vi "Utah Core Audio Test.vi"(11 "Module Config":T9={"Name"="Base Station RF Test", "Parent Q"=refnum, "Is Child?"=FALSE, "Index"=0, "Dirs"={"Root"=path "", "Config"=path "C:/ATE/Config", "Logs"=path "C:/ATE/Logs", "Reports"=path "C:/ATE/Reports", "App Data"=path "C:/ProgramData/MAIN"}, "Simulate"=FALSE, "SimCtrl"=refnum}) -> ()   [LabVIEW 2018]
uses:
  <vilib>/KATE/Queues/Queue Utils.lvlib
  <vilib>/KATE/Module/Module Utils.lvlib
  <vilib>/KATE/Module/Window/Window.Task, Action.ctl
  <vilib>/KATE/Event Log/Event Log.lvlib
  <vilib>/KATE/Scheduler/Scheduler.lvlib
  <vilib>/KATE/Menu/Menu Utils.lvlib
  <vilib>/KATE/Status/Status Utils.lvlib
  Common/Utils/Results/Result.Measurement and Attribute Item Status.ctl
  Common/Utils/Results/Result.Attribute.ctl
  Common/Utils/Results/Result.Limit Type.ctl
  Common/Utils/Results/Result.Numeric.ctl
  <vilib>/KATE/Event Log/Event Notification/Event Notification.lvclass
  <vilib>/KATE/Module/Module.SW Version Info.ctl
  <vilib>/KATE/Event Log/Event Notification/Event Log.Notification Type.ctl
  <vilib>/KATE/Event Log/Event Notification/Event Log.Log Level.ctl
  Common/Utils/Results/Result XML/TestResult.SW Item.ctl
  Common/Utils/TestExec/TestExec.WorkingDir.ctl
  <vilib>/KATE/TCP-IP/Mgr/TCP-IP Mgr.Config.ctl
  <vilib>/KATE/TCP-IP/TCP-IP.lvlib
  Common/Utils/TestExec/TestExec.Test Start Message to Sta.ctl
  <vilib>/KATE/Files/File Utils.lvlib
  Common/Utils/Errors/Error.Error Code List.ctl
  Common/Utils/TestExec/TestExec.Health State Command.ctl
  Common/Utils/Functions/FunctDataMgr/FunctDataMgr.lvclass
  Common/Utils/Results/Result.Results Table Record.ctl
  <vilib>/KATE/Config/Stored Controls/Class.SaveCtrls.lvclass
  <vilib>/KATE/SeqMgr/SeqMgr.Result State Enum.ctl
  <vilib>/KATE/SeqMgr/SeqMgr.lvlib
  <vilib>/KATE/SeqMgr/SeqMgr.Result Info.ctl
  <vilib>/KATE/Config/App Data/Class.AppData.lvclass
  <vilib>/sound2/lvsound2.llb/Sound Data Format.ctl
  <vilib>/sound2/lvsound2.llb/Sound File Write Open.vi
  <vilib>/addons/_NISVFA/_Generation/Signal Generation/SV Discrete Sweep/SV Discrete Sweep.lvclass
  TypeDefs/AudioTest.Result Plot Data.ctl
  <vilib>/sound2/lvsound2.llb/Sound File Write (DBL Single).vi
  <vilib>/KATE/Time/Time Utils.lvlib
  TypeDefs/AudioTest.Config, Limits, Blocked Mic Check.ctl
  TypeDefs/AudioTest.Config, Average Level Config.ctl
  TypeDefs/AudioTest.Config, Sine Sweep Params_V2.ctl
  TypeDefs/AudioTest.Config, Device ID.ctl
  <vilib>/sound2/lvsound2.llb/Sound Output Set Volume (Single).vi
  <vilib>/sound2/lvsound2.llb/Sound Output Write (DBL Single).vi
  <vilib>/sound2/lvsound2.llb/Sampling Mode.ctl
  Common/Utils/Results/Result.Measurement Item.ctl
  <vilib>/sound2/lvsound2.llb/Sound File Write (DBL).vi
  <vilib>/KATE/Queues/Q.Element.ctl
  <vilib>/KATE/Module/Module Config.ctl
  <vilib>/KATE/Module/Module.Working Dirs.ctl
  <vilib>/Utility/miscctls.llb/LVRectTypeDef.ctl
panel:
  in  "Archive Results":bool
  in  "Main Tab":enum32{"Operate", "Maint"}(tab)
  out "TE":bool
  out "Simulate Indication":string="Simulating Instruments"
  in  "Control Tab":enum32{"Test Control", "Config"}(tab)
  in  "Reload Config":bool
  out "Enumerated":bool
  in  "Check UUT Enum Status":bool
  in  "Timeout(s)":dbl=30.0 caption="Time Out(s)" format="%.2f"
  in  "Get Top SN":bool
  in  "Mode":string="Production"
  in  "Run Sweep":bool
  in  "Init UUT Folder":bool
  out "Start Time":timestamp caption="Start\nTime"
  in  "SN":string="ABC123"
  in  "Clear Errors":bool
  in  "Test Reset":bool
  out "Duration(s)":dbl format="%.2g"
  out "Status":string
  in  "Abort":bool
  in  "Result Data Tab":T1(tab)
  in  "UUT Dir":path caption="UUT Folder"
  in  "Open UUT Dir":bool
  in  "Filter":string
  in  "Show Only Failures":bool
  in  "Auto Scroll":bool=TRUE
  out "Results Table":T2[](array[typedef]) caption="Results"
  out "L AvgMag Delta":dbl caption="Delta" format="%.2f"
  out "L AvgMagUnCov":dbl caption="Uncovered" format="%.2f"
  out "L AvgMagCov":dbl caption="Covered" format="%.2f"
  out "R AvgMag Delta":dbl caption="Delta" format="%.2f"
  out "R AvgMagUnCov":dbl caption="Uncovered" format="%.2f"
  out "R AvgMagCov":dbl caption="Covered" format="%.2f"
  out "Right Mic THD":cluster{"F":dbl[], "M":dbl[]}[](graph) caption="Right THD"
  out "Left Mic THD":cluster{"X":dbl[], "Y":dbl[]}[](graph) caption="Left THD"
  out "Right Freq Response":cluster{"frequency":dbl[], "magnitude":dbl[]}[](graph)
  out "Left Freq Response":cluster{"frequency":dbl[], "magnitude":dbl[]}[](graph)
  out "RtThdColor":u32(colorbox)=13816530
  out "RtFRColor":u32(colorbox)=13816530
  out "LFRColor":u32(colorbox)=13816530
  out "LThdColor":u32(colorbox)=13816530
  in  "Raw Time Plots":enum32{"Time", "Covered Mic Mag"}(tab)
  out "Graph Sine Sweep":waveform(dbl)(graph) caption="Stepped Sine Sweep"
  out "Graph Sine Sweep Cal":waveform(dbl)(graph) caption="Stepped Sine Sweep - Calibrated"
  out "Graph Left Covered":waveform(dbl)(graph)
  out "Graph Left Uncovered":waveform(dbl)(graph)
  out "Graph Right Covered":waveform(dbl)(graph)
  out "Graph Right Uncovered":waveform(dbl)(graph)
  out "Right Mic Covered FR":cluster{"F":dbl[], "M":dbl[]}(graph)
  out "Left Mic Covered FR":cluster{"F":dbl[], "M":dbl[]}(graph)
  out "Measurements":path
  out "Result State File":path
  out "Right Mic Covered Raw":path
  out "Right Mic Raw":path
  out "Left Mic Covered Raw":path
  out "Left Mic Raw":path
  out "Sine Sweep Cal":path
  out "Sine Sweep":path
  in  "Undock FW Util":bool
  out "Test Running":bool
  out "Error":errorcluster
  in  "Mic Test Setup":T3
  in  "Clear Graphs":bool
  in  "Clear Raw Data":bool
  in  "Config Tab":enum32{"Microphone Test Setup", "Misc"}(tab)
  in  "Play Tone":bool
  in  "Tone Freq":dbl=1000.0
  in  "Save Wav Files":bool
  in  "Play Volume":dbl(slide)=50.0 scale=0.0..100.0
  in  "SpeakerCalFile":path=path "C:/MTE/Utah Core Audio Test/Config/Microphone Test Speaker Calibration.ini" caption="Speaker Calibration File"
  in  "Limits":T4={"CoveredMicAttn_dB"=30.0, "AvgLevelLL_dBFS"=-30.0, "AvgLevelUL_dBFS"=-10.0, "FreqRespLim"=path "C:/MTE/Utah Core Audio Test/Config/Microphone Test Freq Response Limits.ini", "THDLim"=path "C:/MTE/Utah Core Audio Test/Config/Microphone Test THD Limits.ini"} caption="Test Limits"
  in  "AvgLevelParams":T5={"Freq Start"=500.0, "Freq End"=1200.0} caption="Average Level Calculation"
  in  "Default Data Folder":path=path "C:/MTE/Utah Core Audio Test/Data"
  in  "Sound Devices":T6={"AudioOutName"="Line", "AudioInName"="HMD"}
  in  "Sine Sweep Params":T7={"Duration"=2.54, "Amplitude"=1.0, "FreqStart"=100.0, "FreqEnd"=20000.0, "SampleRate"=44100.0, "StepCnt"=120, "FreqSpacing"=enum."Logarithmic", "Settling"={"Time"=0.0, "Cycles"=1.0}, "Measurement"={"Time"=0.001, "Cycles"=10.0}, "SyncPulseEn"=TRUE} {"Measurement"."Cycles" min=5.0 max=1000.0 step=1.0; "Measurement"."Time" min=0.0 max=5.0 step=0.0001 format="%.3f s"; "Settling"."Cycles" min=0.0 max=100.0 step=0.5; "Settling"."Time" min=0.0 max=5.0 step=0.0001 format="%.3f s"; "StepCnt" min=1; "Amplitude" min=0.0 max=1.0 step=0.1}
  in  "Input Device":i32(ring) items=["Microphone (2- Valve VR Radio & HMD Mic)"]
  in  "Output Device":i32(ring) items=["Speakers (Realtek High Definition Audio)", "Utah (NVIDIA High Definition Audio)", "DELL U3011 (NVIDIA High Definition Audio)", "Realtek Digital Output (Realtek High Definition Audio)", "Realtek Digital Output(Optical) (Realtek High Definition Audio)"]
  in  "Set Audio Output Device Name":bool
  in  "Set Audio Input Device Name":bool
  in  "Stay Open after CLI":bool
  in  "UUT Data Dir":path=path "C:/MTE/Data/X1"
  in  "Sim CLI at Launch":bool
  in  "Run CLI Simulation":bool
  out "R Delta Color":u32(colorbox)=13816530
  out "L Delta Color":u32(colorbox)=13816530
  out "R Level Color":u32(colorbox)=13816530
  out "L Level Color":u32(colorbox)=13816530
  in  "AddTraceInfo":bool caption="Add Trace Info to Errors"
  out "MicTest Dur(s)":dbl=1.0 format="%.2p"
  out "Args":string[](array[string])
  in  "Select Command Line Args":u16(ring) items=["None", "Sweep Left Covered", "Sweep Right Covered", "Sweep Left Uncovered", "Sweep Right Uncovered"]
  in  "Logging Level":T8
  out "App Run Dur(s)":dbl=1.0 format="%.2p"
  out "PlayDur(s)":dbl=1.0 format="%.2p"
  out "Total Samples":i32
  out "Rev":string="v1.0.0"
  out "Error Status":string
  out "Title":string
  in  "Leave Maint":bool
  in  "New Window Bounds":T11={"Left"=212, "Top"=78, "Right"=1444, "Bottom"=899}
  out "Old Window Bounds":T11={"Left"=2142, "Top"=133, "Right"=3354, "Bottom"=889}
  in  "Set Window Bounds":bool
  # "Step                          Name                                                      Value                                    Units      LimType       LL           UL            Result          Code                     Description"
  # "Avg Level:"
  # "dBFS"
  # "dBFS"
  # "dB"
  # "Avg Level:"
  # "dBFS"
  # "dBFS"
  # "dB"
  # "The selected devices are based on the configured Sound Device name lookup."
  # "Volume Check"
  # "Hz"
  # "Relative to Uncovered Mic"
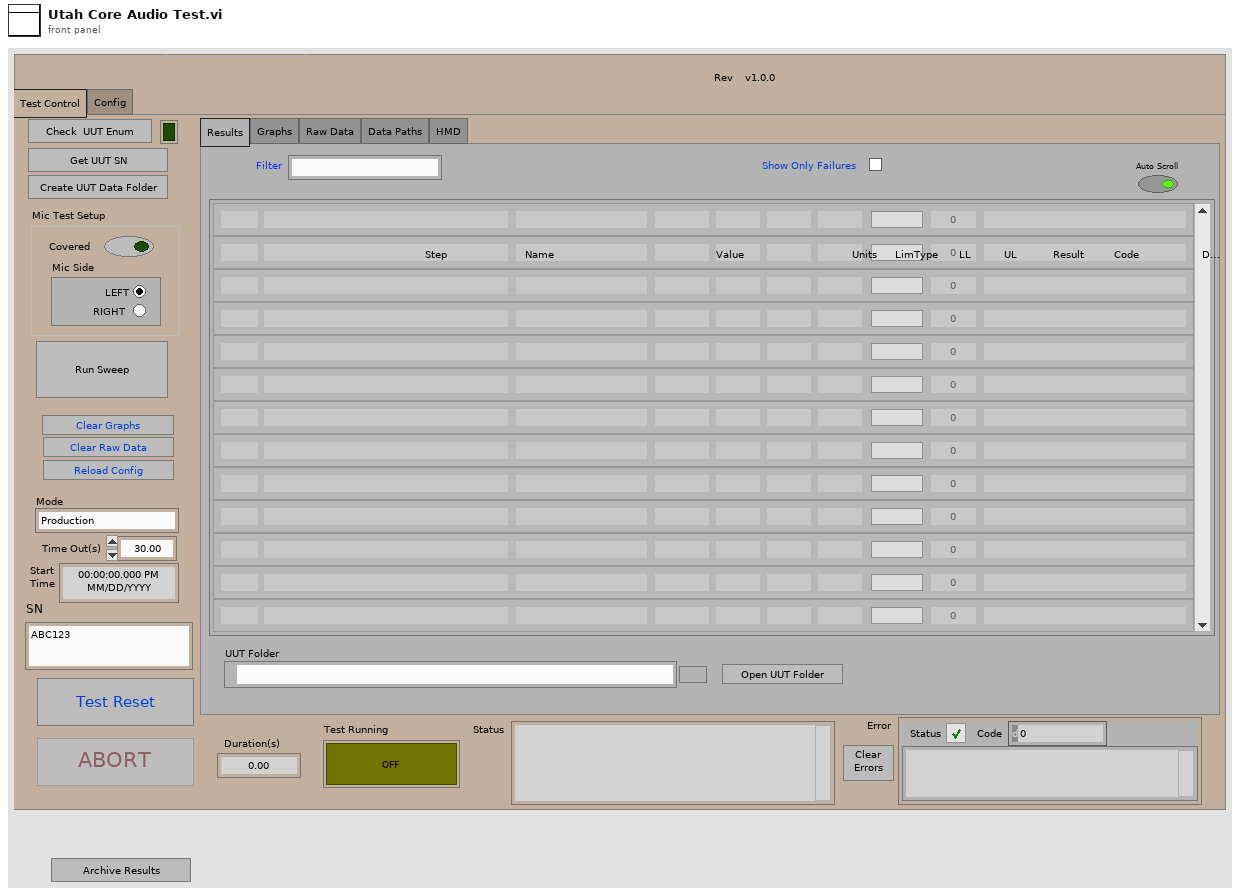
[diagram p1: front panel]
types:
  T1 = enum32{"Results", "Graphs", "Raw Data", "Data Paths", "HMD"}
  T2 = typedef "Result.Results Table Record.ctl" = cluster{"Cnt":i32, "Step":string, "Category":string, "Name":string, "Value":string, "Units":string, "LimType":string, "LL":string, "UL":string, "Status":string, "Status Color":u32, "Code":i32, "Desc":string}
  T3 = cluster{"Mic Side":enum32{"LEFT", "RIGHT"}, "Covered":bool}
  T4 = typedef "AudioTest.Config, Limits, Blocked Mic Check.ctl" = cluster{"CoveredMicAttn_dB":dbl, "AvgLevelLL_dBFS":dbl, "AvgLevelUL_dBFS":dbl, "FreqRespLim":path, "THDLim":path}
  T5 = typedef "AudioTest.Config, Average Level Config.ctl" = cluster{"Freq Start":dbl, "Freq End":dbl}
  T6 = typedef "AudioTest.Config, Device ID.ctl" = cluster{"AudioOutName":string, "AudioInName":string}
  T7 = typedef "AudioTest.Config, Sine Sweep Params_V2.ctl" = cluster{"Duration":dbl, "Amplitude":dbl, "FreqStart":dbl, "FreqEnd":dbl, "SampleRate":dbl, "StepCnt":i32, "FreqSpacing":enum16{"Linear", "Logarithmic"}, "Settling":cluster{"Time":dbl, "Cycles":dbl}, "Measurement":cluster{"Time":dbl, "Cycles":dbl}, "SyncPulseEn":bool}
  T8 = typedef "KATE_Lib.lvlib/Event Log.lvlib/Event Log.Log Level.ctl" = enum16{"Normal", "Verbose", "Debug0", "Debug1", "Debug2"}
  T9 = typedef "KATE_Lib.lvlib/Module Utils.lvlib/Module Config.ctl" = cluster{"Name":string, "Parent Q":refnum<queue>, "Is Child?":bool, "Index":i32, "Dirs":T10, "Simulate":bool, "SimCtrl":refnum<vi>}
  T10 = typedef "KATE_Lib.lvlib/Module Utils.lvlib/Module.Working Dirs.ctl" = cluster{"Root":path, "Config":path, "Logs":path, "Reports":path, "App Data":path}
  T11 = typedef "LVRectTypeDef.ctl" = cluster{"Left":i16, "Top":i16, "Right":i16, "Bottom":i16}
  T12 = typedef "KATE_Lib.lvlib/Module Utils.lvlib/Module.SW Version Info.ctl" = cluster{"AppName":string, "Company":string, "Version":string, "Description":string, "PN":string}
  T13 = typedef "KATE_Lib.lvlib/Module Utils.lvlib/Module Sys Info.ctl" = cluster{"Main Q":refnum<queue>, "Exe":bool, "SW Rev":T12, "Self Ref":refnum<vi>, "Main Tab":refnum<vi>, "Pane":refnum<vi>, "Stop":cluster{"Ref":refnum<event-registration>, "Event":refnum<user-event>}, "Cfg":T9, "Services":cluster{"Name":string, "vi ref":refnum<vi>}[], "Menu Ref":refnum<k9>, "CtrlStates":refnum<class "Class.SaveCtrls.lvclass">, "Docs":cluster{"Tags":string[], "Paths":path[]}, "Log":refnum<class "Event Notification.lvclass">, "Test Controls":refnum<vi>[], "Child Modules":cluster{"Name":string, "vi ref":refnum<vi>}[], "SW Items":string[][], "AppData":refnum<class "Class.AppData.lvclass">, "Subscriptions":refnum<class "Subscription.lvclass">}
  T14 = enum32{"Invalid", "Standard", "Closed", "Hidden", "Minimized", "Maximized"}
  T15 = typedef "KATE_Lib.lvlib/TCP-IP.lvlib/TCP-IP Mgr.Config.ctl" = cluster{"IP":string, "Port":u16, "Listener":bool, "Enable":bool}
  T16 = typedef "TestResult.SW Item.ctl" = cluster{"Name":string, "PN":string, "Version":string, "Note":string}
  T17 = typedef "Result.Measurement Item.ctl" = cluster{"Cnt":i32, "Step":string, "Category":string, "Name":string, "Value":string, "Units":string, "LimType":string, "LL":string, "UL":string, "Status":T18, "Code":i32, "Desc":string, "Time":timestamp}
  T18 = typedef "Result.Measurement and Attribute Item Status.ctl" = i32
  T19 = enum8{"Enabled", "Disabled", "Disabled and Grayed Out"}
  T20 = typedef "KATE_Lib.lvlib/Module Utils.lvlib/Window.Task, Action.ctl" = enum16{"Resize()", "Show Panel(Bool)", "Show Scroll Bars(Bool)", "Dock to SubPanel(SubPanel Ref)", "Undock from SubPanel()", "Return to SubPanel()", "Go To Maint Tab()", "Show Maint Tab(Bool)", "Open Block Diagram()"}
  T21 = typedef "Sound Data Format.ctl" = cluster{"sample rate (S/s)":dbl, "number of channels":i32, "bits per sample":i32}
  T22 = typedef "AudioTest.Result Plot Data.ctl" = cluster{"Order":i32, "Name":string, "X":dbl[], "Y":dbl[], "X Units":string, "Y Units":string, "LimitType":enum16{"None", "LL", "UL"}, "FailCode":i32, "FailDesc":string, "Ref Data Name":string, "Result Name":string, "0dB Level":dbl, "Normalized":bool}
  T23 = enum16{"open", "replace", "create", "open or create", "replace or create", "replace or create with confirmation"}
  T24 = cluster{"Active":bool, "Test":string, "Args":string[]}
  T25 = cluster{"Devices":T6, "SweepParams":T7, "DataFolder":path, "AvgLevelParams":T5, "BlockedMicLim":T4, "SpeakerCalFile":path, "Volume":dbl}
  T26 = typedef "TestExec.WorkingDir.ctl" = cluster{"Name":string, "Path":path}
  T27 = typedef "TestExec.Test Start Message to Sta.ctl" = cluster{"Test Name":string, "Start Time":timestamp, "UUT SN":string}
  T28 = typedef "KATE_Lib.lvlib/Event Log.lvlib/Event Log.Notification Type.ctl" = enum16{"Normal", "Warning", "Error", "Success"}
  T29 = typedef "Result.Attribute.ctl" = cluster{"Cnt":i32, "Step":string, "Category":string, "Name":string, "Value":string, "Status":T18, "Code":i32, "Desc":string, "Time":timestamp}
  T30 = typedef "Result.Numeric.ctl" = cluster{"Cnt":i32, "Step":string, "Category":string, "Name":string, "Value":dbl, "Units":string, "LimType":T31, "LL":dbl, "UL":dbl, "Status":T18, "Code":i32, "Desc":string, "Time":timestamp}
  T31 = typedef "Result.Limit Type.ctl" = enum16{"None", "EQ", "NE", "GT", "LT", "GE", "LE", "GTLT", "GELE", "GELT", "GTLE", "LTGT", "LEGE", "LEGT", "LTGE", "Contains", "NotContains"}
  T32 = typedef "TestExec.Health State Command.ctl" = enum16{"Update", "Clear All", "Clear Warnings", "Clear Errors", "Set Warning", "Set Error"}
  T33 = typedef "KATE_Lib.lvlib/SeqMgr.lvlib/SeqMgr.Result Info.ctl" = cluster{"State":T34, "Code":i32, "Description":string}
  T34 = typedef "KATE_Lib.lvlib/SeqMgr.lvlib/SeqMgr.Result State Enum.ctl" = enum16{"None", "Passing", "Failing", "PASS", "FAIL", "ABORT", "ERROR"}
  T35 = cluster{"Archive":path, "ArchiveSum":path, "Temp Data":path, "UUTDir":path}
  T36 = cluster{"Lnch":bool, "FunctData":refnum<class "FunctDataMgr.lvclass">, "Timeout(s)":dbl, "Dirs":cluster{"Archive":path, "ArchiveSum":path, "Temp Data":path, "UUTDir":path}, "SN_Time":string, "Remote Test":bool, "ResultState":T33, "StaVer":i32, "CL Args":cluster{"Active":bool, "Test":string, "Args":string[]}, "FR Lim":cluster{"LL":T22, "UL":T22}, "THD Lim":cluster{"LL":T22, "UL":T22}, "Rslt":cluster{"Meas":T17[]}, "SavWav":bool}
  T37 = typedef "Error.Error Code List.ctl" = i32
  T38 = cluster{"Sweep":waveform(dbl), "SweepCal":waveform(dbl), "Mic":waveform(dbl), "SmplCnt":i32, "SigConfig":refnum<class "SV Discrete Sweep.lvclass">, "AvgMag":dbl, "Mag":cluster{"F":dbl[], "M":dbl[]}, "THD":cluster{"F":dbl[], "M":dbl[]}, "TestName":string, "Start":dbl}
  T39 = typedef "Sound File Refnum.ctl" = refnum<file>
  T40 = typedef "Sampling Mode.ctl" = i32
  T41 = typedef "Sound Output Task ID.ctl" = u32
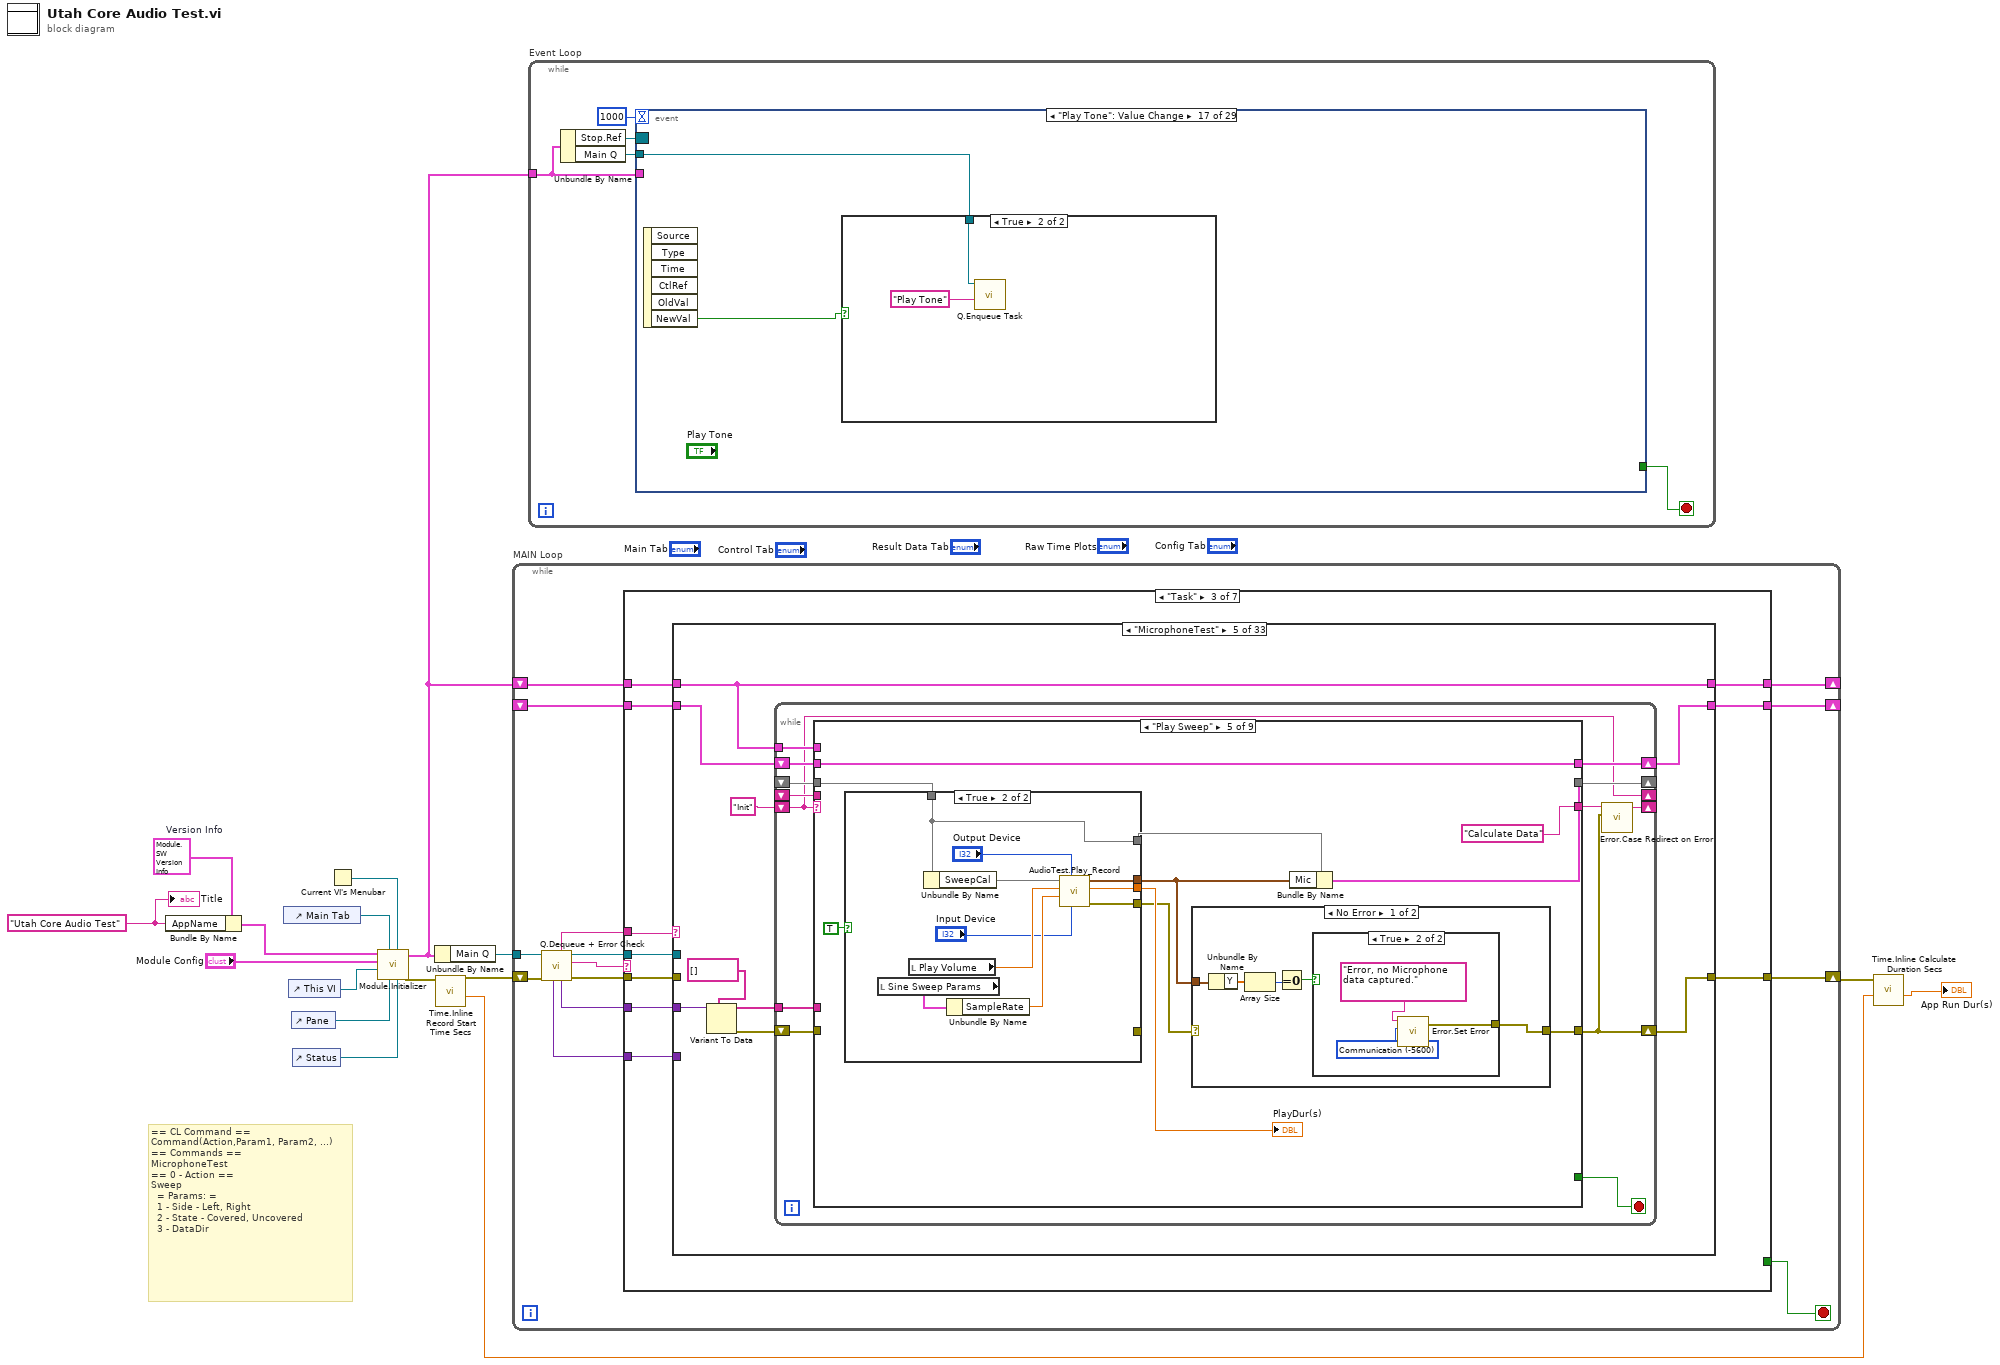
[diagram p0: block diagram]
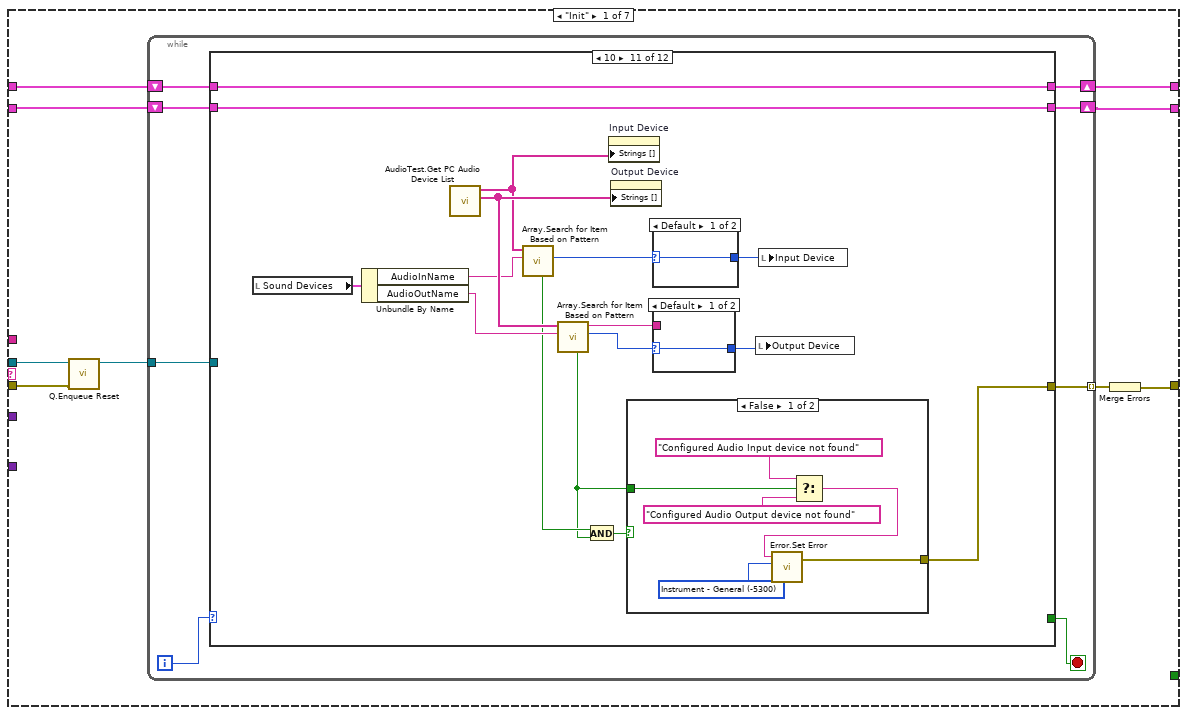
[diagram p2: hidden frame]
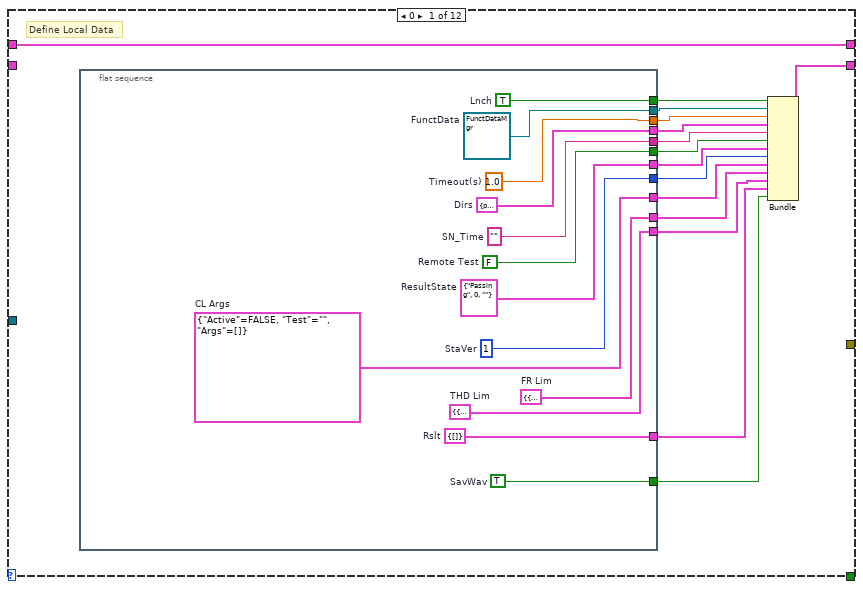
[diagram p3: hidden frame]
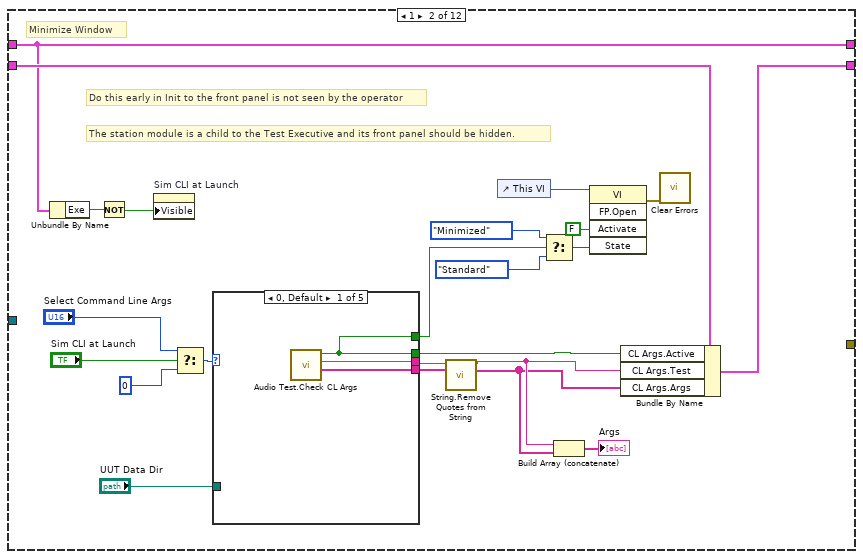
[diagram p4: hidden frame]
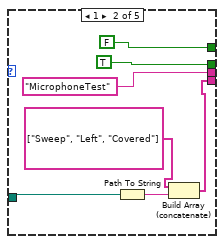
[diagram p5: hidden frame]
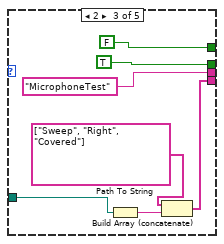
[diagram p6: hidden frame]
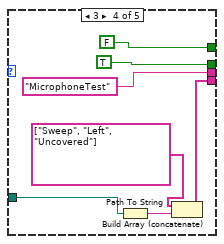
[diagram p7: hidden frame]
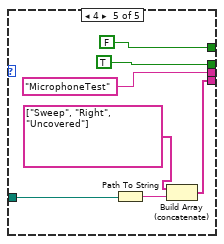
[diagram p8: hidden frame]
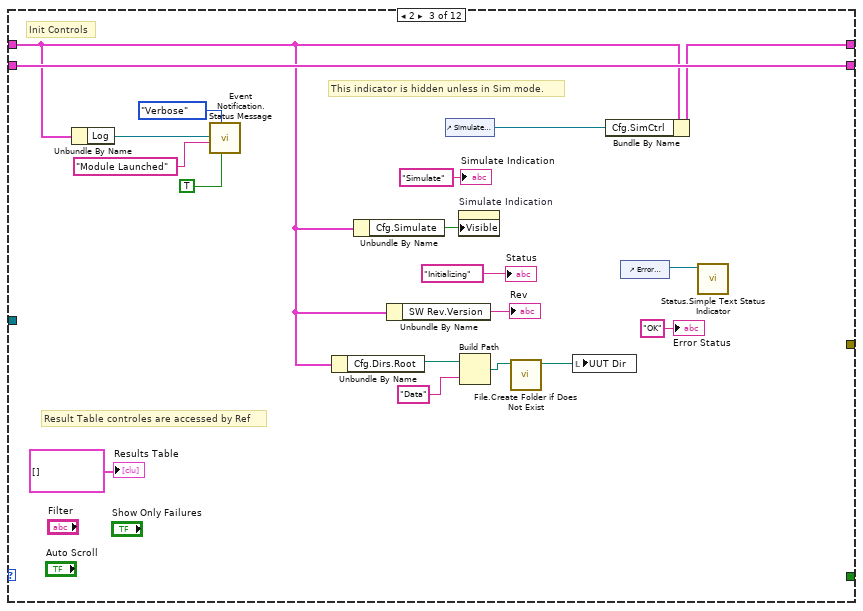
[diagram p9: hidden frame]
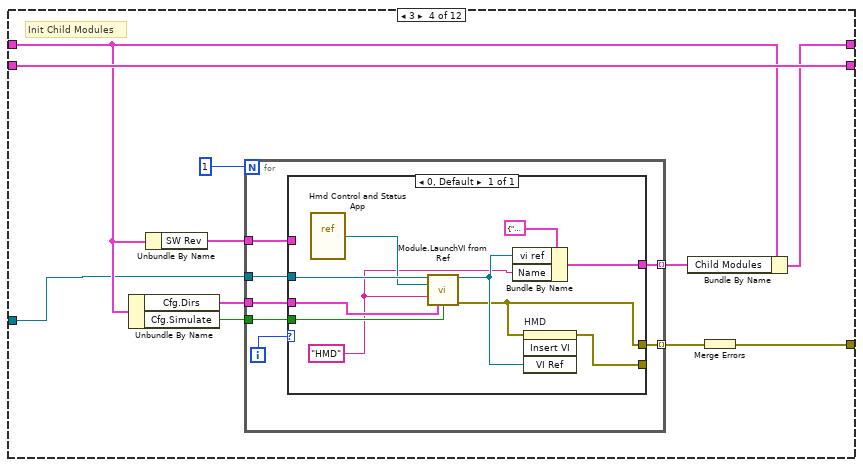
[diagram p10: hidden frame]
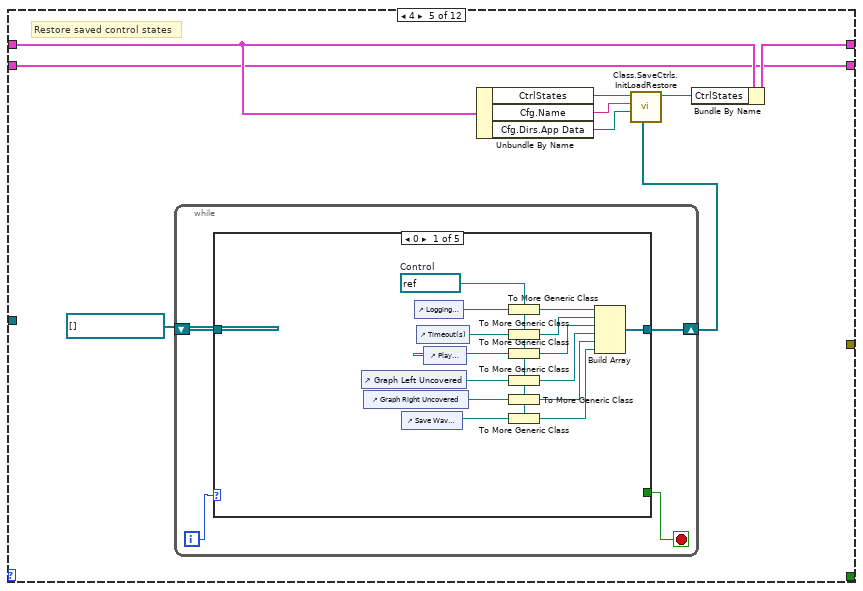
[diagram p11: hidden frame]
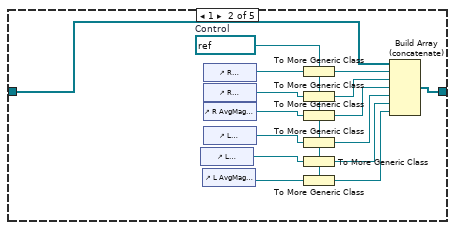
[diagram p12: hidden frame]
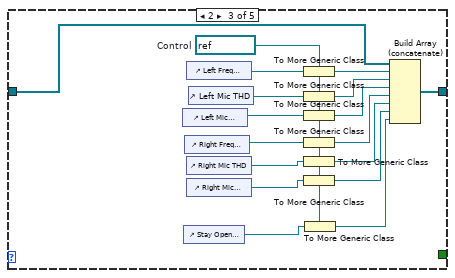
[diagram p13: hidden frame]
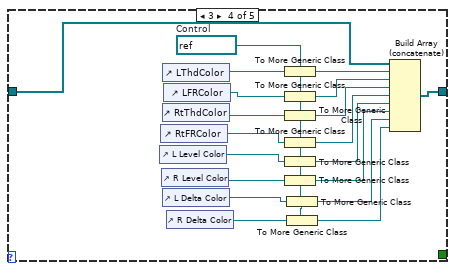
[diagram p14: hidden frame]
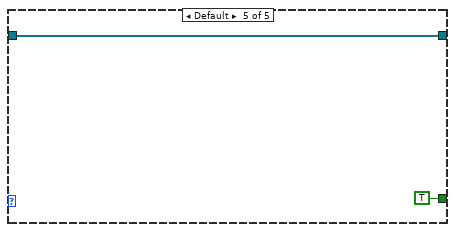
[diagram p15: hidden frame]
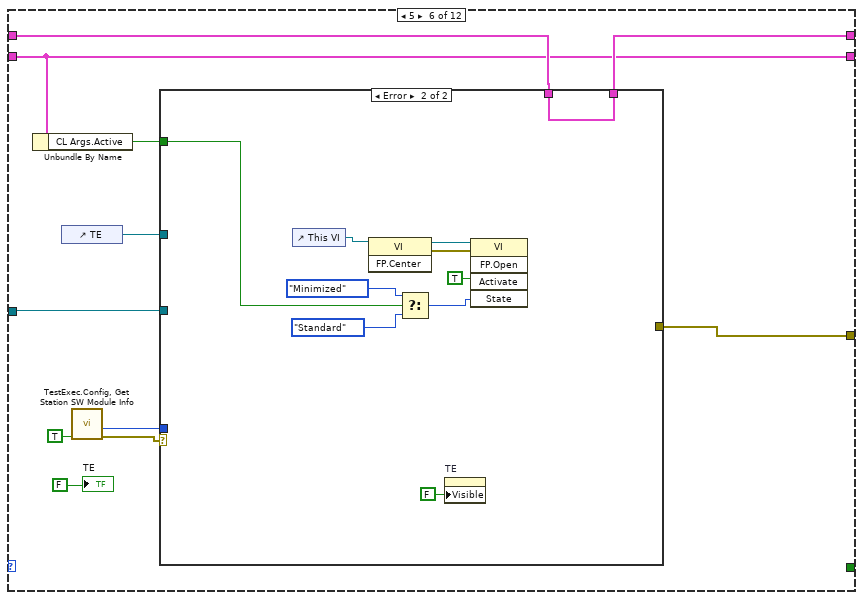
[diagram p16: hidden frame]
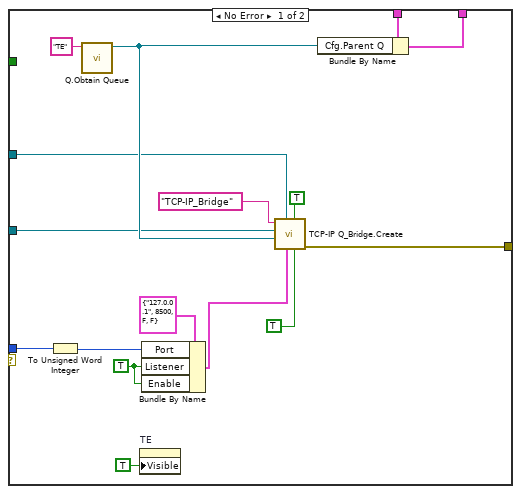
[diagram p17: hidden frame]
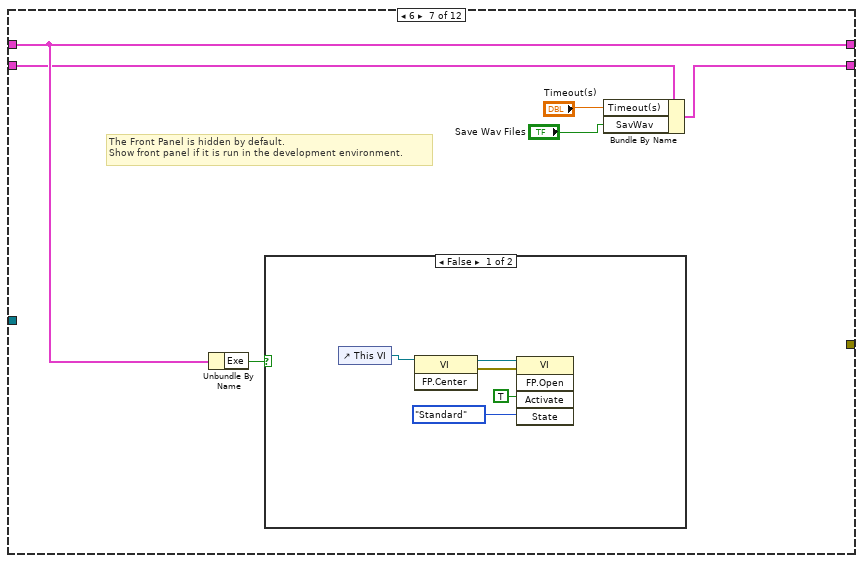
[diagram p18: hidden frame]
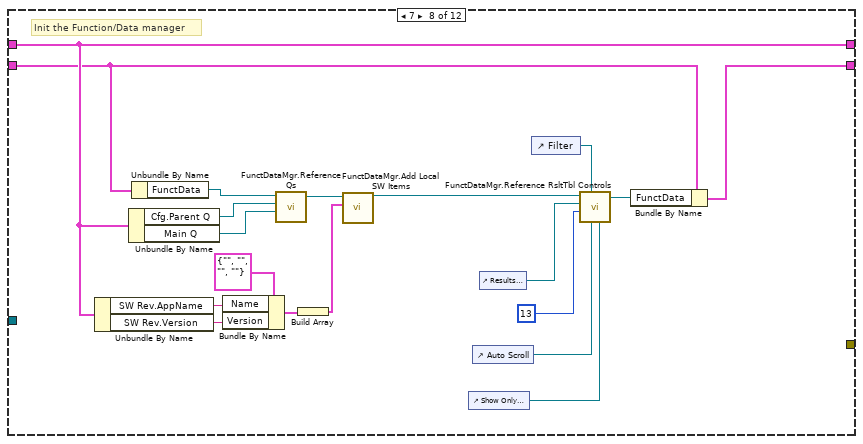
[diagram p20: hidden frame]
diagram:
  w11 = T12 {"AppName"="ModuleX", "Company"="CompanyX", "Version"="1.0", "Description"="This app is being developed.", "PN"=""}  # Version Info
  w8 = "Utah Core Audio Test"
  # "== CL Command ==\nCommand(Action,Param1, Param2, ...)\n== Commands ==\nMicrophoneTest\n== 0 - Action ==\nSweep\n  = Params: =\n  1 - Side - Left, Right\n  2 - State - Covered, Uncovered\n  3 - DataDir"
  n1 = Bundle By Name(cluster=w11, "AppName"=w8) -> (w10:T12)
  n2 = control-ref of="Main Tab"() -> (w16:refnum<vi>)
  n3 = control-ref of="This VI"() -> (w15:refnum<vi>)
  n4 = control-ref of="Pane"() -> (w14:refnum<vi>)
  n5 = control-ref of="Status"() -> (w9:refnum<vi>)
  n6 = Current VI's Menubar() -> (w13:refnum<k9>)
  n7 = call <vilib>:"Module.Initializer.vi"("StatusTxtBx"=w9, "Menu Ref"=w13, "Pane"=w14, "Main Tab"=w16, "Self Ref"=w15, "Module Config"="Module Config", "SW Rev"=w10) -> ("error out"=w3:errorcluster, "Sys"=w6:T13)  [unwired: 3 in]
  n8 = Unbundle By Name(w6) -> ("Main Q"=w7:refnum<queue>)
  n9 = call <vilib>:"Time.Inline Record Start Time Secs.vi"("Error In Upper"=w3) -> ("Start(s)"=w1:dbl, "Error Out Upper"=w2:errorcluster)  [unwired: 8 in, 1 out]
  n10 = while "MAIN Loop" {
    shift-right: [w26] -> w5
    shift-left: w2 -> [w24]
    shift-right: [w27] -> _
    shift-left: _ -> [w30]
    shift-right: [w28] -> _
    shift-left: w6 -> [w29]
    tunnel: w7 -> [w23]
    stop <- w19 stop-if-true
    n11 = call <vilib>:"Q.Dequeue + Error Check.vi"("Error In"=w24, "Q In"=w23) -> ("error out"=w25:errorcluster, "Cmd"=w18:string, "Q Out"=w22:refnum<queue>, "Data1"=w21:variant, "Sub"=w17:string, "Data2"=w20:variant)  [unwired: 4 in]
    n12 = case shown="\"Task\"" w18 {
      selector: w18 -> [_ _ _ _ _ w1970 _]
      tunnel: w30 -> [w35 w390 w452 w1717 w1918 w1976 w2025]
      tunnel: w29 -> [w37 w391 w453 w1718 w1919 w1975 w2021]
      tunnel: [w36 w389 w451 w1716 w1917 w1975 w2022] -> w28
      tunnel: [w34 w388 w450 w1715 w1916 w1974 w2025] -> w27
      tunnel: [w31 _ w444 w1713 _ w1973 w2027] -> w26
      tunnel: w25 -> [w38 _ w446 w1714 _ w1969 _]
      tunnel: w22 -> [w39 w387 w447 w1711 w1922 w1972 _]
      tunnel: w21 -> [_ _ w448 w1710 w1921 w1968 _]
      tunnel: w20 -> [_ _ w445 w1709 w1920 _ _]
      tunnel: w17 -> [_ _ w449 w1712 w1923 w1971 _]
      tunnel: [_ _ _ _ _ _ TRUE] -> w19
      frame "Init" {
        n13 = call <vilib>:"Q.Enqueue Reset.vi"("Error In"=w38, "Q In"=w39) -> ("Q Out"=w33:refnum<queue>)  [unwired: 8 in, 1 out]
        n14 = while {
          shift-right: [w46] -> w36
          shift-left: w37 -> [w47]
          shift-right: [w44] -> w34
          shift-left: w35 -> [w45]
          tunnel: w33 -> [w42]
          tunnel: [w41] -> w32 mode=indexing
          i -> [w40]
          stop <- w43 stop-if-true
          n15 = case shown="10" w40 {
            tunnel: w47 -> [w62 w78 w131 w151 w181 w261 w298 w310 w346 w357 w373 w386]
            tunnel: [w62 w78 w140 w152 w180 w260 w298 w310 w346 w357 w373 w386] -> w46
            tunnel: w45 -> [_ w79 w148 w159 w179 w258 w297 w307 w345 w356 w372 w385]
            tunnel: [w61 w95 w148 w159 w179 w258 w296 w308 w344 w356 w372 w385] -> w44
            tunnel: [_ _ _ _ _ _ _ _ _ _ _ TRUE] -> w43
            tunnel: w42 -> [_ _ _ w150 _ w262 _ _ _ w353 _ _]
            tunnel: [_ _ _ w153 _ w259 _ _ w334 _ w358 _] -> w41
            frame 0 {
              # "Define Local Data"
              n16 = flat-sequence {
                tunnel: [w75] -> w60
                tunnel: [w74] -> w59
                tunnel: [w73] -> w58
                tunnel: [w72] -> w57
                tunnel: [w71] -> w56
                tunnel: [w70] -> w55
                tunnel: [w69] -> w54
                tunnel: [w68] -> w53
                tunnel: [w67] -> w52
                tunnel: [w66] -> w51
                tunnel: [w65] -> w50
                tunnel: [w64] -> w49
                tunnel: [w63] -> w48
                frame #0 {
                  w63 = TRUE  # SavWav
                  w64 = cluster{"Meas":T17[]} {"Meas"=[]}  # Rslt
                  w65 = cluster{"LL":T22, "UL":T22} {"LL"={"Order"=0, "Name"="", "X"=[], "Y"=[], "X Units"="", "Y Units"="", "LimitType"=enum."None", "FailCode"=0, "FailDesc"="", "Ref Data Name"="", "Result Name"="", "0dB Level"=0.0, "Normalized"=FALSE}, "UL"={"Order"=0, "Name"="", "X"=[], "Y"=[], "X Units"="", "Y Units"="", "LimitType"=enum."None", "FailCode"=0, "FailDesc"="", "Ref Data Name"="", "Result Name"="", "0dB Level"=0.0, "Normalized"=FALSE}}  # THD Lim
                  w66 = cluster{"LL":T22, "UL":T22} {"LL"={"Order"=0, "Name"="", "X"=[], "Y"=[], "X Units"="", "Y Units"="", "LimitType"=enum."None", "FailCode"=0, "FailDesc"="", "Ref Data Name"="", "Result Name"="", "0dB Level"=0.0, "Normalized"=FALSE}, "UL"={"Order"=0, "Name"="", "X"=[], "Y"=[], "X Units"="", "Y Units"="", "LimitType"=enum."None", "FailCode"=0, "FailDesc"="", "Ref Data Name"="", "Result Name"="", "0dB Level"=0.0, "Normalized"=FALSE}}  # FR Lim
                  w67 = T24 {"Active"=FALSE, "Test"="", "Args"=[]}  # CL Args
                  w68 = 1  # StaVer
                  w69 = T33 {"State"=enum."Passing", "Code"=0, "Description"=""}  # ResultState
                  w70 = FALSE  # Remote Test
                  w71 = ""  # SN_Time
                  w74 = refnum<class "FunctDataMgr.lvclass"> refnum  # FunctData
                  w72 = T35 {"Archive"=path "", "ArchiveSum"=path "", "Temp Data"=path "", "UUTDir"=path ""}  # Dirs
                  w73 = 1.0  # Timeout(s)
                  w75 = TRUE  # Lnch
                }
              }
              n17 = Bundle("Lnch"=w60, "FunctData"=w59, "Timeout(s)"=w58, "Dirs"=w57, "SN_Time"=w56, "Remote Test"=w55, "ResultState"=w54, "StaVer"=w53, "CL Args"=w52, "FR Lim"=w51, "THD Lim"=w50, "Rslt"=w49, "SavWav"=w48) -> (w61:T36)  [unwired: 1 in]
            }
            frame 1 {
              # "The station module is a child to the Test Executive and its front panel should be hidden."
              # "Do this early in Init to the front panel is not seen by the operator"
              # "Minimize Window"
              n18 = Unbundle By Name(w78) -> ("Exe"=w77:bool)
              n19 = Not(x=w77) -> (.not. x?=w76:bool)
              n20 = property on="Sim CLI at Launch" class="Bool (strict)"("Visible"=w76) -> ()  [unwired: 2 in, 2 out]
              n21 = Select(t="Select Command Line Args", s="Sim CLI at Launch", f=u16 0) -> (s? t:f=w88:u16)
              n22 = case shown="0, Default" w88 {
                tunnel: [w101 "MicrophoneTest" ("Action") "MicrophoneTest" ("Action") "MicrophoneTest" ("Action") "MicrophoneTest" ("Action")] -> w85
                tunnel: [w100 w103 w109 w117 w123] -> w84
                tunnel: [w99 TRUE ("CmdLine") TRUE ("CmdLine") TRUE ("CmdLine") TRUE ("CmdLine")] -> w80
                tunnel: [w99 FALSE ("CmdLine") FALSE ("CmdLine") FALSE ("CmdLine") FALSE ("CmdLine")] -> w91
                tunnel: "UUT Data Dir" -> [_ w102 w111 w116 w124]
                frame 0, Default {
                  n23 = call "Audio Test.Check CL Args.vi"() -> ("Args"=w100:string[], "Action"=w101:string, "CmdLine"=w99:bool)  [unwired: 9 in]
                }
                frame 1 {
                  n24 = Path To String(path=w102) -> (string=w105:string)
                  n25 = Build Array (concatenate)(string[] ["Sweep", "Left", "Covered"], w105) -> (w103:string[])
                }
                frame 2 {
                  n26 = Path To String(path=w111) -> (string=w112:string)
                  n27 = Build Array (concatenate)(string[] ["Sweep", "Right", "Covered"], w112) -> (w109:string[])
                }
                frame 3 {
                  n28 = Path To String(path=w116) -> (string=w119:string)
                  n29 = Build Array (concatenate)(string[] ["Sweep", "Left", "Uncovered"], w119) -> (w117:string[])
                }
                frame 4 {
                  n30 = Path To String(path=w124) -> (string=w126:string)
                  n31 = Build Array (concatenate)(string[] ["Sweep", "Right", "Uncovered"], w126) -> (w123:string[])
                }
              }
              n32 = call "String.Remove Quotes from String.vi"("1D String In"=w84, "String In"=w85) -> ("1D String without Quotes"=w82:string[], "String without Quotes"=w83:string)  [unwired: 7 in, 1 out]
              n33 = control-ref of="This VI"() -> (w97:refnum<vi>)
              n34 = Select(t=T14."Minimized" ("State"), s=w91, f=T14."Standard" ("State")) -> (s? t:f=w92:T14)
              n35 = Build Array (concatenate)(w83, w82) -> (→"Args":string[])
              n36 = invoke class="VI" method="FP.Open"(reference=w97, "Activate"=FALSE ("Activate?"), "State"=w92) -> (error out=w96:errorcluster)  [unwired: 2 in, 4 out]
              n37 = Bundle By Name(cluster=w79, "CL Args.Active"=w80, "CL Args.Test"=w83, "CL Args.Args"=w82) -> (w95:T36)
              n38 = call <vilib>:"Clear Errors.vi"("error in (no error)"=w96) -> ()  [unwired: 5 in, 2 out]
            }
            frame 2 {
              # "Init Controls"
              # "This indicator is hidden unless in Sim mode."
              # "Result Table controles are accessed by Ref"
              n39 = Unbundle By Name(w131) -> ("Log"=w146:refnum<class "Event Notification.lvclass">)
              n40 = call <vilib>:"Event Notification.Status Message.vi"("Log"=TRUE, "Level"=Event_Log.Log_Level."Verbose", "Message"="Module Launched", "Event Notification in"=w146) -> ()  [unwired: 8 in]
              n41 = Unbundle By Name(w131) -> ("Cfg.Dirs.Root"=w135:path)
              n42 = Unbundle By Name(w131) -> ("Cfg.Simulate"=w130:bool)
              n43 = Unbundle By Name(w131) -> ("SW Rev.Version"=→"Rev":string)
              n44 = control-ref of="Simulate Indication"() -> (w141:refnum<vi>)
              n45 = property on="Simulate Indication" class="Str"("Visible"=w130) -> ()  [unwired: 2 in, 2 out]
              n46 = Build Path(base path=w135, name or relative path="Data") -> (appended path=w133:path)
              n47 = call <vilib>:"File.Create Folder if Does Not Exist.vi"("Path"=w133) -> ("Dup Path"=w132:path)  [unwired: 8 in, 2 out]
              n48 = local write "UUT Dir"(w132) -> ()
              n49 = Bundle By Name(cluster=w131, "Cfg.SimCtrl"=w141) -> (w140:T13)
              n50 = control-ref of="Error Status"() -> (w139:refnum<vi>)
              n51 = call <vilib>:"Status.Simple Text Status Indicator.vi"("Status TextBox"=w139) -> ()  [unwired: 10 in, 1 out]
              "Results Table" <- T2[] [] ("Results Table")
              "Simulate Indication" <- "Simulate" ("Simulate Indication")
              "Status" <- "Initializing" ("Status")
              "Error Status" <- "OK" ("Error Status")
            }
            frame 3 {
              # "Init Child Modules"
              n52 = Unbundle By Name(w151) -> ("Cfg.Dirs"=w156:T10, "Cfg.Simulate"=w157:bool)
              n53 = Unbundle By Name(w151) -> ("SW Rev"=w155:T12)
              n54 = for {
                N: 1 -> [_]
                tunnel: w155 -> [w166]
                tunnel: [w161] -> w149 mode=indexing
                tunnel: w150 -> [w164]
                tunnel: w156 -> [w163]
                tunnel: w157 -> [w162]
                tunnel: [w160] -> w158 mode=indexing
                i -> [w165]
                n55 = case shown="0, Default" w165 {
                  tunnel: w166 -> [_]
                  tunnel: w164 -> [w176]
                  tunnel: w163 -> [w172]
                  tunnel: w162 -> [w171]
                  tunnel: [w174] -> w161
                  tunnel: [w168] -> w160
                  tunnel: [w167] -> _
                  frame 0, Default {
                    w169 = "HMD"
                    n56 = vi-ref "Hmd Control and Status App.vi"() -> (w175:refnum<vi>)
                    n57 = call <vilib>:"Module.LaunchVI from Ref.vi"("Parent Q"=w176, "VI Ref In"=w175, "Q Name"=w169, "Working Dirs"=w172, "Simulate"=w171) -> ("VI Ref Out"=w173:refnum<vi>, "error out"=w168:errorcluster)  [unwired: 8 in, 1 out]
                    n58 = Bundle By Name(cluster=cluster{"Name":string, "vi ref":refnum<vi>} {"Name"="", "vi ref"=refnum} ("Service"), "vi ref"=w173, "Name"=w169) -> (w174:cluster{"Name":string, "vi ref":refnum<vi>})
                    n59 = invoke on="HMD" class="SubPnl" method="Insert VI"(error in=w168, "VI Ref"=w173) -> (error out=w167:errorcluster)  [unwired: 2 in, 3 out]
                  }
                }
              }
              n60 = Bundle By Name(cluster=w151, "Child Modules"=w149) -> (w152:T13)
              n61 = Merge Errors(w158) -> (w153:errorcluster)
            }
            frame 4 {
              # "Restore saved control states"
              n62 = while {
                shift-right: [w189] -> w177
                shift-left: refnum<vi>[] [] -> [w186]
                i -> [w188]
                stop <- w187 stop-if-true
                n63 = case shown="0" w188 {
                  tunnel: [w192 w211 w229 w248 w255] -> w189
                  tunnel: [_ _ _ _ TRUE] -> w187
                  tunnel: w186 -> [_ w204 w219 w236 w255]
                  frame 0 {
                    w193 = refnum<vi> refnum  # Control
                    n64 = control-ref of="Graph Left Uncovered"() -> (w202:refnum<vi>)
                    n65 = control-ref of="Graph Right Uncovered"() -> (w191:refnum<vi>)
                    n66 = control-ref of="Save Wav Files"() -> (w190:refnum<vi>)
                    n67 = control-ref of="Logging Level"() -> (w194:refnum<vi>)
                    n68 = control-ref of="Timeout(s)"() -> (w198:refnum<vi>)
                    n69 = control-ref of="Play Volume"() -> (w203:refnum<vi>)
                    n70 = To More Generic Class(target class=w193, reference=w194) -> (generic class reference=w196:refnum<vi>)
                    n71 = To More Generic Class(target class=w193, reference=w198) -> (generic class reference=w195:refnum<vi>)
                    n72 = To More Generic Class(target class=w193, reference=w203) -> (generic class reference=w197:refnum<vi>)
                    n73 = To More Generic Class(target class=w193, reference=w202) -> (generic class reference=w199:refnum<vi>)
                    n74 = To More Generic Class(target class=w193, reference=w191) -> (generic class reference=w200:refnum<vi>)
                    n75 = To More Generic Class(target class=w193, reference=w190) -> (generic class reference=w201:refnum<vi>)
                    n76 = Build Array(w196, w195, w197, w199, w200, w201) -> (w192:refnum<vi>[])
                  }
                  frame 1 {
                    w212 = refnum<vi> refnum  # Control
                    n77 = control-ref of="L AvgMagCov"() -> (w206:refnum<vi>)
                    n78 = control-ref of="L AvgMag Delta"() -> (w205:refnum<vi>)
                    n79 = control-ref of="R AvgMagUnCov"() -> (w210:refnum<vi>)
                    n80 = control-ref of="R AvgMagCov"() -> (w209:refnum<vi>)
                    n81 = control-ref of="R AvgMag Delta"() -> (w208:refnum<vi>)
                    n82 = control-ref of="L AvgMagUnCov"() -> (w207:refnum<vi>)
                    n83 = To More Generic Class(target class=w212, reference=w210) -> (generic class reference=w214:refnum<vi>)
                    n84 = To More Generic Class(target class=w212, reference=w209) -> (generic class reference=w213:refnum<vi>)
                    n85 = To More Generic Class(target class=w212, reference=w208) -> (generic class reference=w215:refnum<vi>)
                    n86 = To More Generic Class(target class=w212, reference=w207) -> (generic class reference=w216:refnum<vi>)
                    n87 = To More Generic Class(target class=w212, reference=w206) -> (generic class reference=w217:refnum<vi>)
                    n88 = To More Generic Class(target class=w212, reference=w205) -> (generic class reference=w218:refnum<vi>)
                    n89 = Build Array (concatenate)(w204, w214, w213, w215, w216, w217, w218) -> (w211:refnum<vi>[])
                  }
                  frame 2 {
                    w221 = refnum<vi> refnum  # Control
                    n90 = control-ref of="Left Mic Covered FR"() -> (w226:refnum<vi>)
                    n91 = control-ref of="Stay Open after CLI"() -> (w222:refnum<vi>)
                    n92 = control-ref of="Right Freq Response"() -> (w225:refnum<vi>)
                    n93 = control-ref of="Left Freq Response"() -> (w228:refnum<vi>)
                    n94 = control-ref of="Right Mic THD"() -> (w224:refnum<vi>)
                    n95 = control-ref of="Right Mic Covered FR"() -> (w223:refnum<vi>)
                    n96 = control-ref of="Left Mic THD"() -> (w227:refnum<vi>)
                    n97 = To More Generic Class(target class=w221, reference=w228) -> (generic class reference=w231:refnum<vi>)
                    n98 = To More Generic Class(target class=w221, reference=w227) -> (generic class reference=w230:refnum<vi>)
                    n99 = To More Generic Class(target class=w221, reference=w226) -> (generic class reference=w232:refnum<vi>)
                    n100 = To More Generic Class(target class=w221, reference=w225) -> (generic class reference=w233:refnum<vi>)
                    n101 = To More Generic Class(target class=w221, reference=w224) -> (generic class reference=w234:refnum<vi>)
                    n102 = To More Generic Class(target class=w221, reference=w223) -> (generic class reference=w235:refnum<vi>)
                    n103 = To More Generic Class(target class=w221, reference=w222) -> (generic class reference=w220:refnum<vi>)
                    n104 = Build Array (concatenate)(w219, w231, w230, w232, w233, w234, w235, w220) -> (w229:refnum<vi>[])
                  }
                  frame 3 {
                    w245 = refnum<vi> refnum  # Control
                    n105 = control-ref of="L Level Color"() -> (w240:refnum<vi>)
                    n106 = control-ref of="RtFRColor"() -> (w241:refnum<vi>)
                    n107 = control-ref of="R Level Color"() -> (w239:refnum<vi>)
                    n108 = control-ref of="LThdColor"() -> (w244:refnum<vi>)
                    n109 = control-ref of="RtThdColor"() -> (w242:refnum<vi>)
                    n110 = control-ref of="L Delta Color"() -> (w238:refnum<vi>)
                    n111 = control-ref of="LFRColor"() -> (w243:refnum<vi>)
                    n112 = control-ref of="R Delta Color"() -> (w237:refnum<vi>)
                    n113 = To More Generic Class(target class=w245, reference=w244) -> (generic class reference=w250:refnum<vi>)
                    n114 = To More Generic Class(target class=w245, reference=w243) -> (generic class reference=w249:refnum<vi>)
                    n115 = To More Generic Class(target class=w245, reference=w242) -> (generic class reference=w251:refnum<vi>)
                    n116 = To More Generic Class(target class=w245, reference=w241) -> (generic class reference=w252:refnum<vi>)
                    n117 = To More Generic Class(target class=w245, reference=w240) -> (generic class reference=w253:refnum<vi>)
                    n118 = To More Generic Class(target class=w245, reference=w239) -> (generic class reference=w254:refnum<vi>)
                    n119 = To More Generic Class(target class=w245, reference=w238) -> (generic class reference=w247:refnum<vi>)
                    n120 = To More Generic Class(target class=w245, reference=w237) -> (generic class reference=w246:refnum<vi>)
                    n121 = Build Array (concatenate)(w236, w250, w249, w251, w252, w253, w254, w247, w246) -> (w248:refnum<vi>[])
                  }
                  frame Default {
                  }
                }
              }
              n122 = Unbundle By Name(w181) -> ("CtrlStates"=w185:refnum<class "Class.SaveCtrls.lvclass">, "Cfg.Name"=w183:string, "Cfg.Dirs.App Data"=w184:path)
              n123 = call-dynamic "Class.SaveCtrls.InitLoadRestore.vi"("Ctrl Array"=w177, "Module Data Dir"=w184, "Module Name"=w183, "CtrlStates In"=w185) -> ("CtrlStates"=w182:refnum<class "Class.SaveCtrls.lvclass">)  [unwired: 6 in, 1 out]
              n124 = Bundle By Name(cluster=w181, "CtrlStates"=w182) -> (w180:T13)
            }
            frame 5 {
              n125 = Unbundle By Name(w258) -> ("CL Args.Active"=w257:bool)
              n126 = control-ref of="TE"() -> (w267:refnum<vi>)
              n127 = call "TestExec.Config, Get Station SW Module Info.vi"("Error if File Doesn't Exist"=TRUE) -> ("error out"=w266:errorcluster, "Station IP Port"=w265:i32)  [unwired: 7 in, 2 out]
              n128 = case shown="Error" w266 {
                tunnel: w261 -> [w283 w293]
                tunnel: [w282 w293] -> w260
                tunnel: w265 -> [w275 _]
                tunnel: w262 -> [w272 _]
                tunnel: [w271 _] -> w259
                tunnel: w267 -> [w270 _]
                tunnel: w257 -> [_ w284]
                frame No Error {
                  w276 = TRUE ("Listener")
                  n129 = To Unsigned Word Integer(number=w275) -> (unsigned 16bit integer=w274:u16)
                  n130 = call <vilib>:"Q.Obtain Queue.vi"("Q Name"="TE") -> ("Q Out"=w280:refnum<queue>)  [unwired: 8 in, 2 out]
                  n131 = property on="TE" class="Bool (strict)"("Visible"=TRUE) -> ()  [unwired: 2 in, 2 out]
                  n132 = Bundle By Name(cluster=T15 {"IP"="127.0.0.1", "Port"=8500, "Listener"=FALSE, "Enable"=FALSE} ("Config"), "Port"=w274, "Listener"=w276, "Enable"=w276) -> (w277:T15)
                  n133 = call <vilib>:"TCP-IP Q_Bridge.Create.vi"("Auto Exit"=TRUE, "Notification"=TRUE, "Config"=w277, "StatusCtrlRef"=w270, "Q_DataOut"=w280, "Q_DataIn"=w272, "Control Q Name"="TCP-IP_Bridge" ("Control Q")) -> ("Error Out"=w271:errorcluster)  [unwired: 3 in, 1 out]
                  n134 = Bundle By Name(cluster=w283, "Cfg.Parent Q"=w280) -> (w282:T13)
                }
                frame Error {
                  n135 = control-ref of="This VI"() -> (w289:refnum<vi>)
                  n136 = invoke class="VI" method="FP.Center"(reference=w289) -> (reference out=w290:refnum<vi>, error out=w291:errorcluster)  [unwired: 2 in, 1 out]
                  n137 = Select(t=T14."Minimized" ("State"), s=w284, f=T14."Standard" ("State")) -> (s? t:f=w287:T14)
                  n138 = property on="TE" class="Bool (strict)"("Visible"=FALSE) -> ()  [unwired: 2 in, 2 out]
                  n139 = invoke class="VI" method="FP.Open"(reference=w290, error in=w291, "Activate"=TRUE ("Activate?"), "State"=w287) -> ()  [unwired: 1 in, 5 out]
                }
              }
              "TE" <- FALSE ("Sta")
            }
            frame 6 {
              # "The Front Panel is hidden by default.\nShow front panel if it is run in the development environment."
              n140 = Unbundle By Name(w298) -> ("Exe"=w299:bool)
              n141 = case shown="False" w299 {
                frame False {
                  n142 = control-ref of="This VI"() -> (w302:refnum<vi>)
                  n143 = invoke class="VI" method="FP.Center"(reference=w302) -> (reference out=w303:refnum<vi>, error out=w304:errorcluster)  [unwired: 2 in, 1 out]
                  n144 = invoke class="VI" method="FP.Open"(reference=w303, error in=w304, "Activate"=TRUE ("Activate?"), "State"=T14."Standard") -> ()  [unwired: 1 in, 5 out]
                }
                frame True {
                }
              }
              n145 = Bundle By Name(cluster=w297, "Timeout(s)"="Timeout(s)", "SavWav"="Save Wav Files") -> (w296:T36)
            }
            frame 7 {
              # "Init the Function/Data manager"
              n146 = Unbundle By Name(w310) -> ("SW Rev.AppName"=w314:string, "SW Rev.Version"=w315:string)
              n147 = Unbundle By Name(w310) -> ("Cfg.Parent Q"=w317:refnum<queue>, "Main Q"=w318:refnum<queue>)
              n148 = Unbundle By Name(w307) -> ("FunctData"=w306:refnum<class "FunctDataMgr.lvclass">)
              n149 = Bundle By Name(cluster=T16 {"Name"="", "PN"="", "Version"="", "Note"=""} ("SW"), "Name"=w314, "Version"=w315) -> (w313:T16)
              n150 = call "FunctDataMgr.Reference Qs.vi"("Q Local"=w318, "Q Parent"=w317, "FunctDataMgr in"=w306) -> ("FunctDataMgr"=w319:refnum<class "FunctDataMgr.lvclass">)  [unwired: 7 in, 1 out]
              n151 = Build Array(w313) -> (w316:T16[])
              n152 = call "FunctDataMgr.Add Local SW Items.vi"("Local SW Items"=w316, "FunctDataMgr in"=w319) -> ("FunctDataMgr"=w305:refnum<class "FunctDataMgr.lvclass">)  [unwired: 8 in, 1 out]
              n153 = control-ref of="Show Only Failures"() -> (w322:refnum<vi>)
              n154 = control-ref of="Auto Scroll"() -> (w323:refnum<vi>)
              n155 = control-ref of="Results Table"() -> (w321:refnum<vi>)
              n156 = control-ref of="Filter"() -> (w320:refnum<vi>)
              n157 = call "FunctDataMgr.Reference RsltTbl Controls.vi"("ShowOnlyFail"=w322, "AutoScroll"=w323, "Filter"=w320, "Visible Rows"=13, "RsltTbl"=w321, "FunctDataMgr in"=w305) -> ("FunctDataMgr"=w309:refnum<class "FunctDataMgr.lvclass">)  [unwired: 4 in, 1 out]
              n158 = Bundle By Name(cluster=w307, "FunctData"=w309) -> (w308:T36)
            }
            frame 8 {
              w333 = T37 -5200 items=["No Error"=0, "Abort"=-2, "Misc"=-5000, "Fixture Error"=-5100, "File IO - General"=-5200, "FIle IO - Config Error"=-5201, "Instrument - General"=-5300, "Instrument - Serial Com"=-5301, "Instrument - Camera"=-5302, "Instrument - PS"=-5303, "Instrument - Oscilloscope"=-5304, "Instrument - Function Gen"=-5305, "Instrument - Load"=-5306, "Instrument - Meter"=-5307, "Instrument - Power Control"=-5308, "Instrument - Motion"=-5309, "Instrument - RF"=-5310, "System Exe"=-5400, "Image Processing"=-5500, "Communication"=-5600, "Script - Syntax Error"=-6000, "Script - Invalid Name or Param"=-6100, "Script - Timeout"=-6200, "Invalid Data"=-6300, "FW Update Error"=-6500] ("Std Code")
              # "Init Data Directories"
              n159 = Unbundle By Name(w346) -> ("Cfg.Dirs.Root"=w343:path)
              n160 = Build Path(base path=w343, name or relative path="Data") -> (appended path=w331:path)
              n161 = Build Path(base path=w331, name or relative path="ArchiveSummary") -> (appended path=w328:path)
              n162 = Build Path(base path=w331, name or relative path="Archive") -> (appended path=w341:path)
              n163 = Build Path(base path=w331, name or relative path="Temp") -> (appended path=w330:path)
              n164 = call <vilib>:"File.Create Folder if Does Not Exist.vi"("Path"=w341) -> ("error out"=w337:errorcluster, "Dup Path"=w327:path)  [unwired: 8 in, 1 out]
              n165 = call <vilib>:"File.Create Folder if Does Not Exist.vi"("Path"=w328) -> ("error out"=w336:errorcluster, "Dup Path"=w326:path)  [unwired: 8 in, 1 out]
              n166 = call <vilib>:"File.Create Folder if Does Not Exist.vi"("Path"=w330) -> ("error out"=w338:errorcluster, "Dup Path"=w324:path)  [unwired: 8 in, 1 out]
              n167 = Merge Errors(w338, w337, w336) -> (w335:errorcluster)
              n168 = case shown="True" FALSE {
                tunnel: w324 -> [_ w347]
                frame False {
                }
                frame True {
                  n169 = call <vilib>:"File.Delete Files and SubFolders in a Dir.vi"("Dir"=w347) -> ()  [unwired: 9 in, 2 out]
                }
              }
              n170 = Bundle By Name(cluster=w345, "Dirs.Temp Data"=w324, "Dirs.Archive"=w327, "Dirs.ArchiveSum"=w326) -> (w344:T36)
              n171 = call "Error.Set-Change Error Info.vi"("Std Code"=w333, "error in"=w335, "Description"="Error creating local data folders.") -> ("error out"=w334:errorcluster)  [unwired: 8 in]
            }
            frame 9 {
              n172 = local read "Logging Level"() -> (w352:T8)
              n173 = To Variant(anything=w352) -> (Variant=w354:variant)
              n174 = call <vilib>:"Q.Enqueue App.vi"("Data1"=w354, "Task Name"="Set Logging Level", "Q In"=w353) -> ()  [unwired: 7 in, 2 out]
              n175 = local read "R Level Color"() -> (w350:u32)
              n176 = local read "R Delta Color"() -> (w351:u32)
              n177 = local read "L Delta Color"() -> (w349:u32)
              n178 = local read "L Level Color"() -> (w348:u32)
              n179 = property on="L AvgMagUnCov" class="DigNum (strict)"("NumText.BGColor"=w348) -> ()  [unwired: 2 in, 2 out]
              n180 = property on="R AvgMagUnCov" class="DigNum (strict)"("NumText.BGColor"=w350) -> ()  [unwired: 2 in, 2 out]
              n181 = property on="R AvgMag Delta" class="DigNum (strict)"("NumText.BGColor"=w351) -> ()  [unwired: 2 in, 2 out]
              n182 = property on="L AvgMag Delta" class="DigNum (strict)"("NumText.BGColor"=w349) -> ()  [unwired: 2 in, 2 out]
            }
            frame 10 {
              n183 = local read "Sound Devices"() -> (w364:T6)
              n184 = Unbundle By Name(w364) -> ("AudioInName"=w363:string, "AudioOutName"=w362:string)
              n185 = call "AudioTest.Get PC Audio Device List.vi"() -> ("Output Devices"=w367:string[], "Input Devices"=w366:string[])  [unwired: 10 in]
              n186 = call "Array.Search for Item Based on Pattern.vi"("Pattern"=w363, "List"=w366) -> ("Index"=w368:i32, "Found"=w360:bool)  [unwired: 7 in, 1 out]
              n187 = call "Array.Search for Item Based on Pattern.vi"("Pattern"=w362, "List"=w367) -> ("Index"=w371:i32, "Found Item"=w370:string, "Found"=w359:bool)  [unwired: 7 in]
              n188 = And(x=w360, y=w359) -> (x .and. y?=w361:bool)
              n189 = property on="Input Device" class="Ring (strict)"("Strings []"=w366) -> ()  [unwired: 2 in, 2 out]
              n190 = property on="Output Device" class="Ring (strict)"("Strings []"=w367) -> ()  [unwired: 2 in, 2 out]
              n191 = case shown="False" w361 {
                tunnel: w359 -> [w378 _]
                tunnel: [w374 _] -> w358
                frame False {
                  w375 = T37 -5300 items=["No Error"=0, "Abort"=-2, "Misc"=-5000, "Fixture Error"=-5100, "File IO - General"=-5200, "FIle IO - Config Error"=-5201, "Instrument - General"=-5300, "Instrument - Serial Com"=-5301, "Instrument - Camera"=-5302, "Instrument - PS"=-5303, "Instrument - Oscilloscope"=-5304, "Instrument - Function Gen"=-5305, "Instrument - Load"=-5306, "Instrument - Meter"=-5307, "Instrument - Power Control"=-5308, "Instrument - Motion"=-5309, "Instrument - RF"=-5310, "System Exe"=-5400, "Image Processing"=-5500, "Communication"=-5600, "Script - Syntax Error"=-6000, "Script - Invalid Name or Param"=-6100, "Script - Timeout"=-6200, "Invalid Data"=-6300, "FW Update Error"=-6500] ("Std Code")
                  n192 = Select(t="Configured Audio Input device not found", s=w378, f="Configured Audio Output device not found") -> (s? t:f=w376:string)
                  n193 = call "Error.Set Error.vi"("Code"=w375, "Desc"=w376) -> ("error out"=w374:errorcluster)  [unwired: 5 in]
                }
                frame True {
                }
              }
              n194 = case shown="Default" w368 {
                selector: w368 -> [w382 _]
                tunnel: [w382 0 ("lower limit")] -> w365
                frame Default {
                }
                frame -1 {
                }
              }
              n195 = case shown="Default" w371 {
                selector: w371 -> [w380 _]
                tunnel: [w380 0] -> w369
                tunnel: w370 -> [_ _]
                frame Default {
                }
                frame -1 {
                }
              }
              n196 = local write "Output Device"(w369) -> ()
              n197 = local write "Input Device"(w365) -> ()
            }
            frame Default {
              # "Done"
            }
          }
        }
        n198 = Merge Errors(w32) -> (w31:errorcluster)
      }
      frame "Reset" {
        n199 = while {
          shift-right: [w396] -> w389
          shift-left: w391 -> [w397]
          shift-right: [w394] -> w388
          shift-left: w390 -> [w395]
          tunnel: w387 -> [w392]
          i -> [w398]
          stop <- w393 stop-if-true
          n200 = case shown="Default" w398 {
            tunnel: w397 -> [w403 w407 w426]
            tunnel: [w403 w407 w426] -> w396
            tunnel: w395 -> [w400 w404 w418]
            tunnel: [w401 w404 w419] -> w394
            tunnel: [TRUE _ _] -> w393
            tunnel: w392 -> [_ _ w431]
            frame Default {
              # "Done"
              n201 = Bundle By Name(cluster=w400, "Rslt.Meas"=T17[] []) -> (w401:T36)
            }
            frame 0 {
              # "Init Controls"
              n202 = invoke on="SN" class="Str" method="Reinit To Default"() -> ()  [unwired: 3 in, 3 out]
              n203 = property on="Status" class="Str"("Text.BGColor"=u32 13816530) -> ()  [unwired: 2 in, 2 out]
              n204 = Unbundle By Name(w407) -> ("Log"=w415:refnum<class "Event Notification.lvclass">)
              n205 = local write "Status"("Initializing" ("Status")) -> ()
              n206 = local write "Main Tab"(0) -> ()
              n207 = local write "Control Tab"(0) -> ()
              n208 = local write "Result Data Tab"(0) -> ()
              n209 = call <vilib>:"Event Notification.Status Message.vi"("Log"=TRUE, "Level"=Event_Log.Log_Level."Verbose", "Message"="Reset - Initializing", "Event Notification in"=w415) -> ()  [unwired: 8 in]
              n210 = invoke on="Play Tone" class="Bool (strict)" method="Reinit To Default"() -> ()  [unwired: 3 in, 3 out]
              n211 = Unbundle By Name(w407) -> ("Cfg.Dirs.Config"=w406:path)
              n212 = Build Path(base path=w406, name or relative path="Audio Sequences") -> ()  [unwired: 1 out]
            }
            frame 1 {
              w420 = FALSE ("Lnch")
              # "Enqueue Tasks"
              n213 = Unbundle By Name(w418) -> ("Lnch"=w417:bool)
              n214 = Flush Queue(queue=w431) -> (queue out=w433:refnum<queue>)  [unwired: 1 in, 2 out]
              n215 = case shown="True" w417 {
                tunnel: [string[] ["Test End", "Test Reset", "Config - Read"] string[] ["Config - Read"]] -> w430
                frame False {
                }
                frame True {
                }
              }
              n216 = call <vilib>:"Scheduler.Clear-Reset.vi"("Q In"=w433) -> ("Q Out"=w432:refnum<queue>)  [unwired: 9 in, 1 out]
              n217 = call "Error.Clear.vi"("Q In"=w432) -> ("Q Out"=w425:refnum<queue>)  [unwired: 9 in, 1 out]
              n218 = property on="Abort" class="Bool"("DisabledEnum"=T19."Disabled and Grayed Out" ("Disabled")) -> ()  [unwired: 2 in, 2 out]
              n219 = Unbundle By Name(w418) -> ("CL Args.Active"=w423:bool)
              n220 = for {
                shift-right: [w441] -> w427
                shift-left: _ -> [w442]
                tunnel: w430 -> [w439] mode=indexing
                shift-right: [w440] -> w428
                shift-left: w425 -> [w443]
                n221 = call <vilib>:"Q.Enqueue Task.vi"("Error In"=w442, "Task Name"=w439, "Q In"=w443) -> ("error out"=w441:errorcluster, "Q Out"=w440:refnum<queue>)  [unwired: 7 in]
              }
              n222 = Unbundle By Name(w418) -> ("FunctData"=w421:refnum<class "FunctDataMgr.lvclass">)
              n223 = call "FunctDataMgr.Reset Data.vi"("FunctDataMgr in"=w421) -> ("FunctDataMgr out"=w422:refnum<class "FunctDataMgr.lvclass">)  [unwired: 9 in, 1 out]
              n224 = call <vilib>:"Q.Enqueue App.vi"("Error In"=w427, "Task Name"="Initialization Done", "Q In"=w428) -> ("Q Out"=w424:refnum<queue>)  [unwired: 7 in, 1 out]
              n225 = case shown="True" w423 {
                tunnel: w424 -> [_ w438]
                frame False {
                }
                frame True {
                  n226 = call <vilib>:"Q.Enqueue Task.vi"("Task Name"="CL_Arg_Seq", "Q In"=w438) -> ()  [unwired: 8 in, 2 out]
                }
              }
              n227 = Bundle By Name(cluster=w418, "FunctData"=w422, "Lnch"=w420, "Remote Test"=w420) -> (w419:T36)
            }
          }
        }
      }
      frame "Task" {
        n228 = case shown="\"MicrophoneTest\"" w449 {
          selector: w449 -> [_ _ _ _ _ _ _ _ _ w1284 _ _ _ _ _ _ _ _ _ _ _ _ _ _ _ _ _ _ _ _ _ _ w1684]
          tunnel: w453 -> [w468 w483 w488 w501 w621 w1231 w1248 w1264 w1267 w1297 w1328 w1364 w1368 w1372 w1395 w1397 w1399 w1421 w1437 w1456 w1475 w1484 w1497 w1570 w1578 w1581 w1587 w1596 w1597 w1642 w1644 w1669 w1692]
          tunnel: w452 -> [w459 w484 w494 w500 w626 w1233 w1244 w1263 w1266 w1298 w1326 w1343 w1366 w1379 w1391 w1396 w1398 w1422 w1431 w1453 w1472 w1477 w1496 w1564 w1573 w1584 w1586 w1589 w1605 w1641 w1654 w1668 w1687]
          tunnel: [w468 w483 w488 w501 w621 w1231 w1248 w1264 w1267 w1297 w1328 w1364 w1368 w1372 w1395 w1397 w1404 w1421 w1437 w1456 w1475 w1484 w1493 w1570 w1578 w1580 w1587 w1596 w1597 w1642 w1644 w1669 w1691] -> w451
          tunnel: [w458 w482 w494 w495 w625 w1234 w1245 w1263 w1266 w1298 w1327 w1343 w1367 w1378 w1390 w1396 w1398 w1422 w1430 w1455 w1471 w1485 w1492 w1566 w1575 w1584 w1586 w1594 w1598 w1640 w1654 w1668 w1686] -> w450
          tunnel: w448 -> [w471 w478 _ _ w624 _ _ _ _ _ _ _ _ _ w1394 _ w1409 _ w1435 _ w1474 _ w1494 w1568 w1577 w1583 _ w1595 w1606 _ w1645 _ w1689]
          tunnel: w447 -> [w472 _ _ w498 _ w1232 w1243 _ _ w1272 w1301 _ _ _ _ _ w1407 w1424 _ w1464 _ w1488 w1495 _ _ _ _ _ _ _ _ _ _]
          tunnel: w446 -> [_ _ _ w497 _ _ _ _ _ _ _ _ _ _ _ _ _ _ _ _ _ _ _ _ _ _ _ _ _ _ _ _ w1694]
          tunnel: w445 -> [_ w477 _ _ _ _ _ _ _ _ _ _ _ _ _ _ _ _ _ _ _ _ _ _ _ _ _ _ _ _ _ _ w1695]
          tunnel: [_ w479 _ w496 w620 _ _ _ _ w1285 w1315 _ _ w1373 w1393 _ _ _ _ _ _ _ w1491 _ _ _ _ _ w1600 _ _ w1660 w1693] -> w444
          frame "Funct Local Call" {
            n229 = Variant To Data(type=string[] [], Variant=w471) -> (data=w462:string[])  [unwired: 1 in, 1 out]
            n230 = Delete From Array(array=w462, index=0) -> (deleted portion=w456:string, array with subset deleted=w460:string[])  [unwired: 1 in]
            n231 = Unbundle By Name(w468) -> ("Log"=w467:refnum<class "Event Notification.lvclass">)
            n232 = Concatenate Strings("Running: ", w456) -> (w466:string)
            n233 = call <vilib>:"Q.Enqueue Task.vi"("Task Name"="Test Start", "Q In"=w472) -> ("Q Out"=w475:refnum<queue>)  [unwired: 8 in, 1 out]
            n234 = call <vilib>:"Event Notification.Status Message.vi"("Level"=Event_Log.Log_Level."Verbose", "Message"=w466, "Event Notification in"=w467) -> ()  [unwired: 9 in]
            n235 = To Variant(anything=w460) -> (Variant=w455:variant)
            n236 = Get Date/Time In Seconds() -> (seconds since 1Jan1904=→"Start Time":timestamp)
            n237 = local write "Duration(s)"(0.0 ("Duration(s)")) -> ()
            n238 = call <vilib>:"Q.Enqueue Item.vi"("Data1"=w455, "Sub"=w456, "Cmd"="Function", "Q In"=w475) -> ("Q Out"=w474:refnum<queue>)  [unwired: 6 in, 1 out]
            n239 = call <vilib>:"Q.Enqueue Task.vi"("Task Name"="Test End", "Q In"=w474) -> ()  [unwired: 8 in, 2 out]
            n240 = Bundle By Name(cluster=w459, "Remote Test"=FALSE ("Local Test")) -> (w458:T36)
          }
          frame "Funct RTN" {
            n241 = Unbundle By Name(w484) -> ("FunctData"=w481:refnum<class "FunctDataMgr.lvclass">)
            n242 = call "FunctDataMgr.Function Return.vi"("RTN Info"=w477, "RTN Vars"=w478, "FunctDataMgr in"=w481) -> ("Error Out"=w479:errorcluster, "FunctDataMgr out"=w480:refnum<class "FunctDataMgr.lvclass">)  [unwired: 7 in]
            n243 = Bundle By Name(cluster=w484, "FunctData"=w480) -> (w482:T36)
          }
          frame "HMD Module Undock" {
            n244 = Unbundle By Name(w488) -> ("Child Modules"=w486:cluster{"Name":string, "vi ref":refnum<vi>}[])
            n245 = control-ref of="HMD"() -> (w489:refnum<vi>)
            n246 = Index Array(array=w486) -> (element=w487:cluster{"Name":string, "vi ref":refnum<vi>})  [unwired: 1 in]
            n247 = Unbundle By Name(w487) -> ("Name"=w485:string)
            n248 = call <vilib>:"Module.Window, Q Task.vi"("Sub Panel"=w489, "Q Name"=w485, "Action"=Window.Task,_Action."Dock to SubPanel(SubPanel Ref)") -> ("error out"=w491:errorcluster)  [unwired: 7 in, 1 out]
            n249 = call <vilib>:"Clear Errors.vi"("error in (no error)"=w491) -> ("error out"=w490:errorcluster)  [unwired: 5 in, 1 out]
            n250 = call <vilib>:"Module.Window, Q Task.vi"("Q Name"=w485, "error in"=w490, "Action"=Window.Task,_Action."Undock from SubPanel()") -> ()  [unwired: 7 in, 2 out]
          }
          frame "CL_Arg_Seq" {
            n251 = while {
              shift-right: [w510] -> w495
              shift-left: w500 -> [w512]
              shift-right: [w509] -> _
              shift-left: "Init" -> [w511]
              tunnel: w498 -> [w506]
              shift-right: [w505] -> w496
              shift-left: w497 -> [w504]
              shift-right: [w502] -> _
              shift-left: _ -> [w503]
              stop <- w507 stop-if-true
              n252 = case shown="\"Init\"" w511 {
                tunnel: w512 -> [w516 w528 w556 w575 w595 w605]
                tunnel: [w516 w528 w556 w575 w595 w605] -> w510
                tunnel: ["Command" w524 "Sweep Param2 Check" "Data Dir Check" "Done" "Done"] -> w508
                tunnel: [_ _ _ _ _ TRUE] -> w507
                tunnel: w506 -> [_ _ _ _ _ w608]
                tunnel: [w513 w527 w554 w573 w593 w607] -> w505
                tunnel: w504 -> [_ _ _ _ _ w607]
                tunnel: w503 -> [w515 _ w551 w570 w592 w604]
                tunnel: [w515 w521 w551 w570 w592 w604] -> w502
                frame "Init" {
                  # "RTN if error exists."
                  n253 = invoke on="Play Tone" class="Bool (strict)" method="Reinit To Default"() -> ()  [unwired: 3 in, 3 out]
                  n254 = local read "Error"() -> (w513:errorcluster)
                }
                frame "Command" {
                  w523 = ""  # DataDir
                  # "== Args: ==\nTest\nType\nSide\nDataDir"
                  n255 = Unbundle By Name(w528) -> ("CL Args.Test"=w518:string, "CL Args.Args"=w520:string[])
                  n256 = call <vilib>:"Trim Whitespace.vi"("string"=w518) -> ("trimmed string"=w517:string)  [unwired: 1 in]
                  n257 = Index Array(array=w520, index=0) -> (element=w525:string)
                  n258 = case shown="\"MicrophoneTest\"" w517 {
                    selector: w517 -> [w529 _]
                    tunnel: [w530 w536] -> w527
                    tunnel: w525 -> [_ w538]
                    tunnel: [_ w537] -> w524
                    tunnel: w520 -> [_ w535]
                    tunnel: [_ w534] -> w519
                    frame Default {
                      w533 = T37 -6100 items=["No Error"=0, "Abort"=-2, "Misc"=-5000, "Fixture Error"=-5100, "File IO - General"=-5200, "FIle IO - Config Error"=-5201, "Instrument - General"=-5300, "Instrument - Serial Com"=-5301, "Instrument - Camera"=-5302, "Instrument - PS"=-5303, "Instrument - Oscilloscope"=-5304, "Instrument - Function Gen"=-5305, "Instrument - Load"=-5306, "Instrument - Meter"=-5307, "Instrument - Power Control"=-5308, "Instrument - Motion"=-5309, "Instrument - RF"=-5310, "System Exe"=-5400, "Image Processing"=-5500, "Communication"=-5600, "Script - Syntax Error"=-6000, "Script - Invalid Name or Param"=-6100, "Script - Timeout"=-6200, "Invalid Data"=-6300, "FW Update Error"=-6500] ("Std Code")
                      n259 = Format Into String(format string="Invalid Command \"%s\".  Expected \"MicrophoneTest\"", w529) -> (resulting string=w532:string)  [unwired: 2 in, 1 out]
                      n260 = call "Error.Set Error.vi"("Code"=w533, "Desc"=w532) -> ("error out"=w530:errorcluster)  [unwired: 5 in]
                    }
                    frame "MicrophoneTest" {
                      # "OK"
                      n261 = case shown="\"Sweep\"" w538 {
                        selector: w538 -> [w539 _]
                        tunnel: ["Done" "Sweep Param1 Check"] -> w537
                        tunnel: [w541 _] -> w536
                        tunnel: w535 -> [_ w547]
                        tunnel: [_ w545] -> w534
                        frame Default {
                          w544 = T37 -6100 items=["No Error"=0, "Abort"=-2, "Misc"=-5000, "Fixture Error"=-5100, "File IO - General"=-5200, "FIle IO - Config Error"=-5201, "Instrument - General"=-5300, "Instrument - Serial Com"=-5301, "Instrument - Camera"=-5302, "Instrument - PS"=-5303, "Instrument - Oscilloscope"=-5304, "Instrument - Function Gen"=-5305, "Instrument - Load"=-5306, "Instrument - Meter"=-5307, "Instrument - Power Control"=-5308, "Instrument - Motion"=-5309, "Instrument - RF"=-5310, "System Exe"=-5400, "Image Processing"=-5500, "Communication"=-5600, "Script - Syntax Error"=-6000, "Script - Invalid Name or Param"=-6100, "Script - Timeout"=-6200, "Invalid Data"=-6300, "FW Update Error"=-6500] ("Std Code")
                          n262 = Format Into String(format string="Invalid Action \"%s\", Expected \"Sweep\" or \"Analysis\".", w539) -> (resulting string=w543:string)  [unwired: 2 in, 1 out]
                          n263 = call "Error.Set Error.vi"("Code"=w544, "Desc"=w543) -> ("error out"=w541:errorcluster)  [unwired: 5 in]
                        }
                        frame "Sweep" {
                          n264 = Index Array(array=w547, index=3) -> (element=w545:string)
                        }
                      }
                    }
                  }
                  n265 = Bundle("DataDir"=w523) -> (w522:cluster{"DataDir":string})  [unwired: 1 in]
                  n266 = Bundle By Name(cluster=w522, "DataDir"=w519) -> (w521:cluster{"DataDir":string})
                }
                frame "Sweep Param1 Check" {
                  n267 = Unbundle By Name(w556) -> ("CL Args.Args"=w553:string[])
                  n268 = Index Array(array=w553, index=1) -> (element=w550:string)
                  n269 = call <vilib>:"Trim Whitespace.vi"("string"=w550) -> ("trimmed string"=w549:string)  [unwired: 1 in]
                  n270 = case shown="\"Right\"" w549 {
                    selector: w549 -> [w557 _ _]
                    tunnel: [w558 _ _] -> w554
                    frame Default {
                      w561 = T37 -6100 items=["No Error"=0, "Abort"=-2, "Misc"=-5000, "Fixture Error"=-5100, "File IO - General"=-5200, "FIle IO - Config Error"=-5201, "Instrument - General"=-5300, "Instrument - Serial Com"=-5301, "Instrument - Camera"=-5302, "Instrument - PS"=-5303, "Instrument - Oscilloscope"=-5304, "Instrument - Function Gen"=-5305, "Instrument - Load"=-5306, "Instrument - Meter"=-5307, "Instrument - Power Control"=-5308, "Instrument - Motion"=-5309, "Instrument - RF"=-5310, "System Exe"=-5400, "Image Processing"=-5500, "Communication"=-5600, "Script - Syntax Error"=-6000, "Script - Invalid Name or Param"=-6100, "Script - Timeout"=-6200, "Invalid Data"=-6300, "FW Update Error"=-6500] ("Std Code")
                      n271 = Format Into String(format string="Invalid Param1 \"%s\".  Expected \"Left\" or \"Right\".", w557) -> (resulting string=w560:string)  [unwired: 2 in, 1 out]
                      n272 = call "Error.Set Error.vi"("Code"=w561, "Desc"=w560) -> ("error out"=w558:errorcluster)  [unwired: 5 in]
                    }
                    frame "Right" {
                      n273 = local read "Mic Test Setup"() -> (w563:T3)
                      n274 = Bundle By Name(cluster=w563, "Mic Side"=enum32{"LEFT", "RIGHT"}."RIGHT") -> (w564:T3)
                      n275 = local write "Mic Test Setup"(w564) -> ()
                    }
                    frame "Left" {
                      n276 = local read "Mic Test Setup"() -> (w566:T3)
                      n277 = Bundle By Name(cluster=w566, "Mic Side"=enum32{"LEFT", "RIGHT"}."LEFT") -> (w567:T3)
                      n278 = local write "Mic Test Setup"(w567) -> ()
                    }
                  }
                }
                frame "Sweep Param2 Check" {
                  n279 = Unbundle By Name(w575) -> ("CL Args.Args"=w572:string[])
                  n280 = Index Array(array=w572, index=2) -> (element=w569:string)
                  n281 = call <vilib>:"Trim Whitespace.vi"("string"=w569) -> ("trimmed string"=w568:string)  [unwired: 1 in]
                  n282 = case shown="Default" w568 {
                    selector: w568 -> [w576 _ _]
                    tunnel: [w577 _ _] -> w573
                    frame Default {
                      w580 = T37 -6100 items=["No Error"=0, "Abort"=-2, "Misc"=-5000, "Fixture Error"=-5100, "File IO - General"=-5200, "FIle IO - Config Error"=-5201, "Instrument - General"=-5300, "Instrument - Serial Com"=-5301, "Instrument - Camera"=-5302, "Instrument - PS"=-5303, "Instrument - Oscilloscope"=-5304, "Instrument - Function Gen"=-5305, "Instrument - Load"=-5306, "Instrument - Meter"=-5307, "Instrument - Power Control"=-5308, "Instrument - Motion"=-5309, "Instrument - RF"=-5310, "System Exe"=-5400, "Image Processing"=-5500, "Communication"=-5600, "Script - Syntax Error"=-6000, "Script - Invalid Name or Param"=-6100, "Script - Timeout"=-6200, "Invalid Data"=-6300, "FW Update Error"=-6500] ("Std Code")
                      n283 = Format Into String(format string="Invalid Param2 \"%s\".  Expected \"Covered\" or \"Uncovered\".", w576) -> (resulting string=w579:string)  [unwired: 2 in, 1 out]
                      n284 = call "Error.Set Error.vi"("Code"=w580, "Desc"=w579) -> ("error out"=w577:errorcluster)  [unwired: 5 in]
                    }
                    frame "Covered" {
                      n285 = local read "Mic Test Setup"() -> (w582:T3)
                      n286 = Bundle By Name(cluster=w582, "Covered"=TRUE) -> (w583:T3)
                      n287 = local write "Mic Test Setup"(w583) -> ()
                    }
                    frame "Uncovered" {
                      n288 = local read "Mic Test Setup"() -> (w585:T3)
                      n289 = Bundle By Name(cluster=w585, "Covered"=FALSE) -> (w586:T3)
                      n290 = local write "Mic Test Setup"(w586) -> ()
                    }
                  }
                }
                frame "Data Dir Check" {
                  n291 = Unbundle By Name(w592) -> ("DataDir"=w589:string)
                  n292 = call <vilib>:"Trim Whitespace.vi"("string"=w589) -> ("trimmed string"=w588:string)  [unwired: 1 in]
                  n293 = case shown="\"\"" w588 {
                    selector: w588 -> [w597 _]
                    tunnel: [w596 w598] -> w587
                    frame Default {
                      n294 = String To Path(string=w597) -> (path=w596:path)
                    }
                    frame "" {
                      n295 = local read "Default Data Folder"() -> (w598:path)
                    }
                  }
                  n296 = call <vilib>:"File.Create Folder if Does Not Exist.vi"("Path"=w587) -> ("error out"=w591:errorcluster, "Dup Path"=w590:path)  [unwired: 8 in, 1 out]
                  n297 = local write "UUT Dir"(w587) -> ()
                  n298 = case shown="Error" w591 {
                    tunnel: w590 -> [_ w602]
                    tunnel: [_ w599] -> w593
                    frame No Error {
                    }
                    frame Error {
                      w603 = T37 -6100 items=["No Error"=0, "Abort"=-2, "Misc"=-5000, "Fixture Error"=-5100, "File IO - General"=-5200, "FIle IO - Config Error"=-5201, "Instrument - General"=-5300, "Instrument - Serial Com"=-5301, "Instrument - Camera"=-5302, "Instrument - PS"=-5303, "Instrument - Oscilloscope"=-5304, "Instrument - Function Gen"=-5305, "Instrument - Load"=-5306, "Instrument - Meter"=-5307, "Instrument - Power Control"=-5308, "Instrument - Motion"=-5309, "Instrument - RF"=-5310, "System Exe"=-5400, "Image Processing"=-5500, "Communication"=-5600, "Script - Syntax Error"=-6000, "Script - Invalid Name or Param"=-6100, "Script - Timeout"=-6200, "Invalid Data"=-6300, "FW Update Error"=-6500] ("Std Code")
                      n299 = Format Into String(format string="Unable to access or create UUT Folder \"%s\"", w602) -> (resulting string=w601:string)  [unwired: 2 in, 1 out]
                      n300 = call "Error.Set Error.vi"("Code"=w603, "Desc"=w601) -> ("error out"=w599:errorcluster)  [unwired: 5 in]
                    }
                  }
                }
                frame "Done", Default {
                  n301 = case shown="No Error" w607 {
                    tunnel: w608 -> [w617 w618]
                    tunnel: w605 -> [w615 _]
                    tunnel: [w613 w618] -> w606
                    frame No Error {
                      n302 = Unbundle By Name(w615) -> ("CL Args.Test"=w614:string, "CL Args.Args"=w612:string[])
                      n303 = To Variant(anything=w612) -> (Variant=w616:variant)
                      n304 = call <vilib>:"Q.Enqueue Task.vi"("Data1"=w616, "Task Name"=w614, "Q In"=w617) -> ("Q Out"=w613:refnum<queue>)  [unwired: 7 in, 1 out]
                    }
                    frame Error {
                    }
                  }
                  n305 = call <vilib>:"Q.Enqueue Task.vi"("Task Name"="CL_Test_RTN", "Q In"=w606) -> ()  [unwired: 8 in, 2 out]
                }
              }
              n306 = call "Error.Case Redirect on Error.vi"("error in"=w505, "Next Case"=w508) -> ("Next Case Out"=w509:string)  [unwired: 9 in]
            }
          }
          frame "MicrophoneTest" {
            n307 = Variant To Data(type=string[] [], Variant=w624) -> (data=w622:string[], error out=w623:errorcluster)  [unwired: 1 in]
            n308 = while {
              shift-right: [w639] -> w625
              shift-left: w626 -> [w640]
              shift-right: [w628] -> _
              shift-left: "Init" -> [w629]
              shift-right: [w635] -> w620
              shift-left: w623 -> [w636]
              tunnel: w622 -> [w634]
              tunnel: w621 -> [w633]
              shift-right: [w631] -> _
              shift-left: _ -> [w632]
              shift-right: [w629] -> _
              shift-left: _ -> [w630]
              stop <- w638 stop-if-true
              n309 = case shown="\"Play Sweep\"" w629 {
                tunnel: w640 -> [w642 w678 w698 w731 w761 w791 w846 w1178 w1198]
                tunnel: [w643 w678 w698 w731 w761 w791 w849 w1178 w1198] -> w639
                tunnel: [_ _ _ _ _ _ _ _ TRUE] -> w638
                tunnel: ["Set Mic State" "Build Sweep" "Cal Sweep" "Play Sweep" "Calculate Data" "Process Data" "Results" "Done" "Done"] -> w637
                tunnel: w636 -> [_ _ _ _ _ _ _ _ w1189]
                tunnel: [_ w670 w699 _ w755 w792 _ w1175 w1189] -> w635
                tunnel: w634 -> [w655 _ _ _ _ _ _ _ _]
                tunnel: w633 -> [w667 w672 w713 w735 _ _ _ _ w1191]
                tunnel: w632 -> [_ w677 w715 w734 w758 w802 w845 w1173 w1195]
                tunnel: [w648 w677 w714 w734 w759 w803 w847 w1173 w1195] -> w631
                tunnel: w630 -> [_ _ _ _ _ _ _ _ w1190]
                frame "Init" {
                  w646 = TRUE
                  w650 = 0.0  # Start
                  w656 = cluster{"F":dbl[], "M":dbl[]} {"F"=[], "M"=[]}  # THD
                  w657 = ""  # TestName
                  w658 = cluster{"F":dbl[], "M":dbl[]} {"F"=[], "M"=[]}  # Mag
                  w659 = 0.0  # AvgMag
                  w660 = refnum<class "SV Discrete Sweep.lvclass"> refnum  # SigConfig
                  w661 = 0  # SmplCnt
                  w664 = waveform(dbl) {"t0"=timestamp(0 s since 1904-01-01), "dt"=1.0, "Y"=[]}  # Mic
                  w665 = waveform(dbl) {"t0"=timestamp(0 s since 1904-01-01), "dt"=1.0, "Y"=[]}  # SweepCal
                  w666 = waveform(dbl) {"t0"=timestamp(0 s since 1904-01-01), "dt"=1.0, "Y"=[]}  # Sweep
                  n310 = Array To Spreadsheet String(delimiter (Tab)=", ", array=w655, 3:"" ("format string")) -> (spreadsheet string=w652:string)
                  n311 = Unbundle By Name(w667) -> ("Log"=w669:refnum<class "Event Notification.lvclass">)
                  n312 = call <vilib>:"Trim Whitespace.vi"("string"=w652) -> ("trimmed string"=w651:string)  [unwired: 1 in]
                  n313 = Format Into String(format string="Test: %s" ("Message"), w651) -> (resulting string=w644:string)  [unwired: 2 in, 1 out]
                  n314 = call <vilib>:"Event Notification.Status Message.vi"("Display"=TRUE ("Log"), "Level"=Event_Log.Log_Level."Normal", "Message"=w644, "Event Notification in"=w669) -> ()  [unwired: 8 in]
                  n315 = property on="Test Running" class="Bool (strict)"("Blinking"=w646, "Value"=w646) -> ()  [unwired: 2 in, 2 out]
                  n316 = Bundle By Name(cluster=w642, "Rslt.Meas"=T17[] []) -> (w643:T36)
                  n317 = Bundle("Sweep"=w666, "SweepCal"=w665, "Mic"=w664, "SmplCnt"=w661, "SigConfig"=w660, "AvgMag"=w659, "Mag"=w658, "THD"=w656, "TestName"=w657, "Start"=w650) -> (w649:T38)  [unwired: 1 in]
                  n318 = call <vilib>:"High Resolution Relative Seconds.vi"() -> ("relative seconds"=w647:dbl)
                  n319 = Bundle By Name(cluster=w649, "Start"=w647) -> (w648:T38)
                }
                frame "Set Mic State" {
                  n320 = Unbundle By Name("Mic Test Setup") -> ("Mic Side"=w676:enum32{"LEFT", "RIGHT"})
                  n321 = Unbundle By Name(w672) -> ("Cfg.Simulate"=w671:bool)
                  n322 = case shown="\"RIGHT\"" w676 {
                    tunnel: ["1" "2"] -> w675
                    frame "LEFT", Default {
                    }
                    frame "RIGHT" {
                    }
                  }
                  n323 = case shown="False" w671 {
                    tunnel: w675 -> [w680 _]
                    tunnel: [w682 _] -> w670
                    frame False {
                      w683 = T37 -5600 items=["No Error"=0, "Abort"=-2, "Misc"=-5000, "Fixture Error"=-5100, "File IO - General"=-5200, "FIle IO - Config Error"=-5201, "Instrument - General"=-5300, "Instrument - Serial Com"=-5301, "Instrument - Camera"=-5302, "Instrument - PS"=-5303, "Instrument - Oscilloscope"=-5304, "Instrument - Function Gen"=-5305, "Instrument - Load"=-5306, "Instrument - Meter"=-5307, "Instrument - Power Control"=-5308, "Instrument - Motion"=-5309, "Instrument - RF"=-5310, "System Exe"=-5400, "Image Processing"=-5500, "Communication"=-5600, "Script - Syntax Error"=-6000, "Script - Invalid Name or Param"=-6100, "Script - Timeout"=-6200, "Invalid Data"=-6300, "FW Update Error"=-6500] ("Std Code")
                      n324 = Build Array(w680) -> (w679:string[])
                      n325 = To Variant(anything=w679) -> (Variant=w687:variant)
                      n326 = call <vilib>:"Q.Send Function Command and wait on Ret Data.vi"("Timeout(ms)"=20000, "Q Name"="HMD", "Data1"=w687, "Cmd"="SetMicState" ("Q Name")) -> ("error out"=w685:errorcluster)  [unwired: 6 in, 1 out]
                      n327 = call "Error.Set-Change Error Info.vi"("Std Code"=w683, "Append Details"=FALSE, "error in"=w685, "Description"="Error communicating with DUT.  Was not able to set the Mic State." ("Q Name")) -> ("error out"=w682:errorcluster)  [unwired: 7 in]
                    }
                    frame True {
                    }
                  }
                }
                frame "Build Sweep" {
                  n328 = local read "Sine Sweep Params"() -> (w703:T7)
                  n329 = Unbundle By Name(w713) -> ("Cfg.Dirs.Config"=w694:path)
                  n330 = local read "SpeakerCalFile"() -> (w702:path)
                  n331 = Unbundle By Name(w703) -> ("SampleRate"=w707:dbl)
                  n332 = Unbundle By Name(w698) -> ("SavWav"=w697:bool)
                  n333 = Build Path(base path=w694, name or relative path="Waveforms") -> (appended path=w693:path)
                  n334 = call <vilib>:"File.Create Folder if Does Not Exist.vi"("Path"=w693) -> ("Dup Path"=w692:path)  [unwired: 8 in, 2 out]
                  n335 = call "Audio Test.Generate Sine Sweep, Finite Steps.vi"("Cal Data"=w702, "Sine Sweep Params"=w703) -> ("error out"=w699:errorcluster, "Total Samples"=→"Total Samples":i32, "Output Wvfrm"=w705:waveform(dbl), "SigConfig"=w706:refnum<class "SV Discrete Sweep.lvclass">, "Cal Output Wvfrm"=w701:waveform(dbl))  [unwired: 5 in]
                  "Graph Sine Sweep" <- w705
                  n336 = Bundle By Name(cluster=T21 {"sample rate (S/s)"=22050.0, "number of channels"=2, "bits per sample"=16} ("sound format"), "sample rate (S/s)"=w707, "number of channels"=1, "bits per sample"=16) -> (w710:T21)
                  n337 = Build Path(base path=w692, name or relative path="Sine Sweep.wav") -> (appended path=w700:path)
                  n338 = case shown="False" w697 {
                    tunnel: w710 -> [_ w721]
                    tunnel: w705 -> [_ w719]
                    tunnel: w700 -> [_ w717]
                    tunnel: w699 -> [_ w718]
                    tunnel: [_ w717] -> w696
                    frame False {
                    }
                    frame True {
                      n339 = call-poly <vilib>:"Sound File Open.vi"("error in (no error)"=w718, "sound format"=w721, "path"=w717) -> ("error out"=w723:errorcluster, "sound file refnum"=w725:T39)  [unwired: 7 in]
                      n340 = call-poly <vilib>:"Sound File Write.vi"("error in (no error)"=w723, "data"=w719, "sound file refnum"=w725) -> ("error out"=w722:errorcluster, "sound file refnum out"=w724:T39)  [unwired: 7 in]
                      n341 = call <vilib>:"Sound File Close.vi"("error in (no error)"=w722, "sound file refnum"=w724) -> ("error out"=w720:errorcluster)  [unwired: 9 in]
                      n342 = call <vilib>:"Clear Errors.vi"("error in (no error)"=w720) -> ()  [unwired: 5 in, 2 out]
                    }
                  }
                  "Sine Sweep" <- w696
                  n343 = Bundle By Name(cluster=w715, "SigConfig"=w706, "Sweep"=w705, "SweepCal"=w701) -> (w714:cluster{})
                }
                frame "Cal Sweep" {
                  n344 = local read "Sine Sweep Params"() -> (w736:T7)
                  n345 = Unbundle By Name(w735) -> ("Cfg.Dirs.Config"=w728:path)
                  n346 = Unbundle By Name(w736) -> ("SampleRate"=w737:dbl)
                  n347 = Unbundle By Name(w734) -> ("SweepCal"=w733)
                  "Graph Sine Sweep Cal" <- w733
                  n348 = Unbundle By Name(w731) -> ("SavWav"=w730:bool)
                  n349 = Bundle By Name(cluster=T21 {"sample rate (S/s)"=22050.0, "number of channels"=2, "bits per sample"=16} ("sound format"), "sample rate (S/s)"=w737, "number of channels"=1, "bits per sample"=16) -> (w740:T21)
                  n350 = Build Path(base path=w728, name or relative path="Waveforms") -> (appended path=w726:path)
                  n351 = Build Path(base path=w726, name or relative path="Sound Sweep Cal.wav") -> (appended path=w732:path)
                  n352 = case shown="True" w730 {
                    tunnel: w740 -> [_ w747]
                    tunnel: w733 -> [_ w745]
                    tunnel: w732 -> [_ w744]
                    tunnel: [_ w744] -> w729
                    frame False {
                    }
                    frame True {
                      n353 = call-poly <vilib>:"Sound File Open.vi"("sound format"=w747, "path"=w744) -> ("error out"=w749:errorcluster, "sound file refnum"=w751:T39)  [unwired: 8 in]
                      n354 = call-poly <vilib>:"Sound File Write.vi"("error in (no error)"=w749, "data"=w745, "sound file refnum"=w751) -> ("error out"=w748:errorcluster, "sound file refnum out"=w750:T39)  [unwired: 7 in]
                      n355 = call <vilib>:"Sound File Close.vi"("error in (no error)"=w748, "sound file refnum"=w750) -> ("error out"=w746:errorcluster)  [unwired: 9 in]
                      n356 = call <vilib>:"Clear Errors.vi"("error in (no error)"=w746) -> ()  [unwired: 5 in, 2 out]
                    }
                  }
                  "Sine Sweep Cal" <- w729
                }
                frame "Play Sweep" {
                  n357 = case shown="True" TRUE {
                    tunnel: w758 -> [w765 w771]
                    tunnel: [_ w776] -> w757
                    tunnel: [_ w775] -> w756
                    tunnel: [w770 w774] -> w754
                    tunnel: [w768 _] -> _
                    tunnel: [w766 w771] -> w752
                    frame False {
                      n358 = call <vilib>:"Sound File Read Simple.vi"("path"=path "C:/MTE/Utah Core Audio Test/Data/Sample/Stimulus_20181102_135435.wav") -> ("data"=w763:waveform(dbl)[])  [unwired: 7 in, 3 out]
                      n359 = call <vilib>:"Sound File Read Simple.vi"("path"=path "C:/MTE/Utah Core Audio Test/Data/Sample/Mic Capture_20181102_135435.wav") -> ("error out"=w768:errorcluster, "data"=w769:waveform(dbl)[])  [unwired: 7 in, 2 out]
                      n360 = Index Array(array=w763) -> (element=w762:waveform(dbl))  [unwired: 1 in]
                      n361 = Index Array(array=w769) -> (element=w770:waveform(dbl))  [unwired: 1 in]
                      n362 = Bundle By Name(cluster=w765, "Sweep"=w762) -> (w766:cluster{})
                    }
                    frame True {
                      n363 = local read "Sine Sweep Params"() -> (w779:T7)
                      n364 = local read "Play Volume"() -> (w777:dbl)
                      n365 = Unbundle By Name(w771) -> ("SweepCal"=w780)
                      n366 = Unbundle By Name(w779) -> ("SampleRate"=w778:dbl)
                      n367 = call "AudioTest.Play_Record.vi"("Record Device ID"="Input Device", "Play Device ID"="Output Device", "Sample Rate (Hz)"=w778, "volume"=w777, "Stimulus Wvfrm"=w780) -> ("Error Out"=w775:errorcluster, "PlayDur(s)"=w776:dbl, "Recorded Wvfrm"=w774:waveform(dbl))  [unwired: 4 in]
                    }
                  }
                  "PlayDur(s)" <- w757
                  n368 = case shown="No Error" w756 {
                    selector: w756 -> [_ w789]
                    tunnel: [w781 w789] -> w755
                    tunnel: w754 -> [w785 _]
                    frame No Error {
                      n369 = Unbundle By Name(w785) -> ("Y"=w784:dbl[])
                      n370 = Array Size(array=w784) -> (size(s)=w783:i32)
                      n371 = Equal To 0?(x=w783) -> (x = 0?=w782:bool)
                      n372 = case shown="True" w782 {
                        tunnel: [_ w786] -> w781
                        frame False {
                        }
                        frame True {
                          w787 = T37 -5600 items=["No Error"=0, "Abort"=-2, "Misc"=-5000, "Fixture Error"=-5100, "File IO - General"=-5200, "FIle IO - Config Error"=-5201, "Instrument - General"=-5300, "Instrument - Serial Com"=-5301, "Instrument - Camera"=-5302, "Instrument - PS"=-5303, "Instrument - Oscilloscope"=-5304, "Instrument - Function Gen"=-5305, "Instrument - Load"=-5306, "Instrument - Meter"=-5307, "Instrument - Power Control"=-5308, "Instrument - Motion"=-5309, "Instrument - RF"=-5310, "System Exe"=-5400, "Image Processing"=-5500, "Communication"=-5600, "Script - Syntax Error"=-6000, "Script - Invalid Name or Param"=-6100, "Script - Timeout"=-6200, "Invalid Data"=-6300, "FW Update Error"=-6500] ("Std Code")
                          n373 = call "Error.Set Error.vi"("Code"=w787, "Desc"="Error, no Microphone data captured.") -> ("error out"=w786:errorcluster)  [unwired: 5 in]
                        }
                      }
                    }
                    frame Error {
                    }
                  }
                  n374 = Bundle By Name(cluster=w752, "Mic"=w754) -> (w759:cluster{})
                }
                frame "Calculate Data" {
                  n375 = Unbundle By Name(w802) -> ("SigConfig"=w795, "Sweep"=w806, "Mic"=w799)
                  n376 = local read "Sine Sweep Params"() -> (w794:T7)
                  n377 = local read "Mic Test Setup"() -> (w809:T3)
                  n378 = local read "AvgLevelParams"() -> (w805:T5)
                  n379 = Unbundle By Name(w791) -> ("SavWav"=w790:bool)
                  n380 = Unbundle By Name(w809) -> ("Mic Side"=w808:enum32{"LEFT", "RIGHT"}, "Covered"=w807:bool)
                  n381 = local read "UUT Dir"() -> (w798:path)
                  n382 = Unbundle By Name(w794) -> ("StepCnt"=w793:i32)
                  n383 = call "Audio Test.Stepped Sine Sweep Analysis.vi"("SigConfig"=w795, "StepCnt"=w793, "Response Wvfrm"=w799, "Stimulus Wvfrm"=w806) -> ("error out"=w792:errorcluster, "THD"=w800:cluster{"frequency":dbl[], "THD":dbl[]}, "Magnitude"=w801:cluster{"frequency":dbl[], "magnitude":dbl[]})  [unwired: 5 in]
                  n384 = call "AudioTest.Calculate Average Mag.vi"("Average Level Calculation"=w805, "Magnitude"=w801) -> ("Average Mag"=w804:dbl)  [unwired: 9 in]
                  n385 = case shown="\"LEFT\", Default" w808 {
                    tunnel: w807 -> [w814 w829]
                    tunnel: w799 -> [w812 w828]
                    tunnel: [w813 w827] -> w797
                    tunnel: w798 -> [w811 w826]
                    tunnel: w790 -> [w810 w825]
                    frame "LEFT", Default {
                      n386 = case shown="True" w814 {
                        tunnel: w812 -> [w819 w824]
                        tunnel: [w818 w822] -> w813
                        tunnel: w811 -> [w817 w821]
                        tunnel: w810 -> [w815 w823]
                        frame False {
                          w818 = "Left Uncovered"
                          n387 = call "AudioTest.Save Waveform to CSV File.vi"("Enable"=w815, "Root Name"=w818, "Folder"=w817, "Waveform"=w819) -> ("Path"=→"Left Mic Raw":path)  [unwired: 7 in]
                          "Graph Left Uncovered" <- w819
                        }
                        frame True {
                          w822 = "Left Covered"
                          n388 = call "AudioTest.Save Waveform to CSV File.vi"("Enable"=w823, "Root Name"=w822, "Folder"=w821, "Waveform"=w824) -> ("Path"=→"Left Mic Covered Raw":path)  [unwired: 7 in]
                          "Graph Left Covered" <- w824
                        }
                      }
                    }
                    frame "RIGHT" {
                      n389 = case shown="True" w829 {
                        tunnel: w828 -> [w833 w838]
                        tunnel: [w834 w839] -> w827
                        tunnel: w826 -> [w832 w837]
                        tunnel: w825 -> [w831 w835]
                        frame False {
                          w834 = "Right Uncovered"
                          n390 = call "AudioTest.Save Waveform to CSV File.vi"("Enable"=w831, "Root Name"=w834, "Folder"=w832, "Waveform"=w833) -> ("Path"=→"Right Mic Raw":path)  [unwired: 7 in]
                          "Graph Right Uncovered" <- w833
                        }
                        frame True {
                          w839 = "Right Covered"
                          n391 = call "AudioTest.Save Waveform to CSV File.vi"("Enable"=w835, "Root Name"=w839, "Folder"=w837, "Waveform"=w838) -> ("Path"=→"Right Mic Covered Raw":path)  [unwired: 7 in]
                          "Graph Right Covered" <- w838
                        }
                      }
                    }
                  }
                  n392 = Bundle By Name(cluster=w802, "AvgMag"=w804, "Mag"=w801, "THD"=w800, "TestName"=w797) -> (w803:cluster{})
                }
                frame "Process Data" {
                  n393 = local read "R AvgMagCov"() -> (w840:dbl)
                  n394 = local read "L AvgMagCov"() -> (w841:dbl)
                  n395 = Unbundle By Name(w845) -> ("TestName"=w852, "Mag"=w851)
                  n396 = Unbundle By Name(w845) -> ("AvgMag"=w844)
                  n397 = Unbundle By Name(w846) -> ("THD Lim"=w842:cluster{"LL":T22, "UL":T22})
                  n398 = Unbundle By Name(w846) -> ("FR Lim"=w850:cluster{"LL":T22, "UL":T22})
                  n399 = Unbundle By Name(w845) -> ("THD"=w843)
                  n400 = case shown="\"Left Covered\"" w852 {
                    tunnel: w851 -> [_ w865 w977 w1089 w1131]
                    tunnel: w850 -> [_ w864 w976 w1088 w1130]
                    tunnel: w845 -> [w853 w863 w975 w1087 w1129]
                    tunnel: w846 -> [w854 w862 w974 w1086 w1128]
                    tunnel: [w854 w861 w973 w1085 w1127] -> w849
                    tunnel: [w853 w860 w972 w1084 w1126] -> w847
                    tunnel: w844 -> [_ w859 w971 w1083 w1125]
                    tunnel: w843 -> [_ w858 w970 w1082 w1124]
                    tunnel: w842 -> [_ w857 w969 w1081 w1123]
                    tunnel: w841 -> [_ w856 w968 w1080 w1122]
                    tunnel: w840 -> [_ w855 w967 w1079 w1121]
                    frame Default {
                    }
                    frame "Left Uncovered" {
                      n401 = while {
                        tunnel: w865 -> [w878]
                        tunnel: w864 -> [w877]
                        shift-right: [w873] -> w860
                        shift-left: w863 -> [w875]
                        shift-right: [w874] -> w861
                        shift-left: w862 -> [w876]
                        tunnel: w859 -> [w871]
                        tunnel: w858 -> [w870]
                        tunnel: w857 -> [w869]
                        tunnel: w856 -> [w867]
                        tunnel: w855 -> [w866]
                        i -> [w872]
                        stop <- w868 stop-if-true
                        n402 = case shown="0" w872 {
                          tunnel: w878 -> [w882 _ w907 _ _ _]
                          tunnel: w877 -> [w888 _ w922 _ _ _]
                          tunnel: w876 -> [w887 w901 w926 w936 w960 w964]
                          tunnel: w875 -> [w886 w900 w928 w947 w963 w966]
                          tunnel: [w887 w901 w927 w946 w962 w964] -> w874
                          tunnel: [w886 w900 w928 w947 w963 w966] -> w873
                          tunnel: w871 -> [w881 _ w906 _ w955 _]
                          tunnel: w870 -> [_ w894 _ w933 _ _]
                          tunnel: w869 -> [_ w897 _ w934 _ _]
                          tunnel: [_ _ _ _ _ TRUE] -> w868
                          tunnel: w867 -> [_ _ _ _ w958 _]
                          tunnel: w866 -> [_ _ _ _ _ _]
                          frame 0 {
                            n403 = local read "Left Mic Covered FR"() -> (w883:cluster{"F":dbl[], "M":dbl[]})
                            n404 = Unbundle By Name(w888) -> ("UL.X"=w890:dbl[], "UL.Y"=w889:dbl[])
                            n405 = Unbundle By Name(w888) -> ("LL.X"=w892:dbl[], "LL.Y"=w891:dbl[])
                            n406 = Bundle("X"=w890, "Y"=w889) -> (w885:cluster{"X":dbl[], "Y":dbl[]})  [unwired: 1 in]
                            n407 = Bundle("X"=w892, "Y"=w891) -> (w884:cluster{"X":dbl[], "Y":dbl[]})  [unwired: 1 in]
                            n408 = call "AudioTest.Normalize DB Plot.vi"("Avg DB"=w881, "Plot DB"=w883) -> ("Norm Plot"=w879:cluster{"F":dbl[], "M":dbl[]})  [unwired: 9 in]
                            n409 = call "AudioTest.Normalize DB Plot.vi"("Avg DB"=w881, "Plot DB"=w882) -> ("Norm Plot"=w880:cluster{"F":dbl[], "M":dbl[]})  [unwired: 9 in]
                            n410 = Build Array(w880, w879, w884, w885) -> (→"Left Freq Response":cluster{"X":dbl[], "Y":dbl[]}[])
                          }
                          frame 1 {
                            n411 = Unbundle By Name(w897) -> ("UL.X"=w898:dbl[], "UL.Y"=w899:dbl[])
                            n412 = Bundle("X"=w898, "Y"=w899) -> (w895:cluster{"X":dbl[], "Y":dbl[]})  [unwired: 1 in]
                            n413 = Build Array(w894, w895) -> (→"Left Mic THD":cluster{"X":dbl[], "Y":dbl[]}[])
                          }
                          frame 2 {
                            n414 = call "AudioTest.Normalize DB Plot.vi"("Avg DB"=w906, "Plot DB"=w907) -> ("Norm Plot"=w908:cluster{"F":dbl[], "M":dbl[]})  [unwired: 9 in]
                            n415 = Unbundle By Name(w908) -> ("F"=w917:dbl[], "M"=w916:dbl[])
                            n416 = Unbundle By Name(w922) -> ("LL"=w912:T22, "UL"=w910:T22)
                            n417 = Bundle By Name(cluster=w912, "Result Name"="Left Freq Resp LL") -> (w911:T22)
                            n418 = Bundle By Name(cluster=w910, "Result Name"="Left Freq Resp UL") -> (w909:T22)
                            n419 = Bundle By Name(cluster=T22 {"Order"=0, "Name"="", "X"=[], "Y"=[], "X Units"="", "Y Units"="", "LimitType"=enum."None", "FailCode"=0, "FailDesc"="", "Ref Data Name"="", "Result Name"="", "0dB Level"=0.0, "Normalized"=FALSE} ("Plot Data"), "Name"="Left Freq Resp", "X"=w917, "Y"=w916, "X Units"="Hz", "Y Units"="dB") -> (w915:T22)
                            n420 = call "AudioTest.Compare Plot to Limit.vi"("Plot Limit"=w911, "Plot Data"=w915) -> ("Result Color"=w905:u32, "Meas Rslt"=w925:T17[], "PASS"=w904:bool)  [unwired: 6 in, 1 out]
                            n421 = call "AudioTest.Compare Plot to Limit.vi"("Plot Limit"=w909, "Plot Data"=w915) -> ("Result Color"=w903:u32, "Meas Rslt"=w924:T17[])  [unwired: 6 in, 2 out]
                            n422 = Build Array (concatenate)(w925, w924) -> (w923:T17[])
                            n423 = Select(t=w903, s=w904, f=w905) -> (s? t:f=→"LFRColor":u32)
                            n424 = Bundle By Name(cluster=w926, "Rslt.Meas"=w923) -> (w927:T36)
                          }
                          frame 3 {
                            n425 = Unbundle By Name(w933) -> ("F"=w939, "M"=w938)
                            n426 = Unbundle By Name(w934) -> ("UL"=w931:T22)
                            n427 = Bundle By Name(cluster=T22 {"Order"=0, "Name"="", "X"=[], "Y"=[], "X Units"="", "Y Units"="", "LimitType"=enum."None", "FailCode"=0, "FailDesc"="", "Ref Data Name"="", "Result Name"="", "0dB Level"=0.0, "Normalized"=FALSE} ("Plot Data"), "Name"="Left THD", "X"=w939, "Y"=w938, "X Units"="Hz", "Y Units"="dB") -> (w937:T22)
                            n428 = Bundle By Name(cluster=w931, "Result Name"="Left THD UL") -> (w930:T22)
                            n429 = Unbundle By Name(w936) -> ("Rslt.Meas"=w935:T17[])
                            n430 = call "AudioTest.Compare Plot to Limit.vi"("Plot Limit"=w930, "Plot Data"=w937) -> ("Result Color"=→"LThdColor":u32, "Meas Rslt"=w945:T17[])  [unwired: 6 in, 2 out]
                            n431 = Build Array (concatenate)(w935, w945) -> (w944:T17[])
                            n432 = Bundle By Name(cluster=w936, "Rslt.Meas"=w944) -> (w946:T36)
                          }
                          frame 4 {
                            n433 = local read "Limits"() -> (w951:T4)
                            n434 = Subtract(x=w955, y=w958) -> (x-y=w956:dbl)
                            "L AvgMag Delta" <- w956
                            n435 = Unbundle By Name(w951) -> ("AvgLevelLL_dBFS"=w950:dbl, "AvgLevelUL_dBFS"=w949:dbl, "CoveredMicAttn_dB"=w948:dbl)
                            n436 = Unbundle By Name(w960) -> ("Rslt.Meas"=w959:T17[])
                            n437 = call "AudioTest.Create Mic Level and Attenuation Result.vi"("Delta LL"=w948, "Delta"=w956, "Level UL"=w949, "Level LL"=w950, "Level"=w955, "Side"="Left" ("Category")) -> ("Delta Color"=w952:u32, "Level Color"=w953:u32, "Data"=w957:T17[])  [unwired: 3 in]
                            n438 = Build Array (concatenate)(w959, w957) -> (w961:T17[])
                            n439 = property on="L AvgMagUnCov" class="DigNum (strict)"("NumText.BGColor"=w953) -> ()  [unwired: 2 in, 2 out]
                            n440 = property on="L AvgMag Delta" class="DigNum (strict)"("NumText.BGColor"=w952) -> ()  [unwired: 2 in, 2 out]
                            n441 = Bundle By Name(cluster=w960, "Rslt.Meas"=w961) -> (w962:T36)
                            "L AvgMagUnCov" <- w955
                          }
                          frame Default {
                          }
                        }
                      }
                    }
                    frame "Right Uncovered" {
                      n442 = while {
                        tunnel: w977 -> [w990]
                        tunnel: w976 -> [w989]
                        shift-right: [w985] -> w972
                        shift-left: w975 -> [w987]
                        shift-right: [w986] -> w973
                        shift-left: w974 -> [w988]
                        tunnel: w971 -> [w983]
                        tunnel: w970 -> [w982]
                        tunnel: w969 -> [w981]
                        tunnel: w968 -> [w979]
                        tunnel: w967 -> [w978]
                        i -> [w984]
                        stop <- w980 stop-if-true
                        n443 = case shown="4" w984 {
                          tunnel: w990 -> [w993 _ w1019 _ _ _]
                          tunnel: w989 -> [w999 _ w1034 _ _ _]
                          tunnel: w988 -> [w998 w1013 w1038 w1048 w1072 w1076]
                          tunnel: w987 -> [w997 w1012 w1040 w1059 w1075 w1078]
                          tunnel: [w998 w1013 w1039 w1058 w1074 w1076] -> w986
                          tunnel: [w997 w1012 w1040 w1059 w1075 w1078] -> w985
                          tunnel: w983 -> [w994 _ w1018 _ w1062 _]
                          tunnel: w982 -> [_ w1007 _ w1045 _ _]
                          tunnel: w981 -> [_ w1009 _ w1046 _ _]
                          tunnel: [_ _ _ _ _ TRUE] -> w980
                          tunnel: w979 -> [_ _ _ _ _ _]
                          tunnel: w978 -> [_ _ _ _ w1070 _]
                          frame 0 {
                            n444 = local read "Right Mic Covered FR"() -> (w995:cluster{"F":dbl[], "M":dbl[]})
                            n445 = Unbundle By Name(w999) -> ("UL.X"=w1003:dbl[], "UL.Y"=w1002:dbl[])
                            n446 = Unbundle By Name(w999) -> ("LL.X"=w1005:dbl[], "LL.Y"=w1004:dbl[])
                            n447 = call "AudioTest.Normalize DB Plot.vi"("Avg DB"=w994, "Plot DB"=w995) -> ("Norm Plot"=w991:cluster{"F":dbl[], "M":dbl[]})  [unwired: 9 in]
                            n448 = call "AudioTest.Normalize DB Plot.vi"("Avg DB"=w994, "Plot DB"=w993) -> ("Norm Plot"=w992:cluster{"F":dbl[], "M":dbl[]})  [unwired: 9 in]
                            n449 = Bundle("X"=w1003, "Y"=w1002) -> (w1000:cluster{"X":dbl[], "Y":dbl[]})  [unwired: 1 in]
                            n450 = Bundle("X"=w1005, "Y"=w1004) -> (w1001:cluster{"X":dbl[], "Y":dbl[]})  [unwired: 1 in]
                            n451 = Build Array(w992, w991, w1001, w1000) -> (→"Right Freq Response":cluster{"X":dbl[], "Y":dbl[]}[])
                          }
                          frame 1 {
                            n452 = Unbundle By Name(w1009) -> ("UL.X"=w1010:dbl[], "UL.Y"=w1011:dbl[])
                            n453 = Bundle("X"=w1010, "Y"=w1011) -> (w1008:cluster{"X":dbl[], "Y":dbl[]})  [unwired: 1 in]
                            n454 = Build Array(w1007, w1008) -> (→"Right Mic THD":cluster{"X":dbl[], "Y":dbl[]}[])
                          }
                          frame 2 {
                            n455 = call "AudioTest.Normalize DB Plot.vi"("Avg DB"=w1018, "Plot DB"=w1019) -> ("Norm Plot"=w1020:cluster{"F":dbl[], "M":dbl[]})  [unwired: 9 in]
                            n456 = Unbundle By Name(w1034) -> ("LL"=w1025:T22, "UL"=w1022:T22)
                            n457 = Unbundle By Name(w1020) -> ("F"=w1029:dbl[], "M"=w1028:dbl[])
                            n458 = Bundle By Name(cluster=w1022, "Result Name"="Right Freq Resp UL") -> (w1021:T22)
                            n459 = Bundle By Name(cluster=w1025, "Result Name"="Right Freq Resp LL") -> (w1024:T22)
                            n460 = Bundle By Name(cluster=T22 {"Order"=0, "Name"="", "X"=[], "Y"=[], "X Units"="", "Y Units"="", "LimitType"=enum."None", "FailCode"=0, "FailDesc"="", "Ref Data Name"="", "Result Name"="", "0dB Level"=0.0, "Normalized"=FALSE} ("Plot Data"), "Name"="Right Freq Resp", "X"=w1029, "Y"=w1028, "X Units"="Hz", "Y Units"="dB") -> (w1027:T22)
                            n461 = call "AudioTest.Compare Plot to Limit.vi"("Plot Limit"=w1024, "Plot Data"=w1027) -> ("Result Color"=w1016:u32, "Meas Rslt"=w1037:T17[], "PASS"=w1017:bool)  [unwired: 6 in, 1 out]
                            n462 = call "AudioTest.Compare Plot to Limit.vi"("Plot Limit"=w1021, "Plot Data"=w1027) -> ("Result Color"=w1015:u32, "Meas Rslt"=w1036:T17[])  [unwired: 6 in, 2 out]
                            n463 = Select(t=w1015, s=w1017, f=w1016) -> (s? t:f=→"RtFRColor":u32)
                            n464 = Build Array (concatenate)(w1037, w1036) -> (w1035:T17[])
                            n465 = Bundle By Name(cluster=w1038, "Rslt.Meas"=w1035) -> (w1039:T36)
                          }
                          frame 3 {
                            n466 = Unbundle By Name(w1045) -> ("F"=w1051, "M"=w1050)
                            n467 = Unbundle By Name(w1046) -> ("UL"=w1043:T22)
                            n468 = Bundle By Name(cluster=T22 {"Order"=0, "Name"="", "X"=[], "Y"=[], "X Units"="", "Y Units"="", "LimitType"=enum."None", "FailCode"=0, "FailDesc"="", "Ref Data Name"="", "Result Name"="", "0dB Level"=0.0, "Normalized"=FALSE} ("Plot Data"), "Name"="Right THD", "X"=w1051, "Y"=w1050, "X Units"="Hz", "Y Units"="dB") -> (w1049:T22)
                            n469 = Bundle By Name(cluster=w1043, "Result Name"="Right THD UL") -> (w1042:T22)
                            n470 = Unbundle By Name(w1048) -> ("Rslt.Meas"=w1047:T17[])
                            n471 = call "AudioTest.Compare Plot to Limit.vi"("Plot Limit"=w1042, "Plot Data"=w1049) -> ("Result Color"=→"RtThdColor":u32, "Meas Rslt"=w1057:T17[])  [unwired: 6 in, 2 out]
                            n472 = Build Array (concatenate)(w1047, w1057) -> (w1056:T17[])
                            n473 = Bundle By Name(cluster=w1048, "Rslt.Meas"=w1056) -> (w1058:T36)
                          }
                          frame 4 {
                            n474 = local read "Limits"() -> (w1067:T4)
                            n475 = Subtract(x=w1062, y=w1070) -> (x-y=w1061:dbl)
                            "R AvgMag Delta" <- w1061
                            n476 = Unbundle By Name(w1067) -> ("AvgLevelLL_dBFS"=w1066:dbl, "AvgLevelUL_dBFS"=w1065:dbl, "CoveredMicAttn_dB"=w1064:dbl)
                            n477 = Unbundle By Name(w1072) -> ("Rslt.Meas"=w1071:T17[])
                            n478 = call "AudioTest.Create Mic Level and Attenuation Result.vi"("Delta LL"=w1064, "Delta"=w1061, "Level UL"=w1065, "Level LL"=w1066, "Level"=w1062, "Side"="Right" ("Category")) -> ("Delta Color"=w1068:u32, "Level Color"=w1069:u32, "Data"=w1060:T17[])  [unwired: 3 in]
                            n479 = Build Array (concatenate)(w1071, w1060) -> (w1073:T17[])
                            n480 = property on="R AvgMagUnCov" class="DigNum (strict)"("NumText.BGColor"=w1069) -> ()  [unwired: 2 in, 2 out]
                            n481 = property on="R AvgMag Delta" class="DigNum (strict)"("NumText.BGColor"=w1068) -> ()  [unwired: 2 in, 2 out]
                            n482 = Bundle By Name(cluster=w1072, "Rslt.Meas"=w1073) -> (w1074:T36)
                            "R AvgMagUnCov" <- w1062
                          }
                          frame Default {
                          }
                        }
                      }
                    }
                    frame "Left Covered" {
                      n483 = while {
                        tunnel: w1089 -> [w1102]
                        tunnel: w1088 -> [w1101]
                        shift-right: [w1097] -> w1084
                        shift-left: w1087 -> [w1099]
                        shift-right: [w1098] -> w1085
                        shift-left: w1086 -> [w1100]
                        tunnel: w1083 -> [w1095]
                        tunnel: w1082 -> [w1094]
                        tunnel: w1081 -> [w1093]
                        tunnel: w1080 -> [w1091]
                        tunnel: w1079 -> [w1090]
                        i -> [w1096]
                        stop <- w1092 stop-if-true
                        n484 = case shown="1" w1096 {
                          tunnel: w1102 -> [w1103 _ _]
                          tunnel: w1101 -> [_ _ _]
                          tunnel: w1100 -> [w1105 w1114 w1118]
                          tunnel: w1099 -> [w1104 w1117 w1120]
                          tunnel: [w1105 w1116 w1118] -> w1098
                          tunnel: [w1104 w1117 w1120] -> w1097
                          tunnel: w1095 -> [_ w1107 _]
                          tunnel: w1094 -> [_ _ _]
                          tunnel: w1093 -> [_ _ _]
                          tunnel: [_ _ TRUE] -> w1092
                          tunnel: w1091 -> [_ _ _]
                          tunnel: w1090 -> [_ _ _]
                          frame 0 {
                            "Left Mic Covered FR" <- w1103
                          }
                          frame 1 {
                            n485 = call "String.Float to String, Small Profile.vi"("Numeric"=w1107) -> ("String"=w1106:string)  [unwired: 10 in]
                            n486 = Unbundle By Name(w1114) -> ("Rslt.Meas"=w1113:T17[])
                            n487 = Bundle By Name(cluster=T17 {"Cnt"=0, "Step"="", "Category"="", "Name"="", "Value"="", "Units"="", "LimType"="", "LL"="", "UL"="", "Status"=0, "Code"=0, "Desc"="", "Time"=timestamp(0 s since 1904-01-01)} ("Meas"), "Category"="Level", "Name"="Left Covered Avg Level" ("Category"), "Value"=w1106, "Units"="dB") -> (w1109:T17)
                            n488 = Build Array (concatenate)(w1113, w1109) -> (w1115:T17[])
                            n489 = Bundle By Name(cluster=w1114, "Rslt.Meas"=w1115) -> (w1116:T36)
                            "L AvgMagCov" <- w1107
                          }
                          frame Default {
                          }
                        }
                      }
                    }
                    frame "Right Covered" {
                      n490 = while {
                        tunnel: w1131 -> [w1144]
                        tunnel: w1130 -> [w1143]
                        shift-right: [w1139] -> w1126
                        shift-left: w1129 -> [w1141]
                        shift-right: [w1140] -> w1127
                        shift-left: w1128 -> [w1142]
                        tunnel: w1125 -> [w1137]
                        tunnel: w1124 -> [w1136]
                        tunnel: w1123 -> [w1135]
                        tunnel: w1122 -> [w1133]
                        tunnel: w1121 -> [w1132]
                        i -> [w1138]
                        stop <- w1134 stop-if-true
                        n491 = case shown="1" w1138 {
                          tunnel: w1144 -> [w1145 _ _]
                          tunnel: w1143 -> [_ _ _]
                          tunnel: w1142 -> [w1147 w1156 w1160]
                          tunnel: w1141 -> [w1146 w1159 w1162]
                          tunnel: [w1147 w1158 w1160] -> w1140
                          tunnel: [w1146 w1159 w1162] -> w1139
                          tunnel: w1137 -> [_ w1148 _]
                          tunnel: w1136 -> [_ _ _]
                          tunnel: w1135 -> [_ _ _]
                          tunnel: [_ _ TRUE] -> w1134
                          tunnel: w1133 -> [_ _ _]
                          tunnel: w1132 -> [_ _ _]
                          frame 0 {
                            "Right Mic Covered FR" <- w1145
                          }
                          frame 1 {
                            n492 = call "String.Float to String, Small Profile.vi"("Numeric"=w1148) -> ("String"=w1149:string)  [unwired: 10 in]
                            n493 = Unbundle By Name(w1156) -> ("Rslt.Meas"=w1155:T17[])
                            n494 = Bundle By Name(cluster=T17 {"Cnt"=0, "Step"="", "Category"="", "Name"="", "Value"="", "Units"="", "LimType"="", "LL"="", "UL"="", "Status"=0, "Code"=0, "Desc"="", "Time"=timestamp(0 s since 1904-01-01)} ("Meas"), "Category"="Level", "Name"="Right Covered Avg Level" ("Category"), "Value"=w1149, "Units"="dB") -> (w1150:T17)
                            n495 = Build Array (concatenate)(w1155, w1150) -> (w1157:T17[])
                            n496 = Bundle By Name(cluster=w1156, "Rslt.Meas"=w1157) -> (w1158:T36)
                            "R AvgMagCov" <- w1148
                          }
                          frame Default {
                          }
                        }
                      }
                    }
                  }
                }
                frame "Results" {
                  n497 = local read "Sine Sweep Params"() -> (w1168:T7)
                  n498 = local read "Mic Test Setup"() -> (w1170:T3)
                  n499 = Unbundle By Name(w1178) -> ("Rslt.Meas"=w1163:T17[])
                  n500 = Unbundle By Name(w1170) -> ("Mic Side"=w1169:enum32{"LEFT", "RIGHT"})
                  n501 = Unbundle By Name(w1168) -> ("FreqStart"=w1165:dbl, "FreqEnd"=w1164:dbl)
                  n502 = call "Result.Attributes plus Numeric into Results Table.vi"("Meas"=w1163) -> ("Results Table"=w1177:T2[])  [unwired: 10 in]
                  n503 = Unbundle By Name(w1173) -> ("TestName"=w1172)
                  n504 = for {
                    tunnel: w1177 -> [w1187] mode=indexing
                    tunnel: [w1184] -> w1174 mode=indexing
                    i -> [w1185]
                    n505 = Number To Decimal String(number=w1185) -> (decimal integer string=w1186:string)  [unwired: 1 in]
                    n506 = Bundle By Name(cluster=w1187, "Step"=w1186, "Cnt"=w1185) -> (w1184:T2)
                  }
                  n507 = Max & Min(x=w1165, y=w1164) -> (max(x,y)=w1166:dbl, min(x,y)=w1167:dbl)
                  n508 = case shown="\"RIGHT\"" w1169 {
                    tunnel: w1167 -> [w1181 w1182]
                    tunnel: w1166 -> [w1180 w1183]
                    frame "LEFT", Default {
                      n509 = property on="Left Freq Response" class="XYGraph (strict)"("XScale.Maximum"=w1180, "XScale.Minimum"=w1181) -> ()  [unwired: 2 in, 2 out]
                      n510 = property on="Left Mic THD" class="XYGraph (strict)"("XScale.Maximum"=w1180, "XScale.Minimum"=w1181) -> ()  [unwired: 2 in, 2 out]
                    }
                    frame "RIGHT" {
                      n511 = property on="Right Freq Response" class="XYGraph (strict)"("XScale.Maximum"=w1183, "XScale.Minimum"=w1182) -> ()  [unwired: 2 in, 2 out]
                      n512 = property on="Right Mic THD" class="XYGraph (strict)"("XScale.Maximum"=w1183, "XScale.Minimum"=w1182) -> ()  [unwired: 2 in, 2 out]
                    }
                  }
                  n513 = local read "UUT Dir"() -> (w1171:path)
                  n514 = local write "Results Table"(w1174) -> ()
                  n515 = call "AudioTest.Result Table to CSV Measurements File.vi"("Results Table"=w1174, "Test Name"=w1172, "UUT Dir"=w1171) -> ("error out"=w1175:errorcluster, "Out File"=→"Measurements":path)  [unwired: 7 in]
                }
                frame "Done", Default {
                  w1188 = FALSE
                  n516 = Unbundle By Name(w1195) -> ("Start"=w1193)
                  n517 = call <vilib>:"High Resolution Relative Seconds.vi"() -> ("relative seconds"=w1194:dbl)
                  n518 = Subtract(x=w1194, y=w1193) -> (x-y=→"MicTest Dur(s)":dbl)
                  n519 = case shown="No Error" w1189 {
                    tunnel: w1191 -> [w1201 w1209]
                    tunnel: w1190 -> [_ w1205]
                    frame No Error {
                      n520 = Unbundle By Name(w1201) -> ("Log"=w1203:refnum<class "Event Notification.lvclass">)
                      n521 = call <vilib>:"Event Notification.Status Message.vi"("Display"=TRUE, "Level"=Event_Log.Log_Level."Normal", "Message"="Microphone Test Completed", "Event Notification in"=w1203) -> ()  [unwired: 8 in]
                    }
                    frame Error {
                      w1207 = TRUE ("Log")
                      n522 = Unbundle By Name(w1209) -> ("Log"=w1208:refnum<class "Event Notification.lvclass">)
                      n523 = Format Into String(format string="Error at Mic Test State %s", w1205) -> (resulting string=w1204:string)  [unwired: 2 in, 1 out]
                      n524 = call <vilib>:"Event Notification.Status Message.vi"("Display"=w1207, "Log"=w1207, "Message"=w1204, "Event Notification in"=w1208) -> ()  [unwired: 8 in]
                    }
                  }
                  n525 = property on="Test Running" class="Bool (strict)"("Blinking"=w1188, "Value"=w1188) -> ()  [unwired: 2 in, 2 out]
                }
              }
              n526 = call "Error.Case Redirect on Error.vi"("error in"=w635, "Next Case"=w637) -> ("Next Case Out"=w628:string)  [unwired: 9 in]
            }
          }
          frame "CL_Test_RTN" {
            # "Write result file"
            n527 = Unbundle By Name(w1233) -> ("CL Args.Active"=w1212:bool)
            n528 = Not(x="Stay Open after CLI") -> (.not. x?=w1210:bool)
            n529 = Unbundle By Name(w1231) -> ("SW Rev.Version"=w1230:string)
            n530 = And(x=w1210, y=w1212) -> (x .and. y?=w1211:bool)
            n531 = case shown="True" w1211 {
              tunnel: w1232 -> [_ w1236]
              frame False {
              }
              frame True {
                n532 = call <vilib>:"Q.Enqueue Exit.vi"("Q In"=w1236) -> ()  [unwired: 9 in, 2 out]
              }
            }
            n533 = local read "Error"() -> (w1227:errorcluster)
            n534 = Unbundle By Name(w1227) -> ("Status"=w1220:bool, "Code"=w1224:i32, "source"=w1225:string)
            n535 = local read "UUT Dir"() -> (w1228:path)
            n536 = Select(t="Error", s=w1220, f="Success") -> (s? t:f=w1219:string)
            n537 = Build Path(base path=w1228, name or relative path="Result.txt") -> (appended path=w1214:path)
            "Result State File" <- w1214
            n538 = Bundle By Name(cluster=w1233, "CL Args"=T24 {"Active"=FALSE, "Test"="", "Args"=[]}) -> (w1234:T36)
            n539 = Format Into String(format string="Version = %s\nResult = %s\nCode = %d\nDescription = %s", w1230, w1219, w1224, w1225) -> (resulting string=w1218:string)  [unwired: 2 in, 1 out]
            n540 = Open/Create/Replace File(file path (use dialog)=w1214, operation (0:open)=T23."replace or create") -> (refnum out=w1217:refnum<file>, error out=w1215:errorcluster)  [unwired: 4 in, 1 out]
            n541 = Write to Text File(file (use dialog)=w1217, text=w1218, error in=w1215) -> (error out=w1223:errorcluster)  [unwired: 1 in, 2 out]
            n542 = call <vilib>:"Clear Errors.vi"("error in (no error)"=w1223) -> ()  [unwired: 5 in, 2 out]
          }
          frame "Run CLI Simulation" {
            n543 = local read "Select Command Line Args"() -> (w1237:u16)
            n544 = call <vilib>:"Q.Enqueue Task.vi"("Task Name"="CL_Arg_Seq", "Q In"=w1243) -> ()  [unwired: 8 in, 2 out]
            n545 = case shown="Default" w1237 {
              tunnel: w1237 -> [w1254 _]
              tunnel: [w1253 _] -> w1241
              tunnel: [w1249 _] -> w1238
              frame Default {
                n546 = case shown="1" w1254 {
                  tunnel: [_ "MicrophoneTest" ("Action") "MicrophoneTest" ("Action") "MicrophoneTest" ("Action") "MicrophoneTest" ("Action")] -> w1253
                  tunnel: [_ string[] ["Sweep", "Left", "Covered"] string[] ["Sweep", "Right", "Covered"] string[] ["Sweep", "Left", "Uncovered"] string[] ["Sweep", "Right", "Uncovered"]] -> w1251
                  frame 0, Default {
                  }
                  frame 1 {
                  }
                  frame 2 {
                  }
                  frame 3 {
                  }
                  frame 4 {
                  }
                }
                n547 = local read "UUT Data Dir"() -> (w1250:path)
                n548 = Path To String(path=w1250) -> (string=w1252:string)
                n549 = Build Array (concatenate)(w1251, w1252) -> (w1249:string[])
              }
              frame 0 {
              }
            }
            n550 = call "String.Remove Quotes from String.vi"("1D String In"=w1238, "String In"=w1241) -> ("1D String without Quotes"=w1240:string[], "String without Quotes"=w1239:string)  [unwired: 7 in, 1 out]
            n551 = Build Array (concatenate)(w1239, w1240) -> (w1247:string[])
            n552 = local write "Args"(w1247) -> ()
            n553 = Bundle By Name(cluster=w1244, "CL Args.Active"=FALSE ("CmdLine"), "CL Args.Test"=w1239, "CL Args.Args"=w1240) -> (w1245:T36)
          }
          frame "Clear Raw Data" {
            n554 = invoke on="Left Mic Covered FR" class="XYGraph (strict)" method="Reinit To Default"() -> ()  [unwired: 3 in, 3 out]
            n555 = invoke on="Graph Left Covered" class="WFGraph (strict)" method="Reinit To Default"() -> ()  [unwired: 3 in, 3 out]
            n556 = invoke on="Graph Sine Sweep" class="WFGraph (strict)" method="Reinit To Default"() -> ()  [unwired: 3 in, 3 out]
            n557 = invoke on="Graph Left Uncovered" class="WFGraph (strict)" method="Reinit To Default"() -> ()  [unwired: 3 in, 3 out]
            n558 = invoke on="Right Mic Covered FR" class="XYGraph (strict)" method="Reinit To Default"() -> ()  [unwired: 3 in, 3 out]
            n559 = invoke on="Graph Sine Sweep Cal" class="WFGraph (strict)" method="Reinit To Default"() -> ()  [unwired: 3 in, 3 out]
            n560 = invoke on="Graph Right Covered" class="WFGraph (strict)" method="Reinit To Default"() -> ()  [unwired: 3 in, 3 out]
            n561 = invoke on="Graph Right Uncovered" class="WFGraph (strict)" method="Reinit To Default"() -> ()  [unwired: 3 in, 3 out]
          }
          frame "Clear Graphs" {
            w1265 = u32 13816530
            n562 = invoke on="L AvgMagUnCov" class="DigNum (strict)" method="Reinit To Default"() -> ()  [unwired: 3 in, 3 out]
            n563 = invoke on="L AvgMagCov" class="DigNum (strict)" method="Reinit To Default"() -> ()  [unwired: 3 in, 3 out]
            n564 = invoke on="L AvgMag Delta" class="DigNum (strict)" method="Reinit To Default"() -> ()  [unwired: 3 in, 3 out]
            n565 = invoke on="Left Freq Response" class="XYGraph (strict)" method="Reinit To Default"() -> ()  [unwired: 3 in, 3 out]
            n566 = invoke on="Left Mic THD" class="XYGraph (strict)" method="Reinit To Default"() -> ()  [unwired: 3 in, 3 out]
            n567 = invoke on="Right Mic THD" class="XYGraph (strict)" method="Reinit To Default"() -> ()  [unwired: 3 in, 3 out]
            n568 = invoke on="R AvgMagCov" class="DigNum (strict)" method="Reinit To Default"() -> ()  [unwired: 3 in, 3 out]
            n569 = invoke on="R AvgMag Delta" class="DigNum (strict)" method="Reinit To Default"() -> ()  [unwired: 3 in, 3 out]
            n570 = invoke on="R AvgMagUnCov" class="DigNum (strict)" method="Reinit To Default"() -> ()  [unwired: 3 in, 3 out]
            n571 = invoke on="Right Freq Response" class="XYGraph (strict)" method="Reinit To Default"() -> ()  [unwired: 3 in, 3 out]
            n572 = property on="L AvgMagUnCov" class="DigNum (strict)"("NumText.BGColor"=w1265) -> ()  [unwired: 2 in, 2 out]
            n573 = property on="R AvgMagUnCov" class="DigNum (strict)"("NumText.BGColor"=w1265) -> ()  [unwired: 2 in, 2 out]
            n574 = property on="R AvgMag Delta" class="DigNum (strict)"("NumText.BGColor"=w1265) -> ()  [unwired: 2 in, 2 out]
            n575 = property on="L AvgMag Delta" class="DigNum (strict)"("NumText.BGColor"=w1265) -> ()  [unwired: 2 in, 2 out]
            n576 = local write "LThdColor"(w1265) -> ()
            n577 = local write "RtFRColor"(w1265) -> ()
            n578 = local write "RtThdColor"(w1265) -> ()
            n579 = local write "LFRColor"(w1265) -> ()
          }
          frame "Config - Read", "Config - Write" {
            n580 = To Lower Case(string=w1284) -> (all lower case string=w1273:string)
            n581 = Equal?(x="config - write", y=w1273) -> (x = y?=w1282:bool)
            n582 = call <vilib>:"Q.Enqueue Task.vi"("Top of Q"=TRUE, "Task Name"="Read Limits", "Q In"=w1272) -> ()  [unwired: 7 in, 2 out]
            n583 = Unbundle By Name(w1297) -> ("Cfg.Dirs.Config"=w1296:path)
            n584 = Bundle By Name(cluster=T25 {"Devices"={"AudioOutName"="Line", "AudioInName"="HMD"}, "SweepParams"={"Duration"=2.0, "Amplitude"=1.0, "FreqStart"=20.0, "FreqEnd"=20000.0, "SampleRate"=44100.0, "StepCnt"=120, "FreqSpacing"=enum."Logarithmic", "Settling"={"Time"=0.0, "Cycles"=1.0}, "Measurement"={"Time"=0.001, "Cycles"=10.0}, "SyncPulseEn"=FALSE}, "DataFolder"=path "C:/MTE/Utah Core Audio Test/Data", "AvgLevelParams"={"Freq Start"=20.0, "Freq End"=20000.0}, "BlockedMicLim"={"CoveredMicAttn_dB"=500.0, "AvgLevelLL_dBFS"=12000.0, "AvgLevelUL_dBFS"=44100.0, "FreqRespLim"=path "C:/MTE/Utah Core Audio Test/Config/Microphone Test Freq Response Limits.ini", "THDLim"=path "C:/MTE/Utah Core Audio Test/Config/Microphone Test THD Limits.ini"}, "SpeakerCalFile"=path "C:/MTE/Utah Core Audio Test/Config/Microphone Test Speaker Calibration.ini", "Volume"=0.0} ("Params"), "Devices"="Sound Devices", "SweepParams"="Sine Sweep Params", "DataFolder"="Default Data Folder", "AvgLevelParams"="AvgLevelParams", "BlockedMicLim"="Limits", "SpeakerCalFile"="SpeakerCalFile", "Volume"="Play Volume") -> (w1268:T25)
            n585 = call "AudioTest.Config, Read_Write Microphone Test Setup.vi"("Read(F)/Write(T)"=w1282, "Params"=w1268, "Config Folder"=w1296) -> ("error out"=w1286:errorcluster, "Params"=w1292:T25)  [unwired: 7 in]
            n586 = Unbundle By Name(w1292) -> ("Devices"=w1291:T6, "SweepParams"=w1290:T7, "DataFolder"=w1289:path, "AvgLevelParams"=w1281:T5, "BlockedMicLim"=w1279:T4, "SpeakerCalFile"=w1276:path, "Volume"=w1274:dbl)
            n587 = call <vilib>:"File.Create Folder if Does Not Exist.vi"("Path"=w1289) -> ("error out"=w1287:errorcluster, "Dup Path"=w1288:path)  [unwired: 8 in, 1 out]
            n588 = local write "Sine Sweep Params"(w1290) -> ()
            n589 = local write "Sound Devices"(w1291) -> ()
            n590 = local write "SpeakerCalFile"(w1276) -> ()
            n591 = local write "AvgLevelParams"(w1281) -> ()
            n592 = local write "Default Data Folder"(w1288) -> ()
            n593 = local write "Play Volume"(w1274) -> ()
            n594 = local write "Limits"(w1279) -> ()
            n595 = Merge Errors(w1286, w1287) -> (w1285:errorcluster)
          }
          frame "Read Limits" {
            # "Inc code for LL"
            n596 = local read "Limits"() -> (w1304:T4)
            n597 = call <vilib>:"Q.Enqueue Task.vi"("Top of Q"=TRUE, "Task Name"="Plot Limits", "Q In"=w1301) -> ()  [unwired: 7 in, 2 out]
            n598 = Unbundle By Name(w1304) -> ("FreqRespLim"=w1303:path, "THDLim"=w1302:path)
            n599 = Bundle By Name(cluster=T22 {"Order"=0, "Name"="Freq Response", "X"=[], "Y"=[], "X Units"="dB", "Y Units"="Hz", "LimitType"=enum."None", "FailCode"=0, "FailDesc"="", "Ref Data Name"="", "Result Name"="", "0dB Level"=0.0, "Normalized"=FALSE} ("Plot Template"), "Name"="THD", "FailCode"=400) -> (w1318:T22)
            n600 = Bundle By Name(cluster=T22 {"Order"=0, "Name"="Freq Response", "X"=[], "Y"=[], "X Units"="dB", "Y Units"="Hz", "LimitType"=enum."None", "FailCode"=0, "FailDesc"="", "Ref Data Name"="", "Result Name"="", "0dB Level"=0.0, "Normalized"=FALSE} ("Plot Template"), "Name"="Frequency Response", "FailCode"=300) -> (w1324:T22)
            n601 = call "AudioTest.Read Limit File, Output to Plot Item.vi"("Plot Template"=w1318, "Limit File"=w1302) -> ("error out"=w1316:errorcluster, "UL"=w1307:T22, "LL"=w1306:T22)  [unwired: 7 in]
            n602 = call "AudioTest.Read Limit File, Output to Plot Item.vi"("Plot Template"=w1324, "Limit File"=w1303) -> ("error out"=w1317:errorcluster, "UL"=w1310:T22, "LL"=w1308:T22)  [unwired: 7 in]
            n603 = Unbundle By Name(w1308) -> ("FailCode"=w1314:i32)
            n604 = Unbundle By Name(w1306) -> ("FailCode"=w1311:i32)
            n605 = Increment(x=w1314) -> (x+1=w1313:i32)
            n606 = Bundle By Name(cluster=w1308, "FailCode"=w1313) -> (w1309:T22)
            n607 = Increment(x=w1311) -> (x+1=w1312:i32)
            n608 = Bundle By Name(cluster=w1306, "FailCode"=w1312) -> (w1305:T22)
            n609 = Bundle By Name(cluster=w1326, "FR Lim.LL"=w1309, "FR Lim.UL"=w1310, "THD Lim.LL"=w1305, "THD Lim.UL"=w1307) -> (w1327:T36)
            n610 = Merge Errors(w1317, w1316) -> (w1315:errorcluster)
          }
          frame "Plot Limits" {
            n611 = Unbundle By Name(w1343) -> ("FR Lim"=w1342:cluster{"LL":T22, "UL":T22}, "THD Lim"=w1329:cluster{"LL":T22, "UL":T22})
            n612 = local read "Right Freq Response"() -> (w1357:cluster{"frequency":dbl[], "magnitude":dbl[]}[])
            n613 = local read "Left Freq Response"() -> (w1350:cluster{"frequency":dbl[], "magnitude":dbl[]}[])
            n614 = local read "Left Mic THD"() -> (w1337:cluster{"X":dbl[], "Y":dbl[]}[])
            n615 = local read "Right Mic THD"() -> (w1334:cluster{"F":dbl[], "M":dbl[]}[])
            n616 = Unbundle By Name(w1342) -> ("UL.X"=w1360:dbl[], "UL.Y"=w1361:dbl[])
            n617 = Unbundle By Name(w1342) -> ("LL.X"=w1358:dbl[], "LL.Y"=w1359:dbl[])
            n618 = Unbundle By Name(w1342) -> ("UL.X"=w1347:dbl[], "UL.Y"=w1346:dbl[])
            n619 = Unbundle By Name(w1342) -> ("LL.X"=w1349:dbl[], "LL.Y"=w1348:dbl[])
            n620 = Unbundle By Name(w1329) -> ("UL.X"=w1340:dbl[], "UL.Y"=w1341:dbl[])
            n621 = Unbundle By Name(w1329) -> ("UL.X"=w1331:dbl[], "UL.Y"=w1330:dbl[])
            n622 = Bundle("X"=w1360, "Y"=w1361) -> (w1362:cluster{"X":dbl[], "Y":dbl[]})  [unwired: 1 in]
            n623 = Bundle("X"=w1358, "Y"=w1359) -> (w1363:cluster{"X":dbl[], "Y":dbl[]})  [unwired: 1 in]
            n624 = Bundle("X"=w1347, "Y"=w1346) -> (w1345:cluster{"X":dbl[], "Y":dbl[]})  [unwired: 1 in]
            n625 = Bundle("X"=w1349, "Y"=w1348) -> (w1344:cluster{"X":dbl[], "Y":dbl[]})  [unwired: 1 in]
            n626 = Index Array(array=w1357) -> (element #1=w1356:cluster{"frequency":dbl[], "magnitude":dbl[]}, element #2=w1355:cluster{"frequency":dbl[], "magnitude":dbl[]})  [unwired: 2 in]
            n627 = Index Array(array=w1350) -> (element #1=w1351:cluster{"frequency":dbl[], "magnitude":dbl[]}, element #2=w1352:cluster{"frequency":dbl[], "magnitude":dbl[]})  [unwired: 2 in]
            n628 = Bundle("X"=w1340, "Y"=w1341) -> (w1339:cluster{"X":dbl[], "Y":dbl[]})  [unwired: 1 in]
            n629 = Index Array(array=w1337) -> (element=w1336:cluster{"X":dbl[], "Y":dbl[]})  [unwired: 1 in]
            n630 = Bundle("X"=w1331, "Y"=w1330) -> (w1332:cluster{"X":dbl[], "Y":dbl[]})  [unwired: 1 in]
            n631 = Index Array(array=w1334) -> (element=w1335:cluster{"F":dbl[], "M":dbl[]})  [unwired: 1 in]
            n632 = Build Array(w1356, w1355, w1363, w1362) -> (w1354:cluster{"X":dbl[], "Y":dbl[]}[])
            n633 = Build Array(w1336, w1339) -> (w1338:cluster{"X":dbl[], "Y":dbl[]}[])
            n634 = Build Array(w1335, w1332) -> (w1333:cluster{"X":dbl[], "Y":dbl[]}[])
            n635 = Build Array(w1351, w1352, w1344, w1345) -> (w1353:cluster{"X":dbl[], "Y":dbl[]}[])
            n636 = local write "Right Freq Response"(w1354) -> ()
            n637 = local write "Left Freq Response"(w1353) -> ()
            n638 = local write "Left Mic THD"(w1338) -> ()
            n639 = local write "Right Mic THD"(w1333) -> ()
          }
          frame "Save Wav Files" {
            n640 = local read "Save Wav Files"() -> (w1365:bool)
            n641 = Bundle By Name(cluster=w1366, "SavWav"=w1365) -> (w1367:T36)
          }
          frame "Create_UUTFolder" {
            n642 = Unbundle By Name(w1379) -> ("Dirs.Temp Data"=w1377:path)
            n643 = local read "Start Time"() -> (w1375:timestamp)
            n644 = local read "SN"() -> (w1376:string)
            n645 = Unbundle By Name(w1372) -> ("Cfg.Parent Q"=w1371:refnum<queue>)
            n646 = call "File.Create UUT Dir.vi"("Start Time"=w1375, "SN"=w1376, "Local Data Dir"=w1377) -> ("error out"=w1373:errorcluster, "UUTDir"=w1370:path, "SN_Time"=w1374:string)  [unwired: 6 in]
            n647 = Not A Number/Path/Refnum?(number/path/refnum=w1371) -> (NaN/Path/Refnum?=w1369:bool)
            n648 = case shown="False" w1369 {
              tunnel: w1371 -> [w1385 _]
              tunnel: w1370 -> [w1381 _]
              frame False {
                n649 = Path To String(path=w1381) -> (string=w1384:string)
                n650 = Build Array("UUTDir", w1384) -> (w1383:string[])
                n651 = Build Array(w1383) -> (w1380:string[][])
                n652 = call "TestExec.Set Seq Variable.vi"("Variables"=w1380, "Q In"=w1385) -> ()  [unwired: 9 in, 1 out]
              }
              frame True {
              }
            }
            n653 = local write "UUT Dir"(w1370) -> ()
            n654 = Bundle By Name(cluster=w1379, "Dirs.UUTDir"=w1370, "SN_Time"=w1374) -> (w1378:T36)
          }
          frame "Set TimeOut" {
            n655 = Variant To Data(type=0.0, Variant=w1394) -> (data=w1388:dbl, error out=w1393:errorcluster)  [unwired: 1 in]
            n656 = In Range and Coerce(upper limit=900.0, x=w1388, lower limit=1.0) -> (coerced(x)=w1389:dbl)  [unwired: 1 out]
            n657 = local write "Timeout(s)"(w1389) -> ()
            n658 = Bundle By Name(cluster=w1391, "Timeout(s)"=w1389) -> (w1390:T36)
          }
          frame "Report SW Ver" {
          }
          frame "TCP-IP" {
            n659 = Variant To Data(type=FALSE, Variant=w1409) -> (data=w1400:bool)  [unwired: 1 in, 1 out]
            n660 = Bundle By Name(cluster=w1399, "Cfg.Is Child?"=w1400) -> (w1404:T13)
            n661 = case shown="True" w1400 {
              tunnel: w1407 -> [_ w1415]
              tunnel: w1398 -> [_ w1411]
              frame False {
              }
              frame True {
                # "When Parent connects, Send SW Version and SW Framework Version"
                n662 = Unbundle By Name(w1411) -> ("StaVer"=w1410:i32)
                n663 = call <vilib>:"Q.Enqueue Task.vi"("Task Name"="Report SW Ver", "Q In"=w1415) -> ("Q Out"=w1414:refnum<queue>)  [unwired: 8 in, 1 out]
                n664 = To Variant(anything=w1410) -> (Variant=w1412:variant)
                n665 = call <vilib>:"Q.Enqueue Task.vi"("Data1"=w1412, "Task Name"="Sta Notify Ver", "Q In"=w1414) -> ()  [unwired: 7 in, 2 out]
              }
            }
            n666 = Unbundle By Name(w1404) -> ("Log"=w1406:refnum<class "Event Notification.lvclass">)
            n667 = Select(t="TCP-IP Connected", s=w1400, f="TCP-IP Disconnected") -> (s? t:f=w1401:string)
            n668 = call <vilib>:"Event Notification.Status Message.vi"("Level"=Event_Log.Log_Level."Verbose", "Message"=w1401, "Event Notification in"=w1406) -> ()  [unwired: 9 in]
          }
          frame "Abort", "Test Abort" {
            n669 = call <vilib>:"Scheduler.Clear-Reset.vi"("Q In"=w1424) -> ("error out"=w1426:errorcluster, "Q Out"=w1425:refnum<queue>)  [unwired: 9 in]
            n670 = Flush Queue(queue=w1425, error in (no error)=w1426) -> (queue out=w1423:refnum<queue>)  [unwired: 2 out]
            n671 = Unbundle By Name(w1421) -> ("Log"=w1420:refnum<class "Event Notification.lvclass">)
            n672 = call <vilib>:"Q.Enqueue Task.vi"("Task Name"="Test End", "Q In"=w1423) -> ()  [unwired: 8 in, 2 out]
            n673 = call <vilib>:"Event Notification.Status Message.vi"("Level"=Event_Log.Log_Level."Verbose", "Message"="Test Aborted by Operator", "Event Notification in"=w1420) -> ()  [unwired: 9 in]
            n674 = invoke on="Play Tone" class="Bool (strict)" method="Reinit To Default"() -> ()  [unwired: 3 in, 3 out]
            n675 = for {
              N: 5 -> [_]
              n676 = call "Abort.Send Abort or Done Notificaiton.vi"("Abort(T)/Done(F)"=TRUE) -> ()  [unwired: 10 in, 1 out]
              n677 = Wait (ms)(milliseconds to wait=u32 10) -> ()  [unwired: 1 out]
            }
          }
          frame "Test Data Dirs" {
            n678 = Variant To Data(type=T26[] [{"Name"="", "Path"=path ""}], Variant=w1435) -> (data=w1434:T26[])  [unwired: 1 in, 1 out]
            n679 = Unbundle By Name(w1431) -> ("Dirs"=w1433:T35)
            n680 = for {
              tunnel: w1434 -> [w1440] mode=indexing
              shift-right: [w1441] -> w1432
              shift-left: w1433 -> [w1442]
              n681 = Unbundle By Name(w1440) -> ("Name"=w1439:string, "Path"=w1438:path)
              n682 = case shown="\"DataSumArchiveDir\"" w1439 {
                tunnel: w1442 -> [w1443 w1447 w1452]
                tunnel: [w1443 w1446 w1451] -> w1441
                tunnel: w1438 -> [_ w1445 w1450]
                tunnel: [_ _ w1448] -> _
                frame Default {
                }
                frame "DataArchiveDir" {
                  n683 = call <vilib>:"File.Create Folder if Does Not Exist.vi"("Path"=w1445) -> ("Dup Path"=w1444:path)  [unwired: 8 in, 2 out]
                  n684 = Bundle By Name(cluster=w1447, "Archive"=w1444) -> (w1446:T35)
                }
                frame "DataSumArchiveDir" {
                  n685 = call <vilib>:"File.Create Folder if Does Not Exist.vi"("Path"=w1450) -> ("error out"=w1448:errorcluster, "Dup Path"=w1449:path)  [unwired: 8 in, 1 out]
                  n686 = Bundle By Name(cluster=w1452, "ArchiveSum"=w1449) -> (w1451:T35)
                }
              }
            }
            n687 = Bundle By Name(cluster=w1431, "Dirs"=w1432) -> (w1430:T36)
          }
          frame "Test End" {
            w1463 = FALSE
            n688 = To Variant(anything=FALSE) -> (Variant=w1467:variant)
            n689 = call <vilib>:"Q.Enqueue App.vi"("Top of Q"=TRUE, "Data1"=w1467, "Task Name"="Lock Test Controls", "Q In"=w1464) -> ()  [unwired: 6 in, 2 out]
            n690 = property on="Test Reset" class="Bool"("DisabledEnum"=T19."Enabled" ("Disabled")) -> ()  [unwired: 2 in, 2 out]
            n691 = property on="Abort" class="Bool"("DisabledEnum"=T19."Disabled and Grayed Out" ("Disabled")) -> ()  [unwired: 2 in, 2 out]
            n692 = property on="Test Running" class="Bool (strict)"("Blinking"=w1463, "Value"=w1463) -> ()  [unwired: 2 in, 2 out]
            n693 = local read "Start Time"() -> (w1461:timestamp)
            n694 = Get Date/Time In Seconds() -> (seconds since 1Jan1904=w1462:timestamp)
            n695 = Bundle By Name(cluster=w1453, "Remote Test"=FALSE) -> (w1455:T36)
            n696 = Subtract(x=w1462, y=w1461) -> (x-y=→"Duration(s)":dbl)
          }
          frame "Test Mode" {
            # "TE will send the test mode at the start of a test.\nUse this to make decisions and/or to store with data.\nIt may not apply to this station module."
            n697 = Variant To Data(type="", Variant=w1474) -> (data=w1468:string)  [unwired: 1 in, 1 out]
            n698 = Unbundle By Name(w1472) -> ("FunctData"=w1470:refnum<class "FunctDataMgr.lvclass">)
            n699 = local write "Mode"(w1468) -> ()
            n700 = call "FunctDataMgr.Update Test Mode.vi"("Mode"=w1468, "FunctDataMgr in"=w1470) -> ("FunctDataMgr out"=w1469:refnum<class "FunctDataMgr.lvclass">)  [unwired: 8 in, 1 out]
            n701 = Bundle By Name(cluster=w1472, "FunctData"=w1469) -> (w1471:T36)
          }
          frame "Test Reset" {
            w1479 = u32 13816530
            n702 = call "Error.Clear.vi"("Q In"=w1488) -> ("Q Out"=w1480:refnum<queue>)  [unwired: 9 in, 1 out]
            n703 = call <vilib>:"Q.Enqueue Task.vi"("Task Name"="Clear Graphs", "Q In"=w1480) -> ("Q Out"=w1481:refnum<queue>)  [unwired: 8 in, 1 out]
            n704 = invoke on="Play Tone" class="Bool (strict)" method="Reinit To Default"() -> ()  [unwired: 3 in, 3 out]
            n705 = call <vilib>:"Q.Enqueue Task.vi"("Task Name"="Clear Raw Data", "Q In"=w1481) -> ()  [unwired: 8 in, 2 out]
            n706 = Bundle By Name(cluster=w1477, "Rslt.Meas"=T17[] []) -> (w1478:T36)
            n707 = property on="L AvgMagUnCov" class="DigNum (strict)"("NumText.BGColor"=w1479) -> ()  [unwired: 2 in, 2 out]
            n708 = property on="R AvgMagUnCov" class="DigNum (strict)"("NumText.BGColor"=w1479) -> ()  [unwired: 2 in, 2 out]
            n709 = property on="R AvgMag Delta" class="DigNum (strict)"("NumText.BGColor"=w1479) -> ()  [unwired: 2 in, 2 out]
            n710 = property on="L AvgMag Delta" class="DigNum (strict)"("NumText.BGColor"=w1479) -> ()  [unwired: 2 in, 2 out]
            n711 = local write "LThdColor"(w1479) -> ()
            n712 = local write "RtFRColor"(w1479) -> ()
            n713 = local write "RtThdColor"(w1479) -> ()
            n714 = local write "LFRColor"(w1479) -> ()
            n715 = Unbundle By Name(w1478) -> ("FunctData"=w1486:refnum<class "FunctDataMgr.lvclass">)
            n716 = call "FunctDataMgr.Reset Data.vi"("FunctDataMgr in"=w1486) -> ("FunctDataMgr out"=w1487:refnum<class "FunctDataMgr.lvclass">)  [unwired: 9 in, 1 out]
            n717 = Bundle By Name(cluster=w1478, "FunctData"=w1487) -> (w1485:T36)
            n718 = invoke on="Duration(s)" class="DigNum (strict)" method="Reinit To Default"() -> ()  [unwired: 3 in, 3 out]
            n719 = invoke on="Enumerated" class="Bool (strict)" method="Reinit To Default"() -> ()  [unwired: 3 in, 3 out]
            n720 = property on="Status" class="Str"("Text.BGColor"=u32 13816530) -> ()  [unwired: 2 in, 2 out]
            n721 = local write "Status"("Idle") -> ()
          }
          frame "Test Start" {
            n722 = while {
              tunnel: w1495 -> [w1501]
              tunnel: w1494 -> [w1500]
              shift-right: [w1504] -> w1493
              shift-left: w1497 -> [w1506]
              shift-right: [w1503] -> w1492
              shift-left: w1496 -> [w1505]
              tunnel: [w1498] -> w1491
              i -> [w1502]
              stop <- w1499 stop-if-true
              n723 = case shown="1" w1502 {
                tunnel: w1506 -> [w1520 w1530 w1546 w1562]
                tunnel: w1505 -> [w1510 w1529 w1542 w1561]
                tunnel: [w1520 w1530 w1546 w1562] -> w1504
                tunnel: [w1512 w1529 w1542 w1561] -> w1503
                tunnel: w1501 -> [_ _ w1547 _]
                tunnel: w1500 -> [w1513 _ _ _]
                tunnel: [_ _ _ TRUE] -> w1499
                tunnel: [errorcluster {"status"=FALSE, "code"=0, "source"=""} ("error constant") _ _ _] -> w1498
                frame 0 {
                  # "Record Start Info"
                  n724 = Variant To Data(type=T27 {"Test Name"="", "Start Time"=timestamp(0 s since 1904-01-01), "UUT SN"=""} ("Test Start Info"), Variant=w1513) -> (data=w1519:T27, error out=w1517:errorcluster)  [unwired: 1 in]
                  n725 = case shown="No Error" w1517 {
                    tunnel: w1519 -> [w1525 _]
                    tunnel: [w1524 "Local" ("Test Name")] -> w1518
                    tunnel: [w1523 w1526] -> w1508
                    tunnel: [w1522 w1527] -> w1509
                    tunnel: [TRUE _] -> w1511
                    frame No Error {
                      # "Test launched from TE"
                      n726 = Unbundle By Name(w1525) -> ("Test Name"=w1524:string, "UUT SN"=w1522:string, "Start Time"=w1523:timestamp)
                      n727 = local write "Start Time"(w1523) -> ()
                      n728 = local write "SN"(w1522) -> ()
                    }
                    frame Error {
                      # "Test initiated locally"
                      n729 = local read "Start Time"() -> (w1526:timestamp)
                      n730 = local read "SN"() -> (w1527:string)
                    }
                  }
                  n731 = Unbundle By Name(w1510) -> ("FunctData"=w1516:refnum<class "FunctDataMgr.lvclass">)
                  n732 = call "FunctDataMgr.Test Start.vi"("Reset Data"=w1511, "StartTime"=w1508, "SN"=w1509, "Sequence"=w1518, "FunctDataMgr in"=w1516) -> ("FunctDataMgr out"=w1515:refnum<class "FunctDataMgr.lvclass">)  [unwired: 5 in, 1 out]
                  n733 = Bundle By Name(cluster=w1510, "FunctData"=w1515, "Remote Test"=w1511) -> (w1512:T36)
                }
                frame 1 {
                  w1537 = TRUE
                  # "Init Controls"
                  n734 = property on="Test Reset" class="Bool"("DisabledEnum"=T19."Disabled and Grayed Out" ("Disabled")) -> ()  [unwired: 2 in, 2 out]
                  n735 = property on="Abort" class="Bool"("DisabledEnum"=T19."Enabled" ("Disabled")) -> ()  [unwired: 2 in, 2 out]
                  n736 = Unbundle By Name(w1530) -> ("Log"=w1536:refnum<class "Event Notification.lvclass">)
                  n737 = property on="Test Running" class="Bool (strict)"("Blinking"=w1537) -> ()  [unwired: 2 in, 2 out]
                  n738 = call <vilib>:"Event Notification.Status Message with Error In.vi"("Display"=TRUE, "Log"=TRUE, "Level"=Event_Log.Log_Level."Verbose", "Type"=Event_Log.Notification_Type."Normal", "Message"="Test Running", "Event Notification in"=w1536) -> ()  [unwired: 6 in]
                  "Test Running" <- w1537
                }
                frame 2 {
                  # "Enqueue Tasks"
                  n739 = To Variant(anything=TRUE) -> (Variant=w1551:variant)
                  n740 = Unbundle By Name(w1542) -> ("Remote Test"=w1541:bool)
                  n741 = local read "UUT Dir"() -> (w1544:path)
                  n742 = call <vilib>:"Q.Enqueue App.vi"("Top of Q"=TRUE, "Data1"=w1551, "Task Name"="Lock Test Controls", "Q In"=w1547) -> ("Q Out"=w1545:refnum<queue>)  [unwired: 6 in, 1 out]
                  n743 = Not A Number/Path/Refnum?(number/path/refnum=w1544) -> (NaN/Path/Refnum?=w1543:bool)
                  n744 = Or(x=w1541, y=w1543) -> ()  [unwired: 1 out]
                  n745 = case shown="True" FALSE {
                    tunnel: w1545 -> [_ w1554]
                    frame False {
                    }
                    frame True {
                      n746 = call <vilib>:"Q.Enqueue Task.vi"("Top of Q"=TRUE, "Task Name"="Init UUT Folder", "Q In"=w1554) -> ()  [unwired: 7 in, 2 out]
                    }
                  }
                  n747 = Unbundle By Name(w1546) -> ("Child Modules"=w1552:cluster{"Name":string, "vi ref":refnum<vi>}[])
                  n748 = for {
                    tunnel: w1552 -> [w1557] mode=indexing
                    n749 = Unbundle By Name(w1557) -> ("Name"=w1558:string)
                    n750 = call <vilib>:"Q.Enqueue Task.vi"("Top of Q"=TRUE, "Q Name"=w1558, "Task Name"="Test Start") -> ()  [unwired: 7 in, 2 out]
                  }
                }
                frame Default {
                  # "Done"
                }
              }
            }
          }
          frame "Test Attr Data" {
            n751 = Variant To Data(type=T29[] [] ("Data.Attr"), Variant=w1568) -> (data=w1567:T29[])  [unwired: 1 in, 1 out]
            n752 = Unbundle By Name(w1564) -> ("FunctData"=w1563:refnum<class "FunctDataMgr.lvclass">)
            n753 = call "FunctDataMgr.Update Attribute Data.vi"("Data.Attr"=w1567, "FunctDataMgr in"=w1563) -> ("FunctDataMgr out"=w1565:refnum<class "FunctDataMgr.lvclass">)  [unwired: 8 in, 1 out]
            n754 = Bundle By Name(cluster=w1564, "FunctData"=w1565) -> (w1566:T36)
          }
          frame "Test Num Data" {
            n755 = Variant To Data(type=T30[] [] ("data"), Variant=w1577) -> (data=w1576:T30[])  [unwired: 1 in, 1 out]
            n756 = Unbundle By Name(w1573) -> ("FunctData"=w1572:refnum<class "FunctDataMgr.lvclass">)
            n757 = call "FunctDataMgr.Update Numeric Data.vi"("Data.Num"=w1576, "FunctDataMgr in"=w1572) -> ("FunctDataMgr out"=w1574:refnum<class "FunctDataMgr.lvclass">)  [unwired: 8 in, 1 out]
            n758 = Bundle By Name(cluster=w1573, "FunctData"=w1574) -> (w1575:T36)
          }
          frame "Set Config" {
            n759 = Unbundle By Name(w1581) -> ("AppData"=w1582:refnum<class "Class.AppData.lvclass">)
            n760 = call <vilib>:"ClassAppData.Load_Merge Data.vi"("Data In"=w1583, "Class - App Data in"=w1582) -> ("Class - App Data out"=w1579:refnum<class "Class.AppData.lvclass">)  [unwired: 8 in, 1 out]
            n761 = Bundle By Name(cluster=w1581, "AppData"=w1579) -> (w1580:T13)
          }
          frame "Update Results" {
            n762 = Unbundle By Name(w1586) -> ("FunctData"=w1585:refnum<class "FunctDataMgr.lvclass">)
            n763 = call "FunctDataMgr.Update Result Table Value.vi"("FunctDataMgr in"=w1585) -> ()  [unwired: 9 in, 2 out]
          }
          frame "Test Status" {
            w1593 = T33 {"State"=enum."Passing", "Code"=0, "Description"=""}  # ResultState
            n764 = Variant To Data(type=w1593, Variant=w1595) -> (data=w1588:T33)  [unwired: 1 in, 1 out]
            n765 = Unbundle By Name(w1589) -> ("FunctData"=w1591:refnum<class "FunctDataMgr.lvclass">)
            n766 = call "FunctDataMgr.Update Result State.vi"("Result Info"=w1588, "FunctDataMgr in"=w1591) -> ("FunctDataMgr out"=w1592:refnum<class "FunctDataMgr.lvclass">)  [unwired: 8 in, 1 out]
            n767 = Bundle By Name(cluster=w1589, "FunctData"=w1592) -> (w1590:T36)
            n768 = Bundle By Name(cluster=w1590, "ResultState"=w1588) -> (w1594:T36)
          }
          frame "Update SN" {
            n769 = Variant To Data(type="", Variant=w1606) -> (data=w1601:string)  [unwired: 1 in, 1 out]
            n770 = Unbundle By Name(w1605) -> ("FunctData"=w1609:refnum<class "FunctDataMgr.lvclass">)
            n771 = Unbundle By Name(w1605) -> ("Dirs.UUTDir"=w1604:path)
            n772 = local write "SN"(w1601) -> ()
            n773 = call "FunctDataMgr.Update SN.vi"("SN"=w1601, "FunctDataMgr in"=w1609) -> ("FunctDataMgr out"=w1608:refnum<class "FunctDataMgr.lvclass">)  [unwired: 8 in, 1 out]
            n774 = call <vilib>:"File.Check if File or Folder Exists.vi"("Path"=w1604) -> ("Exists"=w1603:bool, "Dup Path"=w1602:path)  [unwired: 6 in, 3 out]
            n775 = Bundle By Name(cluster=w1605, "FunctData"=w1608) -> (w1599:T36)
            n776 = case shown="True" w1603 {
              tunnel: w1602 -> [_ w1616]
              tunnel: w1601 -> [_ w1625]
              tunnel: [_ w1623] -> w1600
              tunnel: w1599 -> [w1610 w1622]
              tunnel: [w1610 w1621] -> w1598
              tunnel: w1597 -> [_ w1612]
              frame False {
              }
              frame True {
                # "Replace SN"
                n777 = Strip Path(path=w1616) -> (stripped path=w1615:path, name=w1627:string)
                n778 = Match Pattern(string=w1627, regular expression="_") -> (match substring=w1617:string, after substring=w1618:string)  [unwired: 1 in, 2 out]
                n779 = Concatenate Strings(w1625, w1617, w1618) -> (w1624:string)
                n780 = Build Path(base path=w1615, name or relative path=w1624) -> (appended path=w1620:path)
                n781 = Not Equal?(x=w1616, y=w1620) -> (x != y?=w1619:bool)
                n782 = Unbundle By Name(w1612) -> ("Cfg.Parent Q"=w1614:refnum<queue>)
                n783 = case shown="True" w1619 {
                  tunnel: [_ w1638] -> w1623
                  tunnel: [w1634 w1637] -> w1611
                  tunnel: w1616 -> [w1634 w1636]
                  tunnel: w1620 -> [_ w1635]
                  frame False {
                  }
                  frame True {
                    n784 = Move(source path=w1636, 10:w1635) -> (error out=w1638:errorcluster, 3:w1637:path)  [unwired: 3 in, 1 out]
                  }
                }
                n785 = Not A Number/Path/Refnum?(number/path/refnum=w1614) -> (NaN/Path/Refnum?=w1613:bool)
                n786 = local write "UUT Dir"(w1611) -> ()
                n787 = case shown="False" w1613 {
                  tunnel: w1614 -> [w1633 _]
                  tunnel: w1611 -> [w1629 _]
                  frame False {
                    n788 = Path To String(path=w1629) -> (string=w1632:string)
                    n789 = Build Array("UUTDir", w1632) -> (w1631:string[])
                    n790 = Build Array(w1631) -> (w1628:string[][])
                    n791 = call "TestExec.Set Seq Variable.vi"("Variables"=w1628, "Q In"=w1633) -> ()  [unwired: 9 in, 1 out]
                  }
                  frame True {
                  }
                }
                n792 = Bundle By Name(cluster=w1622, "Dirs.UUTDir"=w1611) -> (w1621:T36)
              }
            }
          }
          frame "Update UUT Folder" {
            n793 = Bundle By Name(cluster=w1641, "Dirs.UUTDir"="UUT Dir") -> (w1640:T36)
          }
          frame "Warning" {
            n794 = Variant To Data(type=errorcluster {"status"=FALSE, "code"=0, "source"=""} ("error constant"), Variant=w1645) -> (data=w1646:errorcluster)  [unwired: 1 in, 1 out]
            n795 = Unbundle By Name(w1644) -> ("Cfg.Is Child?"=w1653:bool, "Cfg.Parent Q"=w1652:refnum<queue>)
            n796 = case shown="True" w1653 {
              tunnel: w1652 -> [_ w1656]
              tunnel: w1646 -> [_ w1657]
              tunnel: [_ w1658] -> _
              frame False {
              }
              frame True {
                n797 = call "TestExec.Health Status, Set Error_Warning.vi"("error in"=w1657, "Health State Cmd"=TestExec.Health_State_Command."Set Warning", "Q In"=w1656) -> ("error out"=w1658:errorcluster)  [unwired: 8 in]
              }
            }
            n798 = Unbundle By Name(w1646) -> ("source"=w1649:string)
            n799 = Concatenate Strings("WARNING: ", w1649) -> (w1650:string)
            n800 = Bundle By Name(cluster=w1646, "status"=FALSE, "source"=w1650) -> (w1643:errorcluster)
            n801 = local write "Error"(w1643) -> ()
          }
          frame "Play Tone" {
            w1663 = T40 1 items=["Finite Samples", "Continuous Samples"] ("sample mode")
            n802 = local read "Output Device"() -> (w1659:i32)
            n803 = call <vilib>:"Sound Output Configure.vi"("number of samples/ch"=5000 ("Number of Samples/ch"), "sample mode"=w1663, "sound format"=T21 {"sample rate (S/s)"=44100.0, "number of channels"=2, "bits per sample"=16} ("Sound Format"), "device ID"=w1659) -> ("error out"=w1667:errorcluster, "task ID"=w1666:T41)  [unwired: 6 in]
            n804 = while {
              tunnel: w1666 -> [w1679]
              tunnel: [w1683] -> w1664
              tunnel: w1667 -> [w1681]
              tunnel: [w1678] -> w1665
              stop <- w1682 stop-if-true
              # "Generate Sound"
              n805 = local read "Play Volume"() -> (w1673:dbl)
              n806 = call-poly <vilib>:"Sound Output Set Volume.vi"("error in (no error)"=w1681, "volume"=w1673, "task ID"=w1679) -> ("error out"=w1676:errorcluster, "task ID out"=w1680:T41)  [unwired: 7 in]
              n807 = call "Simulate Signal"("Frequency"="Tone Freq", "error in (no error)"=w1676) -> ("Sine"=w1674:dynamicdata, "error out"=w1675:errorcluster)  [unwired: 12 in]
              n808 = local read "Play Tone"() -> (w1671:bool)
              n809 = call "Convert from Dynamic Data"("Dynamic Data Type"=w1674) -> ("Waveform"=w1677:waveform(dbl))  [unwired: 3 in]
              n810 = call-poly <vilib>:"Sound Output Write.vi"("error in (no error)"=w1675, "data"=w1677, "task ID"=w1680) -> ("error out"=w1678:errorcluster, "task ID out"=w1683:T41)  [unwired: 7 in]
              n811 = Not(x=w1671) -> (.not. x?=w1670:bool)
              n812 = Or(x=w1678, y=w1670) -> (x .or. y?=w1682:bool)
            }
            n813 = call <vilib>:"Sound Output Clear.vi"("error in (no error)"=w1665, "task ID"=w1664) -> ("error out"=w1660:errorcluster)  [unwired: 9 in]
          }
          frame Default {
            # "Handle default function tasks"
            n814 = Unbundle By Name(w1687) -> ("FunctData"=w1690:refnum<class "FunctDataMgr.lvclass">)
            n815 = call "FunctDataMgr.Default Tasks.vi"("Data In"=w1689, "Task In"=w1684, "FunctDataMgr in"=w1690) -> ("Not Fwd Data"=w1685:bool, "FunctDataMgr out"=w1688:refnum<class "FunctDataMgr.lvclass">)  [unwired: 6 in, 1 out]
            n816 = case shown="True" w1685 {
              tunnel: w1695 -> [_ w1708]
              tunnel: w1694 -> [w1697 w1707]
              tunnel: [w1697 w1706] -> w1693
              tunnel: w1692 -> [w1698 w1705]
              tunnel: [w1698 w1704] -> w1691
              tunnel: w1689 -> [_ w1703]
              tunnel: w1688 -> [w1696 _]
              tunnel: w1687 -> [w1700 w1702]
              tunnel: [w1699 w1702] -> w1686
              tunnel: w1684 -> [_ w1701]
              frame False {
                # "Task Handled"
                n817 = Bundle By Name(cluster=w1700, "FunctData"=w1696) -> (w1699:T36)
              }
              frame True {
                # "Handle default module tasks"
                n818 = call <vilib>:"Module.Default Tasks.vi"("Sys"=w1705, "error in"=w1707, "Data2"=w1708, "Data1"=w1703, "Sub"=w1701) -> ("error out"=w1706:errorcluster, "Sys Out"=w1704:T13)  [unwired: 5 in]
              }
            }
          }
        }
      }
      frame "Function" {
        n819 = while {
          shift-right: [w1730] -> w1716
          shift-left: w1718 -> [w1731]
          shift-right: [w1728] -> w1715
          shift-left: w1717 -> [w1729]
          shift-right: [w1726] -> _
          shift-left: _ -> [w1727]
          shift-right: [w1723] -> w1713
          shift-left: w1714 -> [w1724]
          tunnel: w1712 -> [w1722]
          tunnel: w1711 -> [w1721]
          tunnel: w1710 -> [w1720]
          tunnel: w1709 -> [w1719]
          i -> [w1732]
          stop <- w1725 stop-if-true
          n820 = case shown="1" w1732 {
            tunnel: w1731 -> [w1737 w1756 w1904]
            tunnel: [w1737 w1754 w1904] -> w1730
            tunnel: w1729 -> [w1745 w1755 w1902]
            tunnel: [w1744 w1753 w1901] -> w1728
            tunnel: w1727 -> [_ _ w1898]
            tunnel: [FALSE w1748 _] -> w1726
            tunnel: [_ _ TRUE] -> w1725
            tunnel: w1724 -> [_ w1747 w1899]
            tunnel: [_ w1751 w1900] -> w1723
            tunnel: w1722 -> [w1736 w1752 _]
            tunnel: w1721 -> [_ w1750 w1897]
            tunnel: w1720 -> [_ w1749 _]
            tunnel: w1719 -> [w1742 _ _]
            frame 0 {
              # "Default to Immediate Return"
              # "Init"
              n821 = Unbundle By Name(w1745) -> ("FunctData"=w1746:refnum<class "FunctDataMgr.lvclass">)
              n822 = call "FunctDataMgr.Function Initialize.vi"("RTN Info"=w1742, "Name"=w1736, "FunctDataMgr in"=w1746) -> ("FunctDataMgr out"=w1743:refnum<class "FunctDataMgr.lvclass">)  [unwired: 7 in, 1 out]
              n823 = Bundle By Name(cluster=w1745, "FunctData"=w1743) -> (w1744:T36)
              n824 = Format Into String(format string="Performing: %s", w1736) -> (resulting string=w1738:string)  [unwired: 2 in, 1 out]
              n825 = Unbundle By Name(w1737) -> ("Log"=w1740:refnum<class "Event Notification.lvclass">)
              n826 = call <vilib>:"Event Notification.Status Message.vi"("Display"=TRUE ("Log"), "Log"=FALSE, "Level"=Event_Log.Log_Level."Verbose", "Message"=w1738, "Event Notification in"=w1740) -> ()  [unwired: 7 in]
            }
            frame 1 {
              # "Execute"
              n827 = case shown="\"Archive_Results\"" w1752 {
                selector: w1752 -> [_ _ _ _ _ w1863]
                tunnel: w1756 -> [w1770 w1778 w1800 w1826 w1838 w1858]
                tunnel: w1755 -> [w1761 w1786 w1811 w1825 w1836 w1866]
                tunnel: [w1770 w1778 w1800 w1826 w1838 w1858] -> w1754
                tunnel: [w1758 w1785 w1810 w1825 w1836 w1867] -> w1753
                tunnel: [_ _ _ w1815 w1834 w1865] -> w1751
                tunnel: w1750 -> [_ _ w1796 _ _ w1857]
                tunnel: w1749 -> [_ w1772 w1795 w1819 w1835 w1856]
                tunnel: [_ _ _ _ _ FALSE] -> w1748
                tunnel: w1747 -> [_ _ _ _ _ _]
                frame "Create_UUTFolder" {
                  n828 = Unbundle By Name(w1761) -> ("Dirs.Temp Data"=w1764:path)
                  n829 = local read "SN"() -> (w1763:string)
                  n830 = local read "Start Time"() -> (w1762:timestamp)
                  n831 = call "File.Create UUT Dir.vi"("Start Time"=w1762, "SN"=w1763, "Local Data Dir"=w1764) -> ("error out"=w1757:errorcluster, "UUTDir"=w1759:path)  [unwired: 6 in, 1 out]
                  n832 = local write "UUT Dir"(w1759) -> ()
                  n833 = Path To String(path=w1759) -> (string=w1767:string)
                  n834 = Build Array("UUTDir", w1767) -> (w1765:string[])
                  n835 = Unbundle By Name(w1761) -> ("FunctData"=w1769:refnum<class "FunctDataMgr.lvclass">)
                  n836 = Build Array(w1765) -> (w1760:string[][])
                  n837 = call "FunctDataMgr.Function Add RTN Data.vi"("Vars"=w1760, "Error In"=w1757, "FunctDataMgr in"=w1769) -> ("FunctDataMgr out"=w1768:refnum<class "FunctDataMgr.lvclass">)  [unwired: 8 in]
                  n838 = Bundle By Name(cluster=w1761, "FunctData"=w1768, "Dirs.UUTDir"=w1759) -> (w1758:T36)
                }
                frame "GetUUTSN" {
                  n839 = Variant To Data(type=string[] [], Variant=w1772) -> (data=w1773:string[], error out=w1774:errorcluster)  [unwired: 1 in]
                  n840 = Unbundle By Name(w1778) -> ("Child Modules"=w1784:cluster{"Name":string, "vi ref":refnum<vi>}[])
                  n841 = case shown="No Error" w1774 {
                    tunnel: w1773 -> [w1790 _]
                    tunnel: [w1789 _] -> w1771
                    frame No Error {
                      n842 = Index Array(array=w1790) -> (element=w1789:string)  [unwired: 1 in]
                    }
                    frame Error {
                    }
                  }
                  n843 = Index Array(array=w1784) -> (element=w1783:cluster{"Name":string, "vi ref":refnum<vi>})  [unwired: 1 in]
                  n844 = Unbundle By Name(w1778) -> ("Cfg.Parent Q"=w1782:refnum<queue>, "Cfg.Is Child?"=w1781:bool)
                  n845 = Unbundle By Name(w1783) -> ("Name"=w1777:string)
                  n846 = call "TestExec.HMD, Pull SN from UUT.vi"("VarName"=w1771, "ParentQ"=w1782, "HMD Q Name"=w1777, "IsChild"=w1781) -> ("error out"=w1776:errorcluster, "Vars"=w1779:string[][], "SN"=w1780:string)  [unwired: 5 in]
                  n847 = case shown="No Error" w1776 {
                    tunnel: w1780 -> [w1791 _]
                    frame No Error {
                      n848 = local write "SN"(w1791) -> ()
                    }
                    frame Error {
                    }
                  }
                  n849 = Unbundle By Name(w1786) -> ("FunctData"=w1788:refnum<class "FunctDataMgr.lvclass">)
                  n850 = call "FunctDataMgr.Function Add RTN Data.vi"("Vars"=w1779, "Error In"=w1776, "FunctDataMgr in"=w1788) -> ("FunctDataMgr out"=w1787:refnum<class "FunctDataMgr.lvclass">)  [unwired: 8 in]
                  n851 = Bundle By Name(cluster=w1786, "FunctData"=w1787) -> (w1785:T36)
                }
                frame "CheckUutEnumStatus" {
                  n852 = Unbundle By Name(w1800) -> ("Child Modules"=w1799:cluster{"Name":string, "vi ref":refnum<vi>}[])
                  n853 = local read "Timeout(s)"() -> (w1802:dbl)
                  n854 = Index Array(array=w1799) -> (element=w1798:cluster{"Name":string, "vi ref":refnum<vi>})  [unwired: 1 in]
                  n855 = Unbundle By Name(w1798) -> ("Name"=w1797:string)
                  n856 = Multiply(x=w1802, y=1000.0 ("x")) -> (x*y=w1805:dbl)
                  n857 = To Long Integer(number=w1805) -> (32bit integer=w1804:i32)
                  n858 = call <vilib>:"Q.Send Function Command and wait on Ret Data.vi"("Timeout(ms)"=w1804, "Q Name"=w1797, "Data1"=w1795, "Cmd"="GetEnumStatus", "Q In"=w1796) -> ("error out"=w1794:errorcluster, "Ret"=w1808:variant)  [unwired: 5 in]
                  n859 = Variant To Data(type=string[][] [], Variant=w1808) -> (data=w1806:string[][], error out=w1807:errorcluster)  [unwired: 1 in]
                  n860 = case shown="No Error" w1807 {
                    tunnel: w1806 -> [w1814 _]
                    tunnel: [w1814 _] -> w1793
                    frame No Error {
                    }
                    frame Error {
                    }
                  }
                  n861 = call "Hmd.Check RtnVars for Enumerated Status.vi"("Vars"=w1793) -> ("Enumerated"=→"Enumerated":bool)  [unwired: 2 in]
                  n862 = Unbundle By Name(w1811) -> ("FunctData"=w1813:refnum<class "FunctDataMgr.lvclass">)
                  n863 = call "FunctDataMgr.Function Add RTN Data.vi"("Vars"=w1793, "Error In"=w1794, "FunctDataMgr in"=w1813) -> ("FunctDataMgr out"=w1812:refnum<class "FunctDataMgr.lvclass">)  [unwired: 8 in]
                  n864 = Bundle By Name(cluster=w1811, "FunctData"=w1812) -> (w1810:T36)
                }
                frame "Archive_Results" {
                  n865 = Unbundle By Name(w1825) -> ("Dirs.UUTDir"=w1824:path, "Dirs.Archive"=w1823:path, "ResultState.State"=w1817:T34)
                  n866 = Variant To Data(type=string[] [], Variant=w1819) -> (data=w1820:string[], error out=w1821:errorcluster)  [unwired: 1 in]
                  n867 = case shown="No Error" w1821 {
                    tunnel: w1820 -> [w1830 _]
                    tunnel: [w1830 _] -> w1818
                    frame No Error {
                    }
                    frame Error {
                    }
                  }
                  n868 = case shown="\"Failing\", \"FAIL\"" w1817 {
                    tunnel: [_ " - FAIL" " - ERROR" " - ABORT"] -> w1816
                    frame "None", Default {
                    }
                    frame "Failing", "FAIL" {
                      (unwired) TRUE
                    }
                    frame "ERROR" {
                    }
                    frame "ABORT" {
                      (unwired) TRUE
                    }
                  }
                  n869 = call "File.Move to Archive Folder.vi"("NameSuffix"=w1816, "SubDirList"=w1818, "ArchiveDir"=w1823, "UUTDir"=w1824) -> ("error out"=w1815:errorcluster)  [unwired: 6 in, 1 out]
                }
                frame "Archive_SummaryResults" {
                  n870 = Unbundle By Name(w1836) -> ("Dirs.UUTDir"=w1833:path, "Dirs.ArchiveSum"=w1837:path)
                  n871 = call <vilib>:"File.Check if File or Folder Exists.vi"("Path"=w1833) -> ("Exists"=w1831:bool, "Dup Path"=w1832:path)  [unwired: 6 in, 3 out]
                  n872 = case shown="True" w1831 {
                    tunnel: w1837 -> [_ w1841]
                    tunnel: w1835 -> [_ w1850]
                    tunnel: w1832 -> [_ w1849]
                    tunnel: [_ w1843] -> w1834
                    frame False {
                    }
                    frame True {
                      w1847 = T37 -5200 items=["No Error"=0, "Abort"=-2, "Misc"=-5000, "Fixture Error"=-5100, "File IO - General"=-5200, "FIle IO - Config Error"=-5201, "Instrument - General"=-5300, "Instrument - Serial Com"=-5301, "Instrument - Camera"=-5302, "Instrument - PS"=-5303, "Instrument - Oscilloscope"=-5304, "Instrument - Function Gen"=-5305, "Instrument - Load"=-5306, "Instrument - Meter"=-5307, "Instrument - Power Control"=-5308, "Instrument - Motion"=-5309, "Instrument - RF"=-5310, "System Exe"=-5400, "Image Processing"=-5500, "Communication"=-5600, "Script - Syntax Error"=-6000, "Script - Invalid Name or Param"=-6100, "Script - Timeout"=-6200, "Invalid Data"=-6300, "FW Update Error"=-6500] ("Std Code")
                      # "Need to separate adn group data to summary results if applicable."
                      n873 = Variant To Data(type=string[] [], Variant=w1850) -> (data=w1851:string[], error out=w1852:errorcluster)  [unwired: 1 in]
                      n874 = case shown="No Error" w1852 {
                        tunnel: w1851 -> [w1854 _]
                        tunnel: [w1854 _] -> w1840
                        frame No Error {
                        }
                        frame Error {
                        }
                      }
                      n875 = call "File.Build Path, Add Multiple Subfolders, Check for invalid Characters.vi"("Check/Create Dir"=TRUE, "Subfolders"=w1840, "Folder"=w1841) -> ("New Path"=w1839:path)  [unwired: 6 in, 2 out]
                      n876 = call <vilib>:"File.Create Folder if Does Not Exist.vi"("Path"=w1839) -> ("Dup Path"=w1845:path)  [unwired: 8 in, 2 out]
                      n877 = Move(source path=w1849, 10:w1845) -> (error out=w1848:errorcluster)  [unwired: 3 in, 2 out]
                      n878 = Format Into String(format string="Error archiving data.| Destination folder: \"%s\".", w1845) -> (resulting string=w1844:string)  [unwired: 2 in, 1 out]
                      n879 = call "Error.Set-Change Error Info.vi"("Std Code"=w1847, "error in"=w1848, "Description"=w1844) -> ("error out"=w1843:errorcluster)  [unwired: 8 in]
                    }
                  }
                }
                frame Default {
                  n880 = To Upper Case(1:w1863) -> (0:w1862:string)
                  n881 = Match Pattern(string=w1862, regular expression="^HMD\\.") -> (after substring=w1859:string, offset past match=w1861:i32)  [unwired: 1 in, 2 out]
                  n882 = Greater Or Equal To 0?(x=w1861) -> (x >= 0?=w1860:bool)
                  n883 = case shown="True" w1860 {
                    tunnel: [w1873 w1880] -> w1867
                    tunnel: w1866 -> [w1873 w1881]
                    tunnel: [w1872 w1884] -> w1865
                    tunnel: w1863 -> [w1868 _]
                    tunnel: w1859 -> [_ w1886]
                    tunnel: w1858 -> [_ w1895]
                    tunnel: w1857 -> [_ w1888]
                    tunnel: w1856 -> [_ w1885]
                    frame False {
                      w1871 = T37 -6100 items=["No Error"=0, "Abort"=-2, "Misc"=-5000, "Fixture Error"=-5100, "File IO - General"=-5200, "FIle IO - Config Error"=-5201, "Instrument - General"=-5300, "Instrument - Serial Com"=-5301, "Instrument - Camera"=-5302, "Instrument - PS"=-5303, "Instrument - Oscilloscope"=-5304, "Instrument - Function Gen"=-5305, "Instrument - Load"=-5306, "Instrument - Meter"=-5307, "Instrument - Power Control"=-5308, "Instrument - Motion"=-5309, "Instrument - RF"=-5310, "System Exe"=-5400, "Image Processing"=-5500, "Communication"=-5600, "Script - Syntax Error"=-6000, "Script - Invalid Name or Param"=-6100, "Script - Timeout"=-6200, "Invalid Data"=-6300, "FW Update Error"=-6500] ("Std Code")
                      n884 = Format Into String(format string="Unknown Function \"%s\".", w1868) -> (resulting string=w1869:string)  [unwired: 2 in, 1 out]
                      n885 = call "Error.Set-Change Error Info.vi"("Std Code"=w1871, "Description"=w1869, "Set Error"=TRUE) -> ("error out"=w1872:errorcluster)  [unwired: 8 in]
                    }
                    frame True {
                      # "Child modules return only variables and error."
                      n886 = Unbundle By Name(w1895) -> ("Child Modules"=w1894:cluster{"Name":string, "vi ref":refnum<vi>}[])
                      n887 = Unbundle By Name(w1881) -> ("Timeout(s)"=w1892:dbl)
                      n888 = Multiply(x=w1892, y=1000.0) -> (x*y=w1890:dbl)
                      n889 = Index Array(array=w1894) -> (element=w1893:cluster{"Name":string, "vi ref":refnum<vi>})  [unwired: 1 in]
                      n890 = To Long Integer(number=w1890) -> (32bit integer=w1889:i32)
                      n891 = Unbundle By Name(w1893) -> ("Name"=w1887:string)
                      n892 = call <vilib>:"Q.Send Function Command and wait on Ret Data.vi"("Timeout(ms)"=w1889, "Q Name"=w1887, "Data1"=w1885, "Cmd"=w1886, "Q In"=w1888) -> ("error out"=w1884:errorcluster, "Ret"=w1876:variant)  [unwired: 5 in]
                      n893 = Variant To Data(type=string[][] [], Variant=w1876) -> (data=w1877:string[][], error out=w1878:errorcluster)  [unwired: 1 in]
                      n894 = Unbundle By Name(w1881) -> ("FunctData"=w1883:refnum<class "FunctDataMgr.lvclass">)
                      n895 = case shown="Error" w1878 {
                        tunnel: w1877 -> [w1896 _]
                        tunnel: [w1896 _] -> w1875
                        frame No Error {
                        }
                        frame Error {
                        }
                      }
                      n896 = call "FunctDataMgr.Function Add RTN Data.vi"("Vars"=w1875, "FunctDataMgr in"=w1883) -> ("FunctDataMgr out"=w1882:refnum<class "FunctDataMgr.lvclass">)  [unwired: 9 in]
                      n897 = Bundle By Name(cluster=w1881, "FunctData"=w1882) -> (w1880:T36)
                    }
                  }
                }
              }
            }
            frame Default {
              # "Return"
              n898 = case shown="False" w1898 {
                tunnel: w1902 -> [w1909 w1911]
                tunnel: [w1908 w1912] -> w1901
                tunnel: [w1906 _] -> w1900
                tunnel: w1899 -> [w1905 w1913]
                tunnel: w1897 -> [_ _]
                frame False {
                  n899 = Unbundle By Name(w1909) -> ("FunctData"=w1910:refnum<class "FunctDataMgr.lvclass">)
                  n900 = call "FunctDataMgr.Function Return.vi"("Error In"=w1905, "FunctDataMgr in"=w1910) -> ("Error Out"=w1906:errorcluster, "FunctDataMgr out"=w1907:refnum<class "FunctDataMgr.lvclass">)  [unwired: 8 in]
                  n901 = Bundle By Name(cluster=w1909, "FunctData"=w1907) -> (w1908:T36)
                }
                frame True {
                  # "In case, record error.\n\nThis case is reached when a function is set to retrn later (after some tasks have been performed.\nThat function(or one of its tasks) is responsible for enquing the 'Funct RTN' task."
                  n902 = Unbundle By Name(w1911) -> ("FunctData"=w1915:refnum<class "FunctDataMgr.lvclass">)
                  n903 = call "FunctDataMgr.Function Add RTN Data.vi"("Error In"=w1913, "FunctDataMgr in"=w1915) -> ("FunctDataMgr out"=w1914:refnum<class "FunctDataMgr.lvclass">)  [unwired: 9 in]
                  n904 = Bundle By Name(cluster=w1911, "FunctData"=w1914) -> (w1912:T36)
                }
              }
            }
          }
        }
      }
      frame "App" {
        n905 = case shown="\"Set Logging Level\"" w1923 {
          tunnel: w1922 -> [_ _ w1945 _]
          tunnel: w1921 -> [_ w1926 _ w1957]
          tunnel: w1920 -> [_ _ _ _]
          tunnel: w1919 -> [w1925 w1931 w1950 w1960]
          tunnel: w1918 -> [w1924 w1930 w1949 w1958]
          tunnel: [w1925 w1931 w1950 w1953] -> w1917
          tunnel: [w1924 w1930 w1949 w1958] -> w1916
          frame Default {
          }
          frame "Lock Test Controls" {
            n906 = Variant To Data(type=FALSE, Variant=w1926) -> (data=w1928:bool, error out=w1929:errorcluster)  [unwired: 1 in]
            n907 = case shown="No Error" w1929 {
              selector: w1929 -> [_ w1943]
              tunnel: w1928 -> [w1936 _]
              tunnel: [_ w1943] -> _
              frame No Error {
                n908 = case shown="True" w1936 {
                  tunnel: [T19."Enabled" ("Disabled") T19."Disabled and Grayed Out" ("Disabled")] -> w1932
                  tunnel: [T19."Enabled" ("Disabled") T19."Disabled" ("Disabled")] -> _
                  tunnel: [TRUE ("Enable") FALSE ("Enable")] -> w1933
                  frame False {
                  }
                  frame True {
                  }
                }
                n909 = Current VI's Menubar() -> (w1934:refnum<k9>)
                n910 = call <vilib>:"Menu.Enable Item.vi"("Enable"=w1933, "Tag"="Config", "Menu Ref"=w1934) -> ()  [unwired: 7 in, 2 out]
                n911 = property on="Mode" class="Str"("DisabledEnum"=w1932) -> ()  [unwired: 2 in, 2 out]
                n912 = property on="SN" class="Str"("DisabledEnum"=w1932) -> ()  [unwired: 2 in, 2 out]
                n913 = property on="Get Top SN" class="Bool"("DisabledEnum"=w1932) -> ()  [unwired: 2 in, 2 out]
                n914 = property on="Archive Results" class="Bool"("DisabledEnum"=w1932) -> ()  [unwired: 2 in, 2 out]
                n915 = property on="Init UUT Folder" class="Bool"("DisabledEnum"=w1932) -> ()  [unwired: 2 in, 2 out]
                n916 = property on="Run Sweep" class="Bool"("DisabledEnum"=w1932) -> ()  [unwired: 2 in, 2 out]
                n917 = property on="Check UUT Enum Status" class="Bool"("DisabledEnum"=w1932) -> ()  [unwired: 2 in, 2 out]
              }
              frame Error {
              }
            }
          }
          frame "Initialization Done" {
            n918 = To Variant(anything=FALSE) -> (Variant=w1947:variant)
            n919 = call <vilib>:"Q.Enqueue App.vi"("Data1"=w1947, "Task Name"="Lock Test Controls", "Q In"=w1945) -> ()  [unwired: 7 in, 2 out]
            n920 = local write "Status"("Idle") -> ()
          }
          frame "Set Logging Level" {
            n921 = Variant To Data(type=Event_Log.Log_Level."Normal" ("Logging Level"), Variant=w1957) -> (data=w1951:T8)  [unwired: 1 in, 1 out]
            n922 = local read "Logging Level"() -> (w1954:T8)
            n923 = Unbundle By Name(w1960) -> ("Log"=w1959:refnum<class "Event Notification.lvclass">)
            n924 = call <vilib>:"Event Notification.Set Logging Level.vi"("Log Level"=w1951, "Event Notification in"=w1959) -> ("Event Notification out"=w1961:refnum<class "Event Notification.lvclass">)  [unwired: 9 in]
            n925 = Not Equal?(x=w1951, y=w1954) -> (x != y?=w1955:bool)
            n926 = case shown="True" w1955 {
              tunnel: w1951 -> [_ w1967]
              frame False {
              }
              frame True {
                n927 = local write "Logging Level"(w1967) -> ()
              }
            }
            n928 = Bundle By Name(cluster=w1960, "Log"=w1961) -> (w1953:T13)
            n929 = Unbundle By Name(w1953) -> ("Child Modules"=w1952:cluster{"Name":string, "vi ref":refnum<vi>}[])
            n930 = for {
              tunnel: w1952 -> [w1966] mode=indexing
              tunnel: w1951 -> [w1962]
              n931 = Unbundle By Name(w1966) -> ("Name"=w1963:string)
              n932 = To Variant(anything=w1962) -> (Variant=w1964:variant)
              n933 = call <vilib>:"Q.Enqueue App.vi"("Data1"=w1964, "Q Name"=w1963, "Task Name"="Set Logging Level") -> ()  [unwired: 7 in, 2 out]
            }
          }
        }
      }
      frame "Error", Default {
        n934 = case shown="\"Error\"" w1970 {
          selector: w1970 -> [_ w2015]
          tunnel: [_ w2016] -> w1973
          tunnel: w1968 -> [w1985 _]
          tunnel: w1969 -> [w1983 _]
          tunnel: w1971 -> [w1984 _]
          tunnel: w1972 -> [w1982 _]
          tunnel: w1976 -> [w1979 w2014]
          tunnel: w1975 -> [w1980 _]
          tunnel: [w1978 w2014] -> w1974
          frame "Error" {
            n935 = case shown="Default" w1984 {
              tunnel: w1985 -> [_ w2012 _]
              tunnel: w1983 -> [w2008 _ _]
              tunnel: [w2008 w2010 _] -> w1977
              tunnel: w1982 -> [w2007 w2009 w2013]
              tunnel: [w2007 w2009 w2013] -> w1981
              frame Default {
              }
              frame "Error" {
                n936 = Variant To Data(type=errorcluster {"status"=FALSE, "code"=0, "source"=""} ("error constant"), Variant=w2012) -> (data=w2010:errorcluster)  [unwired: 1 in, 1 out]
              }
              frame "Clear" {
              }
            }
            n937 = case shown="Error" w1977 {
              selector: w1977 -> [_ w1997]
              tunnel: w1981 -> [_ _]
              tunnel: w1980 -> [w1989 w2002]
              tunnel: w1979 -> [w1987 w1998]
              tunnel: [w1987 w1998] -> w1978
              frame No Error {
                # "Clear Local Errors"
                n938 = local read "Error"() -> (w1986:errorcluster)
                n939 = Unbundle By Name(w1989) -> ("Log"=w1988:refnum<class "Event Notification.lvclass">)
                n940 = case shown="Error" w1986 {
                  tunnel: w1988 -> [_ w1994]
                  frame No Error {
                  }
                  frame Error {
                    n941 = invoke on="Error" class="Clust (strict)" method="Reinit To Default"() -> ()  [unwired: 3 in, 3 out]
                    n942 = call <vilib>:"Event Notification.Status Message.vi"("Log"=TRUE, "Level"=Event_Log.Log_Level."Verbose", "Message"="Cleared Errors", "Event Notification in"=w1994) -> ()  [unwired: 8 in]
                  }
                }
                n943 = control-ref of="Error Status"() -> (w1990:refnum<vi>)
                n944 = call <vilib>:"Status.Simple Text Status Indicator.vi"("Status TextBox"=w1990) -> ()  [unwired: 10 in, 1 out]
              }
              frame Error {
                # "Record Error"
                n945 = Unbundle By Name(w2002) -> ("Log"=w2001:refnum<class "Event Notification.lvclass">)
                n946 = call "Error.Remove Trace Info form Error Desc.vi"("error in"=w1997, "Leave In Trace Info"="AddTraceInfo") -> ("error out"=w1996:errorcluster)  [unwired: 9 in]
                "Error" <- w1996
                n947 = Unbundle By Name(w1996) -> ("code"=w2005:i32, "source"=w2004:string)
                n948 = Format Into String(format string="ERROR!!! Code: %d, Desc: %s", w2005, w2004) -> (resulting string=w2000:string)  [unwired: 2 in, 1 out]
                n949 = control-ref of="Error Status"() -> (w2003:refnum<vi>)
                n950 = call <vilib>:"Event Notification.Status Message with Error In.vi"("Type"=Event_Log.Notification_Type."Error", "Message"=w2000, "Event Notification in"=w2001) -> ()  [unwired: 9 in]
                n951 = call <vilib>:"Status.Simple Text Status Indicator.vi"("error in"=w1996, "Status TextBox"=w2003) -> ()  [unwired: 9 in, 1 out]
              }
            }
          }
          frame Default {
            n952 = Concatenate Strings("Undefined State: \"", w2015, "\".") -> (w2017:string)
            n953 = Bundle By Name(cluster=errorcluster {"status"=TRUE, "code"=-5000, "source"=""} ("error constant"), "source"=w2017) -> (w2016:errorcluster)
          }
        }
      }
      frame "Exit" {
        # "This connection is made to not close\n the module until exit tasks are done."
        n954 = stacked-sequence {
          tunnel: w2025 -> [_ _ _]
          tunnel: [errorcluster {"status"=FALSE, "code"=0, "source"=""} ("error constant") _ _] -> w2024
          tunnel: [_ w2036 _] -> _
          tunnel: [_ w2034 _] -> _
          tunnel: w2021 -> [w2029 _ _]
          frame #0 {
            # "Close connection to instruments"
            n955 = Unbundle By Name(w2029) -> ("Child Modules"=w2028:cluster{"Name":string, "vi ref":refnum<vi>}[])
            n956 = for {
              tunnel: w2028 -> [w2033] mode=indexing
              tunnel: [w2031] -> _ mode=indexing
              n957 = Unbundle By Name(w2033) -> ("Name"=w2032:string)
              n958 = call <vilib>:"Q.Enqueue Exit.vi"("Q Name"=w2032) -> ("error out"=w2031:errorcluster)  [unwired: 9 in, 1 out]
            }
          }
          frame #1 {
            n959 = call <vilib>:"Q.Enqueue Exit.vi"("Q Name"="Graphs" ("Control Q")) -> ("error out"=w2034:errorcluster)  [unwired: 9 in, 1 out]
            n960 = call <vilib>:"Q.Enqueue Exit.vi"("Q Name"="TCP-IP_Bridge" ("Control Q")) -> ("error out"=w2036:errorcluster)  [unwired: 9 in, 1 out]
          }
          frame #2 {
            # "Store colors so when app reopens will restore"
            n961 = property on="L AvgMagUnCov" class="DigNum (strict)"() -> ("NumText.BGColor"=→"L Level Color":u32)  [unwired: 2 in, 2 out]
            n962 = property on="R AvgMagUnCov" class="DigNum (strict)"() -> ("NumText.BGColor"=→"R Level Color":u32)  [unwired: 2 in, 2 out]
            n963 = property on="R AvgMag Delta" class="DigNum (strict)"() -> ("NumText.BGColor"=→"R Delta Color":u32)  [unwired: 2 in, 2 out]
            n964 = property on="L AvgMag Delta" class="DigNum (strict)"() -> ("NumText.BGColor"=→"L Delta Color":u32)  [unwired: 2 in, 2 out]
          }
        }
        n965 = Bundle By Name(cluster=w2021, "Cfg.Is Child?"=FALSE) -> (w2022:T13)
        n966 = call <vilib>:"Module.Destructor.vi"("error in"=w2024, "Sys"=w2022) -> ("error out"=w2027:errorcluster)  [unwired: 9 in]
      }
    }
  }
  n967 = while "Event Loop" {
    tunnel: w6 -> [w2045]
    stop <- w2046 stop-if-true
    n968 = Unbundle By Name(w2045) -> ("Stop.Ref"=w2044:refnum<event-registration>, "Main Q"=w2043:refnum<queue>)
    n969 = event shown="[16] \"Play Tone\": Value Change" {
      selector: w2044 -> [_ _ _ _ _ _ _ _ _ _ _ _ _ _ _ _ _ _ _ _ _ _ _ _ _ _ _ _ _]
      dyn-events: _ -> [_ _ _ _ _ _ _ _ _ _ _ _ _ _ _ _ _ _ _ _ _ _ _ _ _ _ _ _ _]
      timeout: 1000 -> [_ _ _ _ _ _ _ _ _ _ _ _ _ _ _ _ _ _ _ _ _ _ _ _ _ _ _ _ _]
      tunnel: [w2049 TRUE w2065 _ _ _ _ _ _ _ _ _ _ _ _ _ _ _ _ _ _ _ _ _ _ _ _ _ _] -> w2046
      tunnel: w2045 -> [w2048 _ w2063 _ _ _ _ _ _ _ _ _ _ _ _ _ _ _ _ _ _ _ _ _ _ _ _ _ _]
      tunnel: w2043 -> [w2051 _ w2064 w2088 _ _ w2098 w2102 w2108 w2110 w2116 w2121 w2126 w2146 w2161 w2168 w2171 w2174 w2177 w2179 w2181 w2183 _ w2186 w2190 w2192 w2194 _ w2200]
      event Panel Close? {
        n970 = event-data() -> ()  [unwired: 1 in, 4 out]
        n971 = Unbundle By Name(w2048) -> ("Cfg.Is Child?"=w2047:bool)
        n972 = case shown="True" w2047 {
          tunnel: w2051 -> [w2054 w2057]
          tunnel: [TRUE TRUE] -> w2050
          tunnel: [TRUE FALSE] -> w2049
          tunnel: [_ w2055] -> _
          frame False {
            # "Parent - Exit"
            n973 = call <vilib>:"Q.Enqueue Exit.vi"("Q In"=w2054) -> ()  [unwired: 9 in, 2 out]
          }
          frame True {
            # "Child - Hide Panel and if was \nin a subpanel, return to subpanel."
            n974 = call <vilib>:"Module.Window, Q Task.vi"("Action"=Window.Task,_Action."Return to SubPanel()", "Q In"=w2057) -> ("error out"=w2055:errorcluster)  [unwired: 8 in, 1 out]
          }
        }
        n975 = event-data("Discard?"=w2050) -> ()  [unwired: 1 in, 1 out]
      }
      event User Event {
        n976 = event-data() -> ()  [unwired: 1 in, 5 out]
      }
      event Menu Selection (User) {
        n977 = event-data() -> ("MenuRef"=w2061:refnum<k9>, "ItemTag"=w2062:string)  [unwired: 1 in, 5 out]
        n978 = case shown="\"Help.About\"" w2062 {
          selector: w2062 -> [w2067 _ _ _ _ w2077 _ _]
          tunnel: [_ TRUE _ _ _ _ _ _] -> w2065
          tunnel: w2064 -> [_ w2070 _ w2073 _ w2081 w2083 w2086]
          tunnel: [_ _ w2072 _ _ _ _ _] -> _
          tunnel: w2063 -> [w2066 _ _ _ w2075 _ _ _]
          tunnel: w2061 -> [_ _ _ _ _ w2078 _ _]
          frame Default {
            # "Check if a help document was selected.\nIf so, open the document"
            n979 = Unbundle By Name(w2066) -> ("Docs.Tags"=w2069:string[], "Docs.Paths"=w2068:path[])
            n980 = call <vilib>:"Menu.Help, Open User Manual Items.vi"("Menu Tag Selection"=w2067, "Paths"=w2068, "Tags"=w2069) -> ()  [unwired: 8 in, 1 out]
          }
          frame "Exit" {
            n981 = call <vilib>:"Q.Enqueue Exit.vi"("Q In"=w2070) -> ()  [unwired: 9 in, 2 out]
          }
          frame "Event Log" {
            n982 = call <vilib>:"Event Log.Show.vi"() -> ("error out"=w2072:errorcluster)  [unwired: 11 in]
          }
          frame "Reset" {
            n983 = call <vilib>:"Q.Enqueue Reset.vi"("Q In"=w2073) -> ()  [unwired: 9 in, 2 out]
          }
          frame "Help.About" {
            n984 = Unbundle By Name(w2075) -> ("SW Rev"=w2074:T12)
            n985 = call <vilib>:"Help.About.vi"("SW Version"=w2074) -> ()  [unwired: 11 in]
          }
          frame "Simulate OFF", "Simulate ON" {
            n986 = call <vilib>:"Menu.Simulate, Set Menu State.vi"("Menu Tag"=w2077, "Menu Ref"=w2078) -> ("Sim ON"=w2076:bool)  [unwired: 8 in, 1 out]
            n987 = To Variant(anything=w2076) -> (Variant=w2080:variant)
            n988 = call <vilib>:"Q.Enqueue Task.vi"("Data1"=w2080, "Task Name"="Simulate", "Q In"=w2081) -> ()  [unwired: 7 in, 2 out]
          }
          frame "Show Block Diagram" {
            n989 = call <vilib>:"Module.Window, Q Task.vi"("Action"=Window.Task,_Action."Open Block Diagram()", "Q In"=w2083) -> ()  [unwired: 8 in, 2 out]
          }
          frame "Go to Maint Tab" {
            n990 = call <vilib>:"Module.Window, Q Task.vi"("Show"=TRUE, "Action"=Window.Task,_Action."Go To Maint Tab()", "Q In"=w2086) -> ()  [unwired: 7 in, 2 out]
          }
        }
      }
      event Panel Resize {
        n991 = event-data() -> ()  [unwired: 1 in, 8 out]
        n992 = case shown="True" FALSE {
          tunnel: w2088 -> [_ w2090]
          frame False {
          }
          frame True {
            n993 = call <vilib>:"Module.Window, Q Task.vi"("Action"=Window.Task,_Action."Resize()", "Q In"=w2090) -> ()  [unwired: 8 in, 2 out]
          }
        }
      }
      event "Set Window Bounds": Value Change {
        n994 = event-data() -> ()  [unwired: 1 in, 6 out]
        n995 = control-ref of="This VI"() -> (w2093:refnum<vi>)
        n996 = property class="VI"(reference=w2093, "Front Panel.WinBounds"="New Window Bounds", "Front Panel.Resizeable"=TRUE ("Front Panel Window:Resizable")) -> ("Front Panel.PanelBounds"=→"Old Window Bounds":T11)  [unwired: 1 in, 2 out]
      }
      event "Leave Maint": Value Change {
        n997 = event-data() -> ()  [unwired: 1 in, 6 out]
        n998 = local write "Main Tab"(0) -> ()
      }
      event Value Change {
        n999 = event-data() -> ()  [unwired: 1 in, 6 out]
        n1000 = To Variant(anything="Logging Level") -> (Variant=w2097:variant)
        n1001 = call <vilib>:"Q.Enqueue App.vi"("Data1"=w2097, "Task Name"="Set Logging Level", "Q In"=w2098) -> ()  [unwired: 7 in, 2 out]
      }
      event "Abort": Value Change {
        n1002 = event-data() -> ()  [unwired: 1 in, 6 out]
        n1003 = call <vilib>:"Scheduler.Clear-Reset.vi"("Q In"=w2102) -> ("error out"=w2104:errorcluster, "Q Out"=w2103:refnum<queue>)  [unwired: 9 in]
        n1004 = Flush Queue(queue=w2103, error in (no error)=w2104) -> (queue out=w2101:refnum<queue>)  [unwired: 2 out]
        n1005 = call <vilib>:"Q.Enqueue Task.vi"("Task Name"="Test Abort", "Q In"=w2101) -> ()  [unwired: 8 in, 2 out]
        n1006 = for {
          N: 5 -> [_]
          n1007 = call "Abort.Send Abort or Done Notificaiton.vi"("Abort(T)/Done(F)"=TRUE) -> ()  [unwired: 10 in, 1 out]
          n1008 = Wait (ms)(milliseconds to wait=u32 10) -> ()  [unwired: 1 out]
        }
      }
      event "Test Reset": Value Change {
        n1009 = event-data() -> ()  [unwired: 1 in, 6 out]
        n1010 = call <vilib>:"Q.Enqueue Task.vi"("Task Name"="Test Reset", "Q In"=w2108) -> ()  [unwired: 8 in, 2 out]
      }
      event "Filter", "Show Only Failures": Value Change {
        n1011 = event-data() -> ()  [unwired: 1 in, 6 out]
        n1012 = call <vilib>:"Q.Enqueue Task.vi"("Task Name"="Update Results", "Q In"=w2110) -> ()  [unwired: 8 in, 2 out]
      }
      event "Get Top SN": Value Change {
        n1013 = event-data() -> ()  [unwired: 1 in, 6 out]
        n1014 = Build Array("GetUUTSN", "TopSN") -> (w2114:string[])
        n1015 = To Variant(anything=w2114) -> (Variant=w2115:variant)
        n1016 = call <vilib>:"Q.Enqueue Task.vi"("Data1"=w2115, "Task Name"="Funct Local Call", "Q In"=w2116) -> ()  [unwired: 7 in, 2 out]
      }
      event "Check UUT Enum Status": Value Change {
        n1017 = event-data() -> ()  [unwired: 1 in, 6 out]
        n1018 = Build Array("CheckUutEnumStatus") -> (w2119:string[])
        n1019 = To Variant(anything=w2119) -> (Variant=w2120:variant)
        n1020 = call <vilib>:"Q.Enqueue Task.vi"("Data1"=w2120, "Task Name"="Funct Local Call", "Q In"=w2121) -> ()  [unwired: 7 in, 2 out]
      }
      event "Run Sweep": Value Change {
        n1021 = event-data() -> ()  [unwired: 1 in, 6 out]
        n1022 = local read "Mic Test Setup"() -> (w2135:T3)
        n1023 = local read "UUT Dir"() -> (w2132:path)
        n1024 = call <vilib>:"File.Check if File or Folder Exists.vi"("Path"=w2132) -> ("Exists"=w2125:bool)  [unwired: 6 in, 4 out]
        n1025 = Unbundle By Name(w2135) -> ("Mic Side"=w2134:enum32{"LEFT", "RIGHT"}, "Covered"=w2133:bool)
        n1026 = case shown="True" w2125 {
          tunnel: [w2139 w2141] -> w2127
          tunnel: w2126 -> [w2138 w2141]
          frame False {
            n1027 = call <vilib>:"Q.Enqueue Task.vi"("Task Name"="Create_UUTFolder", "Q In"=w2138) -> ("Q Out"=w2139:refnum<queue>)  [unwired: 8 in, 1 out]
          }
          frame True {
          }
        }
        n1028 = case shown="\"LEFT\", Default" w2134 {
          tunnel: ["Left" "Right"] -> w2130
          frame "LEFT", Default {
          }
          frame "RIGHT" {
          }
        }
        n1029 = case shown="True" w2133 {
          tunnel: ["Uncovered" "Covered"] -> w2129
          frame False {
          }
          frame True {
          }
        }
        n1030 = Build Array("Sweep", w2130, w2129) -> (w2128:string[])
        n1031 = invoke on="Play Tone" class="Bool (strict)" method="Reinit To Default"() -> ()  [unwired: 3 in, 3 out]
        n1032 = To Variant(anything=w2128) -> (Variant=w2136:variant)
        n1033 = call <vilib>:"Q.Enqueue Task.vi"("Data1"=w2136, "Task Name"="MicrophoneTest", "Q In"=w2127) -> ("Q Out"=w2124:refnum<queue>)  [unwired: 7 in, 1 out]
        n1034 = call <vilib>:"Q.Enqueue Task.vi"("Task Name"="CL_Test_RTN", "Q In"=w2124) -> ()  [unwired: 8 in, 2 out]
      }
      event "Set Audio Output Device Name", "Set Audio Input Device Name": Value Change {
        n1035 = event-data() -> ()  [unwired: 1 in, 6 out]
        n1036 = stacked-sequence {
          tunnel: w2146 -> [_ w2156]
          frame #0 {
            n1037 = local read "Sound Devices"() -> (w2148:T6)
            n1038 = case shown="True" "Set Audio Input Device Name" {
              tunnel: w2148 -> [w2152 w2155]
              tunnel: [w2151 w2154] -> w2147
              frame True {
                n1039 = property on="Input Device" class="Ring (strict)"() -> ("RingText.Text"=w2150:string)  [unwired: 2 in, 2 out]
                n1040 = Bundle By Name(cluster=w2152, "AudioInName"=w2150) -> (w2151:T6)
              }
              frame False {
                n1041 = property on="Output Device" class="Ring (strict)"() -> ("RingText.Text"=w2153:string)  [unwired: 2 in, 2 out]
                n1042 = Bundle By Name(cluster=w2155, "AudioOutName"=w2153) -> (w2154:T6)
              }
            }
            n1043 = local write "Sound Devices"(w2147) -> ()
          }
          frame #1 {
            n1044 = call <vilib>:"Q.Enqueue Task.vi"("Task Name"="Config - Write", "Q In"=w2156) -> ()  [unwired: 8 in, 2 out]
          }
        }
      }
      event "Init UUT Folder": Value Change {
        n1045 = event-data() -> ()  [unwired: 1 in, 6 out]
        n1046 = Build Array("Create_UUTFolder") -> (w2158:string[])
        n1047 = To Variant(anything=w2158) -> (Variant=w2159:variant)
        n1048 = call <vilib>:"Q.Enqueue Task.vi"("Data1"=w2159, "Task Name"="Funct Local Call", "Q In"=w2161) -> ()  [unwired: 7 in, 2 out]
      }
      event "Archive Results": Value Change {
        n1049 = event-data() -> ()  [unwired: 1 in, 6 out]
        n1050 = call "File.Date String, File Safe.vi"() -> ("Date"=w2163:string)  [unwired: 3 in]
        n1051 = Build Array("Archive_Results", "Mode", w2163) -> (w2166:string[])
        n1052 = To Variant(anything=w2166) -> (Variant=w2167:variant)
        n1053 = call <vilib>:"Q.Enqueue Task.vi"("Data1"=w2167, "Task Name"="Funct Local Call", "Q In"=w2168) -> ()  [unwired: 7 in, 2 out]
      }
      event "Play Tone": Value Change {
        n1054 = event-data() -> ("NewVal"=w2170:bool)  [unwired: 1 in, 5 out]
        n1055 = case shown="True" w2170 {
          tunnel: w2171 -> [_ w2173]
          frame False {
          }
          frame True {
            n1056 = call <vilib>:"Q.Enqueue Task.vi"("Task Name"="Play Tone", "Q In"=w2173) -> ()  [unwired: 8 in, 2 out]
          }
        }
      }
      event "Reload Config": Value Change {
        n1057 = event-data() -> ()  [unwired: 1 in, 6 out]
        n1058 = call <vilib>:"Q.Enqueue Task.vi"("Task Name"="Config - Read", "Q In"=w2174) -> ()  [unwired: 8 in, 2 out]
      }
      event "Default Data Folder", "SpeakerCalFile", "Play Volume": Value Change {
        n1059 = event-data() -> ()  [unwired: 1 in, 6 out]
        n1060 = call <vilib>:"Q.Enqueue Task.vi"("Task Name"="Config - Write", "Q In"=w2177) -> ()  [unwired: 8 in, 2 out]
      }
      event "Clear Raw Data": Value Change {
        n1061 = event-data() -> ()  [unwired: 1 in, 6 out]
        n1062 = call <vilib>:"Q.Enqueue Task.vi"("Task Name"="Clear Raw Data", "Q In"=w2179) -> ()  [unwired: 8 in, 2 out]
      }
      event "Save Wav Files": Value Change {
        n1063 = event-data() -> ()  [unwired: 1 in, 6 out]
        n1064 = call <vilib>:"Q.Enqueue Task.vi"("Task Name"="Save Wav Files", "Q In"=w2181) -> ()  [unwired: 8 in, 2 out]
      }
      event "Clear Graphs": Value Change {
        n1065 = event-data() -> ()  [unwired: 1 in, 6 out]
        n1066 = call <vilib>:"Q.Enqueue Task.vi"("Task Name"="Clear Graphs", "Q In"=w2183) -> ()  [unwired: 8 in, 2 out]
      }
      event "Open UUT Dir": Value Change {
        n1067 = event-data() -> ()  [unwired: 1 in, 6 out]
        n1068 = local read "UUT Dir"() -> (w2185:path)
        n1069 = call <vilib>:"File.Open File or Folder.vi"("Path"=w2185) -> ("Error Out"=w2184:errorcluster)  [unwired: 10 in]
        n1070 = call <vilib>:"Clear Errors.vi"("error in (no error)"=w2184) -> ()  [unwired: 5 in, 2 out]
      }
      event "Clear Errors": Value Change {
        n1071 = event-data() -> ()  [unwired: 1 in, 6 out]
        n1072 = call "Error.Clear.vi"("Q In"=w2186) -> ()  [unwired: 9 in, 2 out]
      }
      event "SN": Value Change {
        n1073 = event-data() -> ()  [unwired: 1 in, 6 out]
        n1074 = To Variant(anything="SN") -> (Variant=w2187:variant)
        n1075 = call <vilib>:"Q.Enqueue Task.vi"("Data1"=w2187, "Task Name"="Update SN", "Q In"=w2190) -> ()  [unwired: 7 in, 2 out]
      }
      event "UUT Dir": Value Change {
        n1076 = event-data() -> ()  [unwired: 1 in, 6 out]
        n1077 = call <vilib>:"Q.Enqueue Task.vi"("Task Name"="Update UUT Folder", "Q In"=w2192) -> ()  [unwired: 8 in, 2 out]
      }
      event "Undock FW Util": Value Change {
        n1078 = event-data() -> ()  [unwired: 1 in, 6 out]
        n1079 = call <vilib>:"Q.Enqueue Task.vi"("Task Name"="HMD Module Undock", "Q In"=w2194) -> ()  [unwired: 8 in, 2 out]
      }
      event Timeout {
        n1080 = event-data() -> ()  [unwired: 1 in, 3 out]
        n1081 = local read "Test Running"() -> (w2195:bool)
        n1082 = case shown="True" w2195 {
          frame False {
          }
          frame True {
            n1083 = local read "Start Time"() -> (w2196:timestamp)
            n1084 = Get Date/Time In Seconds() -> (seconds since 1Jan1904=w2197:timestamp)
            n1085 = Subtract(x=w2197, y=w2196) -> (x-y=w2198:dbl)
            n1086 = local write "Duration(s)"(w2198) -> ()
          }
        }
      }
      event "Run CLI Simulation": Value Change {
        n1087 = event-data() -> ()  [unwired: 1 in, 6 out]
        n1088 = call "Error.Clear.vi"("Q In"=w2200) -> ("Q Out"=w2199:refnum<queue>)  [unwired: 9 in, 1 out]
        n1089 = call <vilib>:"Q.Enqueue Task.vi"("Task Name"="Run CLI Simulation", "Q In"=w2199) -> ()  [unwired: 8 in, 2 out]
      }
    }
  }
  n1090 = call <vilib>:"Time.Inline Calculate Duration Secs.vi"("Start(Sec)"=w1, "Error In Top"=w5) -> ("Duration(s)"=→"App Run Dur(s)":dbl)  [unwired: 7 in, 2 out]
  "Title" <- w8
